vi "Main_Marvin Remake.vi"() -> ()   [LabVIEW 2017]
uses:
  PCAN_Driver/ControlCAN.llb/DevType.ctl
  PCAN_Driver/ControlCAN.llb/CAN Channel.ctl
  PCAN_Driver/ControlCAN.llb/VCI_INIT_CONFIG.ctl
  PCAN_Driver/ControlCAN.llb/InitFlag.ctl
  PCAN_Driver/ControlCAN.llb/Fliter.ctl
  PCAN_Driver/ControlCAN.llb/Mode.ctl
  <vilib>/Utility/miscctls.llb/LVRowAndColumnTypeDef.ctl
  <vilib>/Utility/config.llb/Read Key (String).vi
  <vilib>/Utility/config.llb/Write Key (String).vi
  <vilib>/Utility/cursorutil.llb/Set Cursor (Icon Pict).vi
  PCAN_Driver/ControlCAN.lvlib
  <vilib>/Utility/config.llb/NI_LVConfig.lvlib
panel:
  in  "AD Resistor Step":dbl=9.0 format="%#_13g"
  out "ClosePanel":bool=TRUE
  out "UUT SN Report":string
  out "Automation":bool
  out "Test Failed":bool
  out "AuxiOFFResult":bool
  out "AuxiONResult":bool
  out "SensCalResult":bool
  out "VisualInspectionResult":bool
  out "BurnResult":bool
  out "BurnSpeed":bool
  out "BurnTemp":bool
  out "BurnDC":bool
  out "TempControlResult":bool
  out "MotorTempResult":bool
  out "StopTimeResult":bool
  out "SpeedResult":bool=TRUE
  out "VenableDirectionResult":bool
  out "VenableResult":bool
  out "ComTestResult":bool=TRUE
  out "UUT SoftwareVer":string
  out "Next SN":i32
  in  "SetSN":bool
  out "Current SN":i32
  out "Cal":dbl
  out "AO[1]Meas":dbl
  out "FullSpeed2 Speed":dbl
  out "FullSpeed2 Current":dbl
  out "FullSpeed1 Current":dbl
  out "FullSpeed1 Speed":dbl
  out "MaxBurnInTempVal":dbl
  in  "Stop Burn-in":bool
  out "VISA Tester":refnum<visa-resource-name>
  out "UUT":u8
  out "CAN Status":bool
  in  "Channel 2":T1 caption="Channel" items=["Channel 1", "Channel 2"]
  out "Config_CANAT":T7 {"DevType" items=["USB-CAN"=3, "USB-CAN2"=4]; "CanIndex" items=["通道1", "通道2"]; "VCI_INIT_CONFIG"."Fliter" items=["接收所有类型"=3, "只接收标准帧"=4, "只接收扩展帧"=7]; "VCI_INIT_CONFIG"."Mode" items=["正常工作", "自测模式（环回）", "仅侦听模式"]; "VCI_INIT_CONFIG"."InitFlag" items=["使用Flash参数", "使用界面设置参数"]}
  out "Array":u64[][](array[numeric]) format="%016x"
  out "Motor Phase Current RMS":dbl
  out "Ambient Temperature":dbl
  out "Speed error":bool
  out "Commutation err":bool
  out "Under voltage/Over voltage":bool
  out "Derated drive temp":bool
  out "Motor Over temperature":bool
  out "Motor Sensor temp Fauilre":bool
  out "Drive Over temperature":bool
  out "Drive Sensor temp Failure":bool
  out "Ambient Over temp":bool
  out "Ambient Sensor temp":bool
  out "DC Voltage":dbl
  out "DC Current":dbl
  out "Power transistor Heat sink Temp.":dbl
  out "Motor Stator Temp.":dbl
  out "Motor Speed RPM":dbl
  out "ECS State":u16
  out "UUT":string="EBAY"
  in  "Logger Path":path
  in  "Report":bool
  in  "Start":bool
  in  "ATR":string[][](table)=[["Test Communication", "-", "-", "-", "-", ""], ["Set S/N", "-", "-", "-", "-", ""], ["Set Board Number", "-", "-", "-", "-", ""], [" ", "", "", "", "", ""], ["Test Communication", "-", "-", "-", "-", ""], ["Get S/N", "-", "-", "-", "", ""], ["Get Board Number", "-", "-", "-", "", ""], ["Get FW", "-", "-", "-", "", ""], ["Enable Motor", "", "", "", "", ""], ["Small position command", "", "", "", "", ""], ["Measure delta", "", "", "", "", ""], ["Velocity command", "", "", "", "", ""]]
  in  "Settings":bool
  in  "Refresh Button":bool
  out "Status":bool
  in  "VISA Marvin":refnum<visa-resource-name>="COM6"
  in  "Serial Com":bool
  in  "Help Button":bool
  out "Pannel User Message":string
  in  "Stop Button":bool
  # "Marvin"
  # "REDLER TECHNOLOGIES LTD"
  # "ver 1.2n"
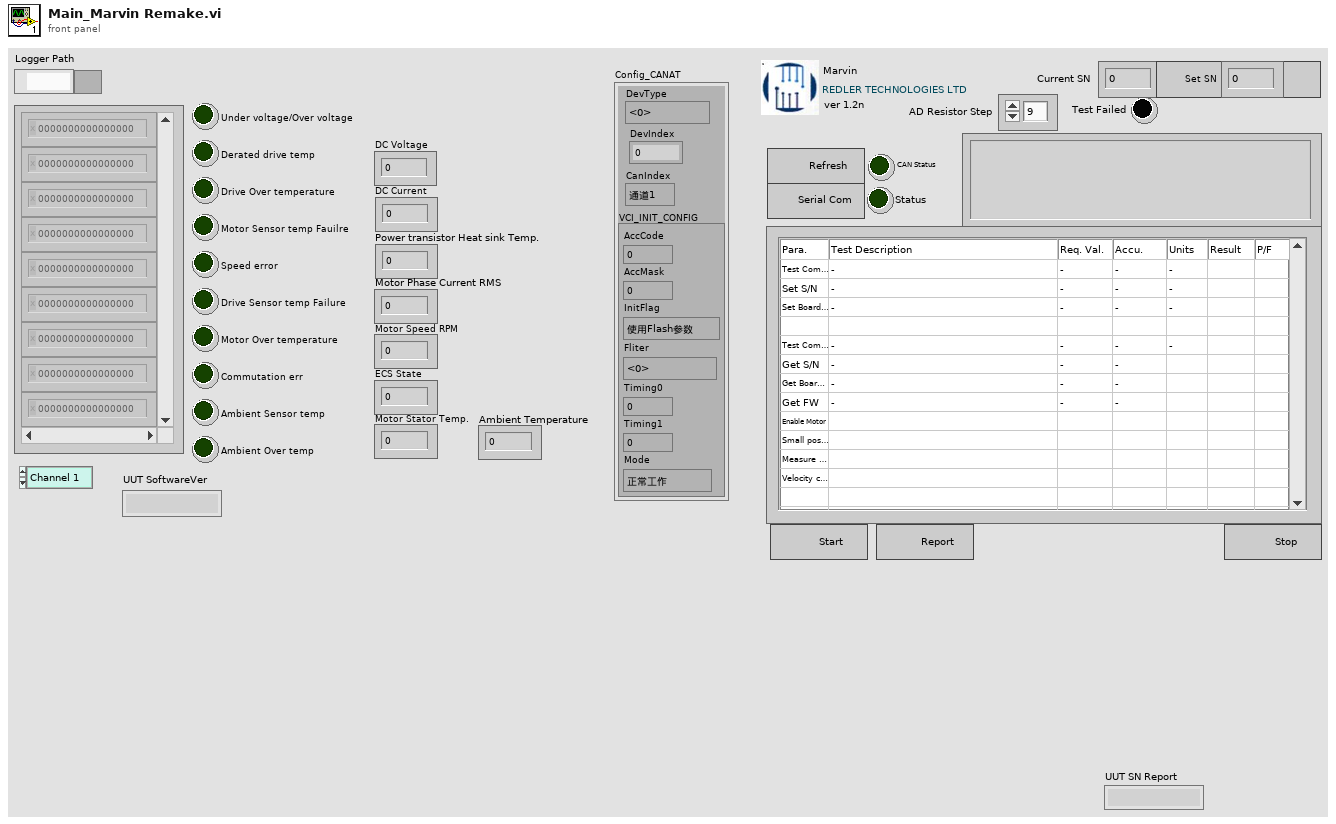
[diagram p1: front panel]
types:
  T1 = typedef "ControlCAN.lvlib/CAN Channel.ctl" = u32
  T2 = typedef "ControlCAN.lvlib/DevType.ctl" = u32
  T3 = typedef "ControlCAN.lvlib/VCI_INIT_CONFIG.ctl" = cluster{"AccCode":u32, "AccMask":u32, "InitFlag":T4, "Fliter":T5, "Timing0":u8, "Timing1":u8, "Mode":T6}
  T4 = typedef "ControlCAN.lvlib/InitFlag.ctl" = u32
  T5 = typedef "ControlCAN.lvlib/Fliter.ctl" = u8
  T6 = typedef "ControlCAN.lvlib/Mode.ctl" = u8
  T7 = cluster{"DevType":T2, "DevIndex":u32, "CanIndex":T1, "VCI_INIT_CONFIG":T3}
  T8 = cluster{"VISA":refnum<visa-resource-name>, "Array Test":enum16{"Auxiliary", "Temp Sens Cal", "Com Test", "Enable Test", "Speed Command", "Stop Time", "Temp Control", "Burn in", "Visual Inspec", "Empty"}[]}
  T9 = cluster{"ID":u32, "MSGTYPE":u8, "LEN":u8, "aDATA":u8[]}[]
  T10 = enum16{"Erase ATR Table", "Stop", "MainProgram", "Initialize"}
  T11 = enum16{"K15", "K16", "K17", "Venable", "Firmeware", "Fan", "Power", "120C", "110C", "100C", "90C", "80C", "70C", "60C", "50C", "40C", "30C", "25C", "20C", "10C", "0C"}
  T12 = enum16{"Stop", "Result", "FullSpeed2", "MD[1]=1", "FullSpeed1", "MD[1]=0"}
  T13 = enum8{"Term1", "Term2", "Current", "Fan", "TempCPU"}
  T14 = enum16{"Stop", "AO[1]=Meas.", "TA[5]", "AO[1]=0", "Start"}
  T15 = enum16{"Stop", "BurnIn", "Ambient Temp", "MotorSpeed", "DC Current Measure", "Start"}
  T16 = enum16{"Auxiliary", "Temp Sens Cal", "Com Test", "Enable Test", "Speed Command", "Stop Time", "Temp Control", "Burn in", "Visual Inspec", "Empty"}[]
  T17 = enum16{"K15", "K16", "K17", "Venable", "Firmeware", "Fan", "Power", "120C", "110C", "100C", "90C", "80C", "70C", "60C", "50C", "40C", "30C", "25C", "20C", "10C", "0C"}[]
  T18 = enum32{"6000", "11500", "15100", "11500-2", "6000-2"}[]
  T19 = enum8{"Enabled", "Disabled", "Disabled and Grayed Out"}
  T20 = typedef "LVRowAndColumnTypeDef.ctl" = cluster{"Row":i32, "Column":i32}
  T21 = enum32{"Invalid", "Standard", "Closed", "Hidden", "Minimized", "Maximized"}
  T22 = cluster{"ID":u32, "MSGTYPE":u8, "LEN":u8, "aDATA":u8[]}
  T23 = enum16{"Auxiliary", "Temp Sens Cal", "Com Test", "Enable Test", "Speed Command", "Stop Time", "Temp Control", "Burn in", "Visual Inspec", "Empty"}
  T24 = enum16{"open", "replace", "create", "open or create", "replace or create", "replace or create with confirmation"}
  T25 = typedef "NI_LVConfig.lvlib/Config Data RefNum.ctl" = refnum<k1>
  T26 = typedef "ControlCAN.lvlib/VCI_CAN_OBJ.ctl" = cluster{"ID":u32, "TimeStamp":u32, "TimeFlag":u8, "SendType":u8, "RemoteFlag":u8, "ExternFlag":u8, "DataLen":u8, "Data":u8[], "Reserved":u8[]}
  T27 = cluster{"Type":enum16{"接收", "发送"}, "Channel":T1, "Time":timestamp, "VCI_CAN_OBJ":T26}[]
  T28 = cluster{"Type":enum16{"接收", "发送"}, "Channel":T1, "Time":timestamp, "VCI_CAN_OBJ":T26}
  T29 = typedef "LVPoint32TypeDef.ctl" = cluster{"Horizontal":i32, "Vertical":i32}
  T30 = enum8{"Term1", "Term2", "Current", "Fan", "TempCPU"}[]
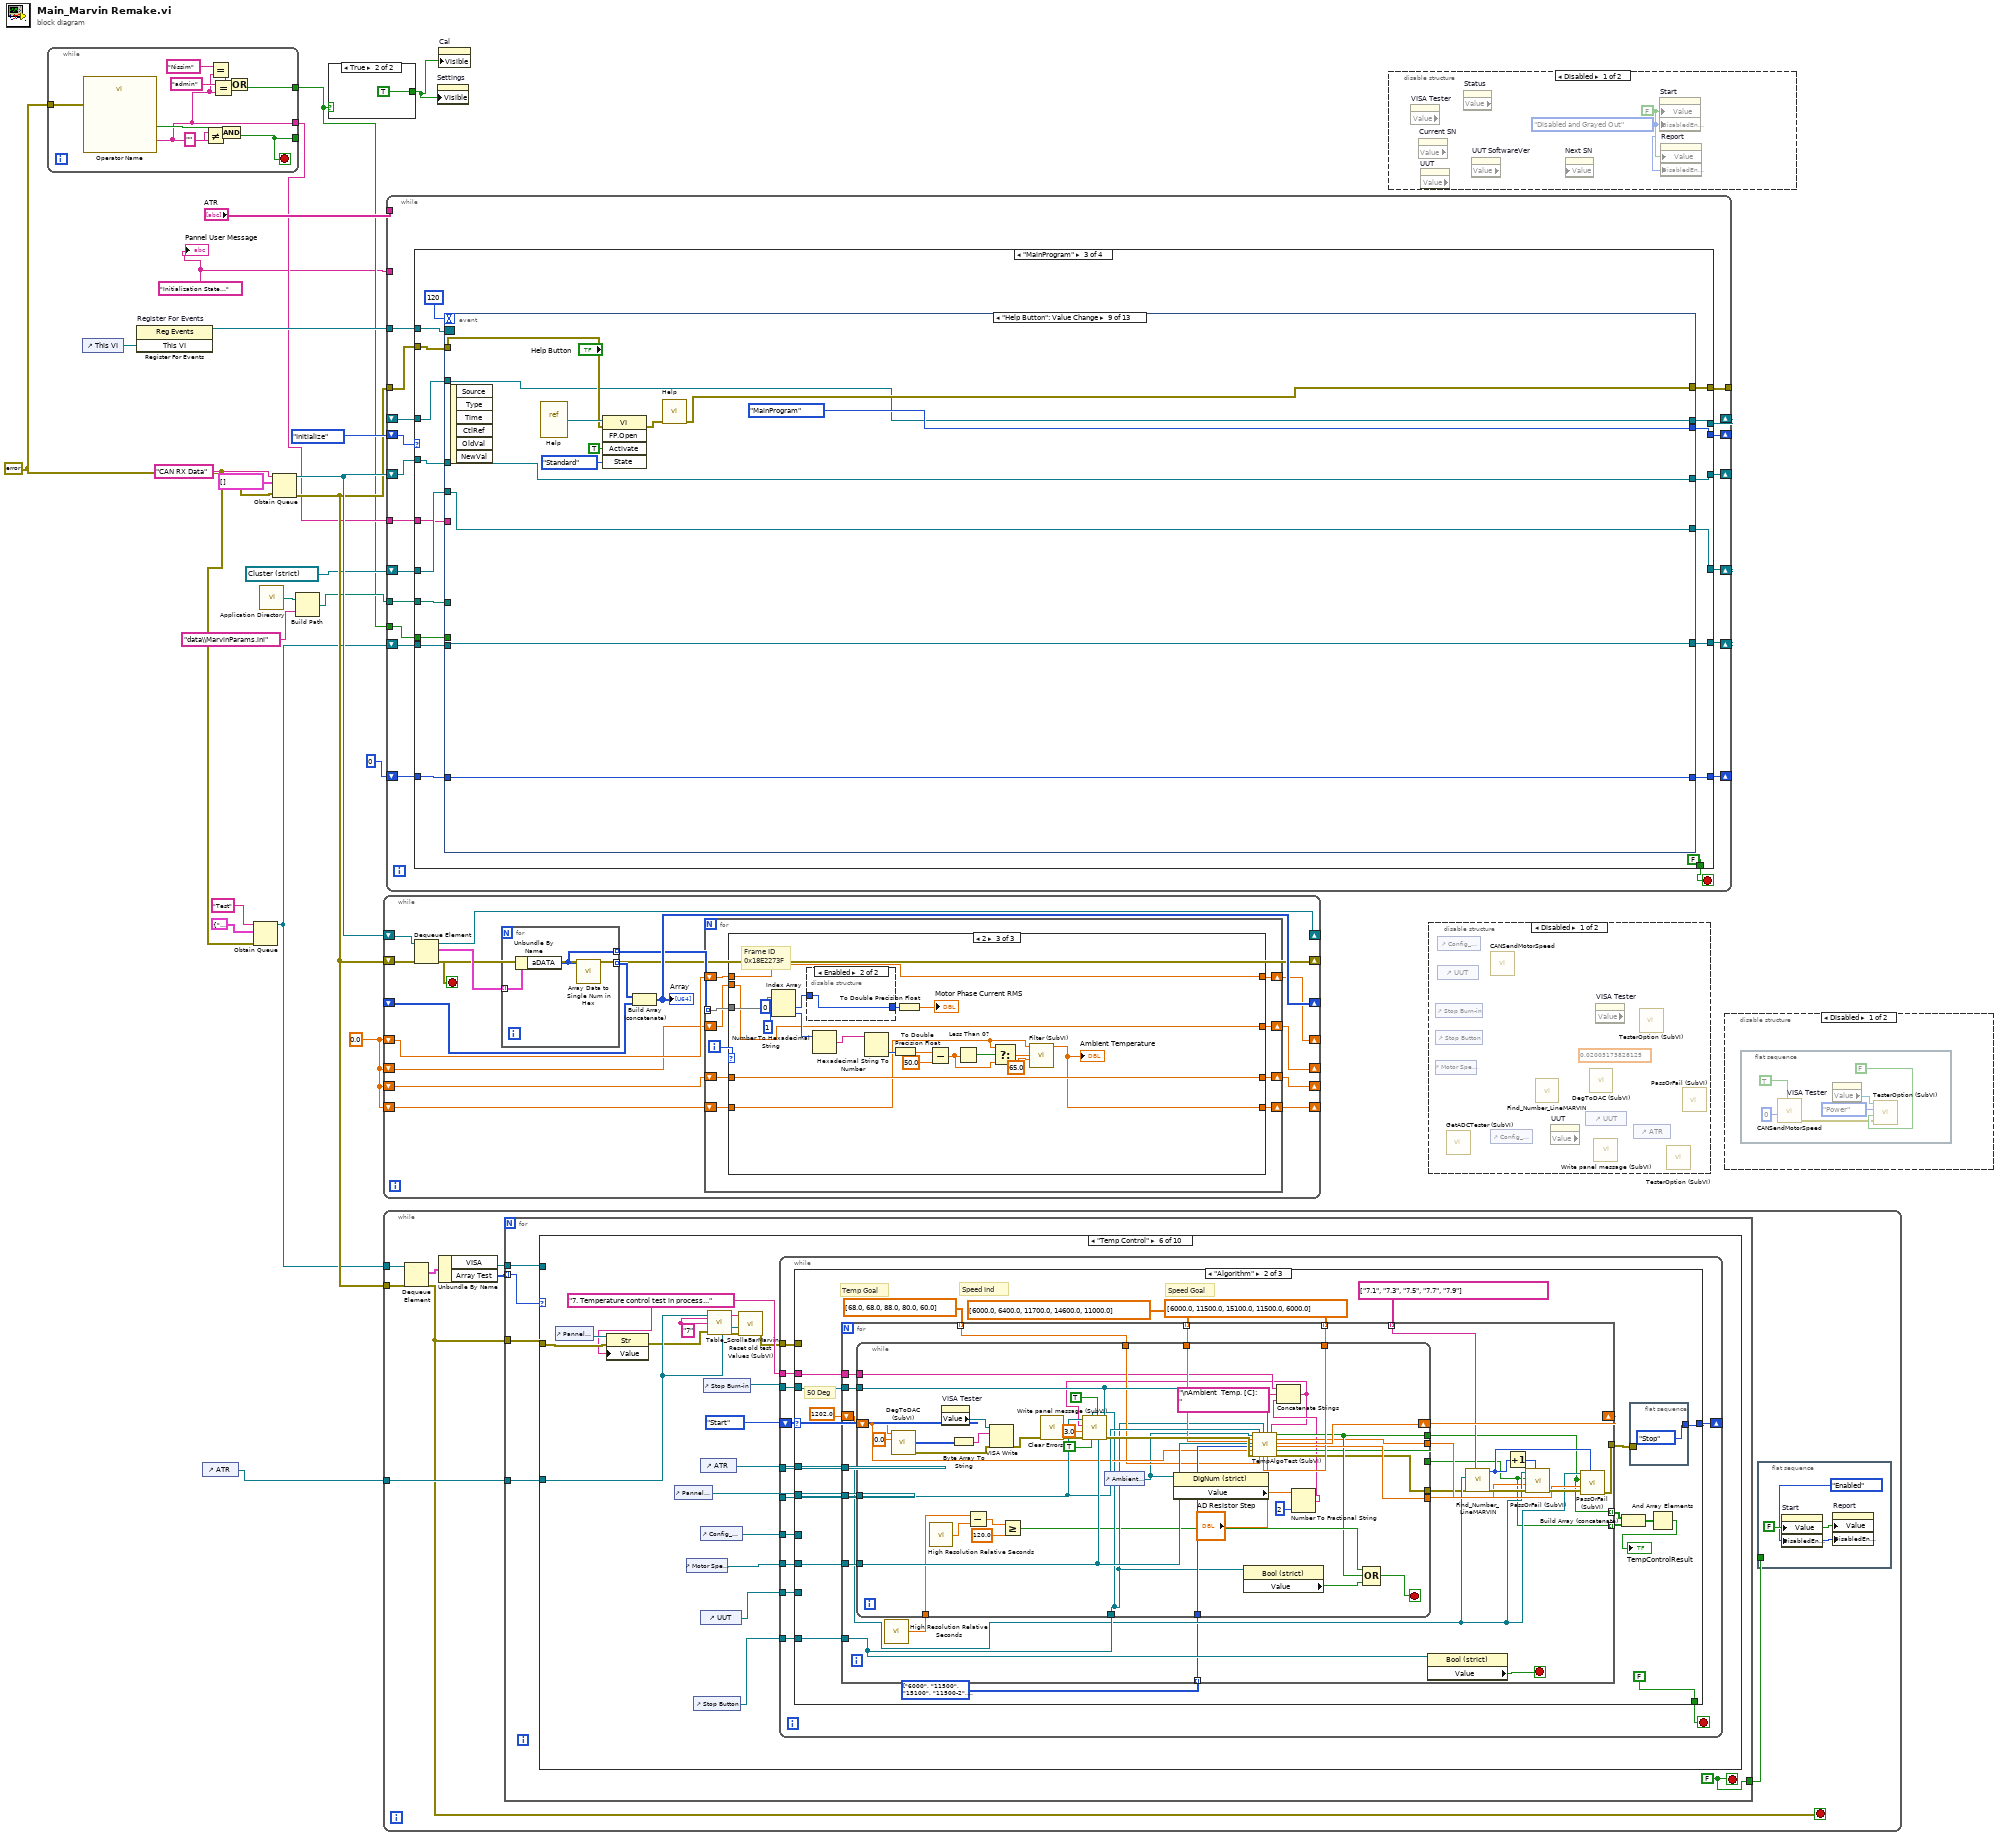
[diagram p0: block diagram]
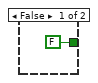
[diagram p2: hidden frame]
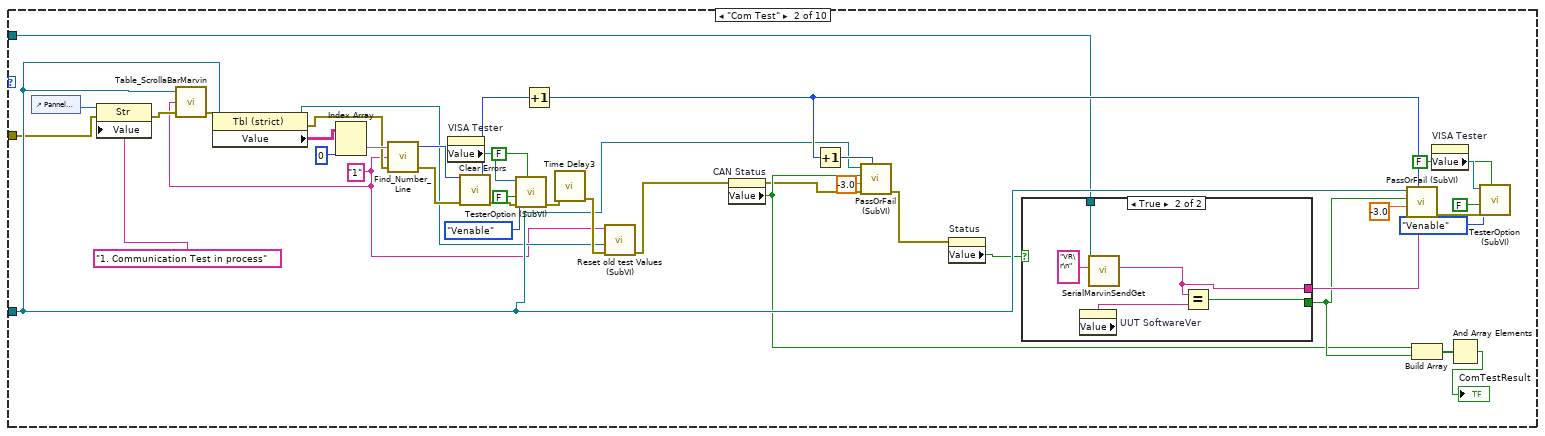
[diagram p7: hidden frame]
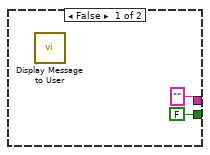
[diagram p8: hidden frame]
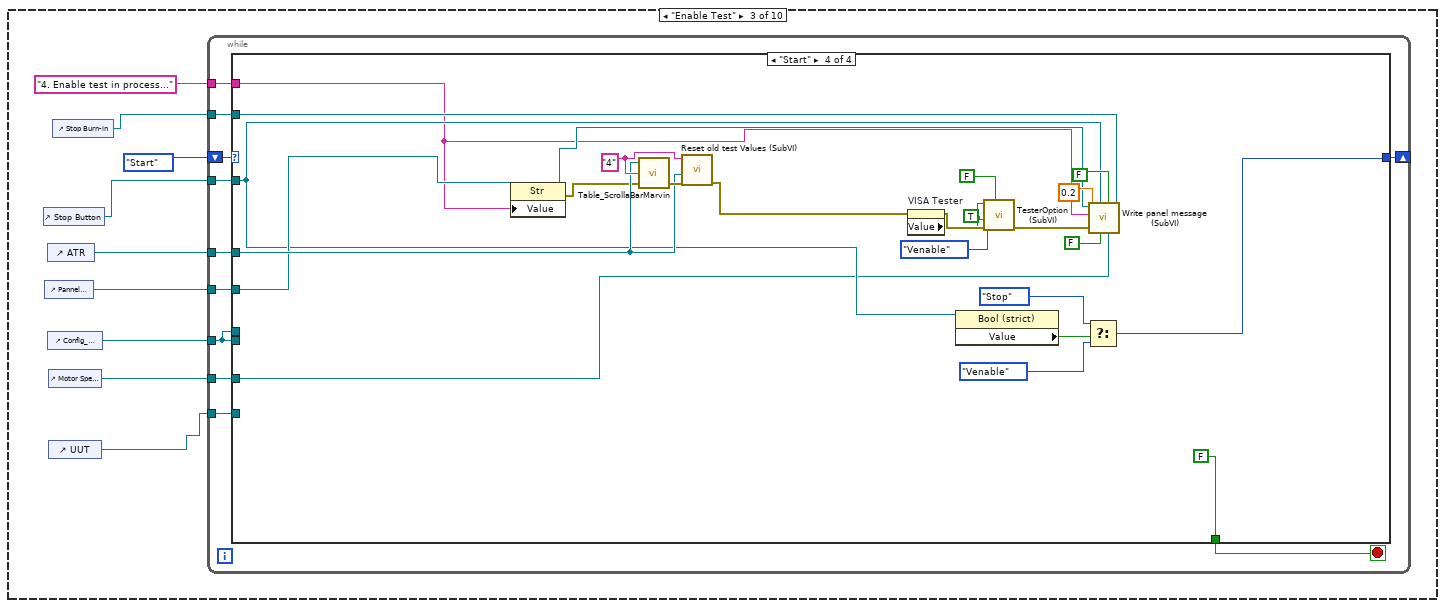
[diagram p9: hidden frame]
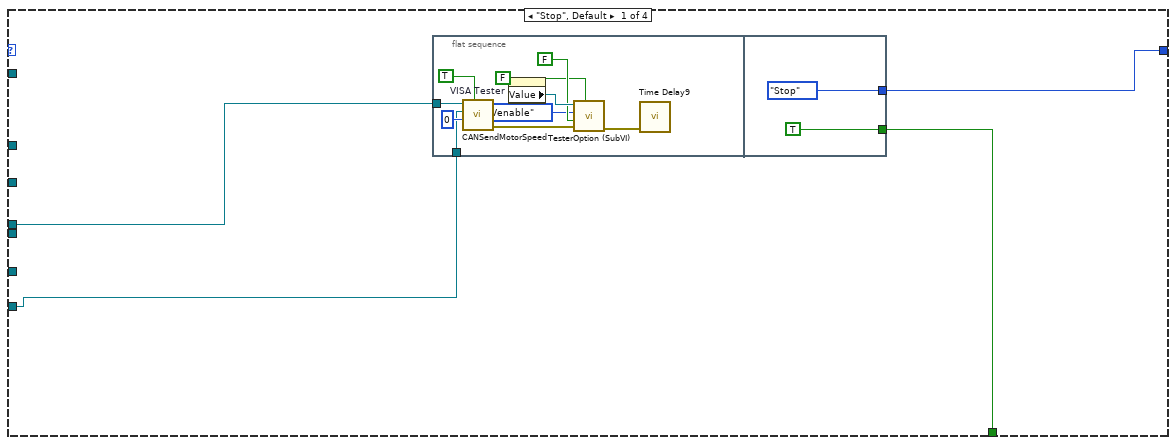
[diagram p10: hidden frame]
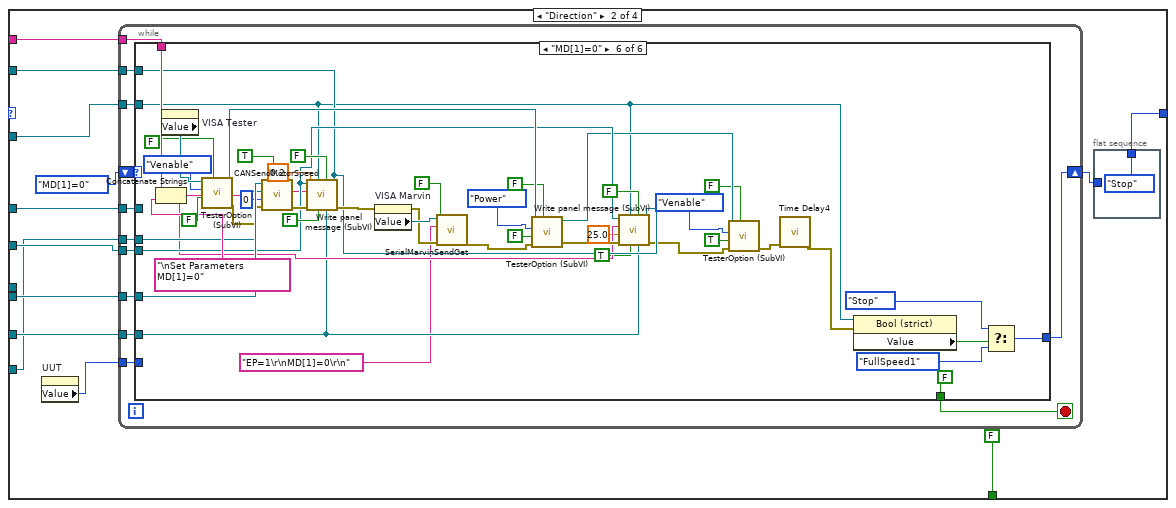
[diagram p11: hidden frame]
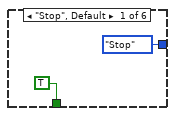
[diagram p12: hidden frame]
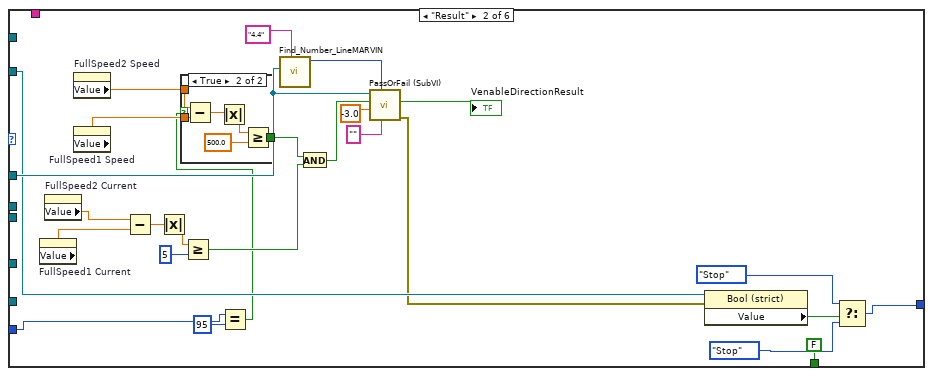
[diagram p13: hidden frame]
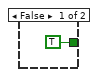
[diagram p14: hidden frame]
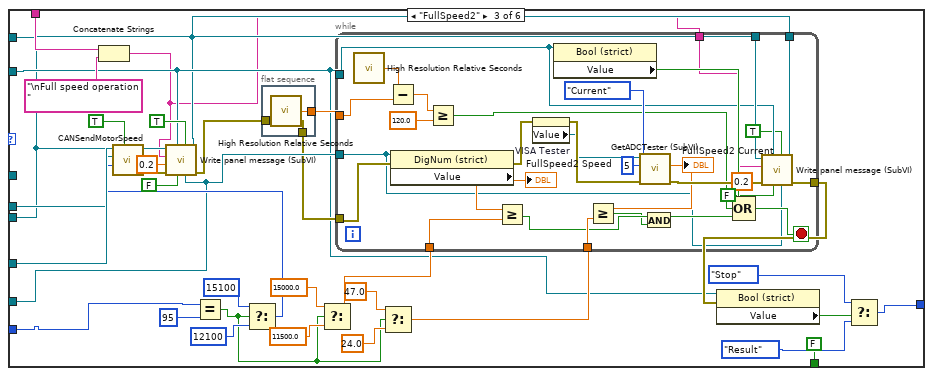
[diagram p15: hidden frame]
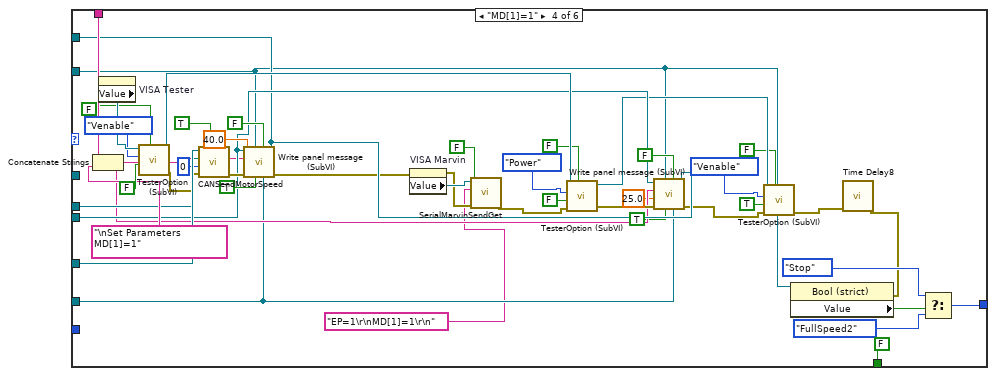
[diagram p16: hidden frame]
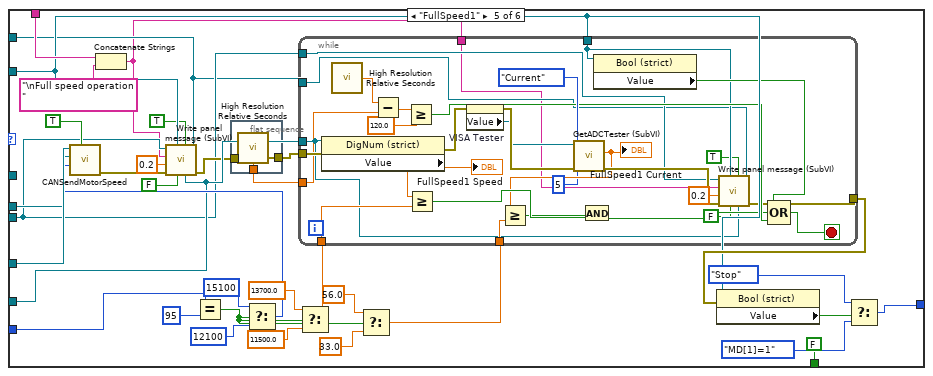
[diagram p17: hidden frame]
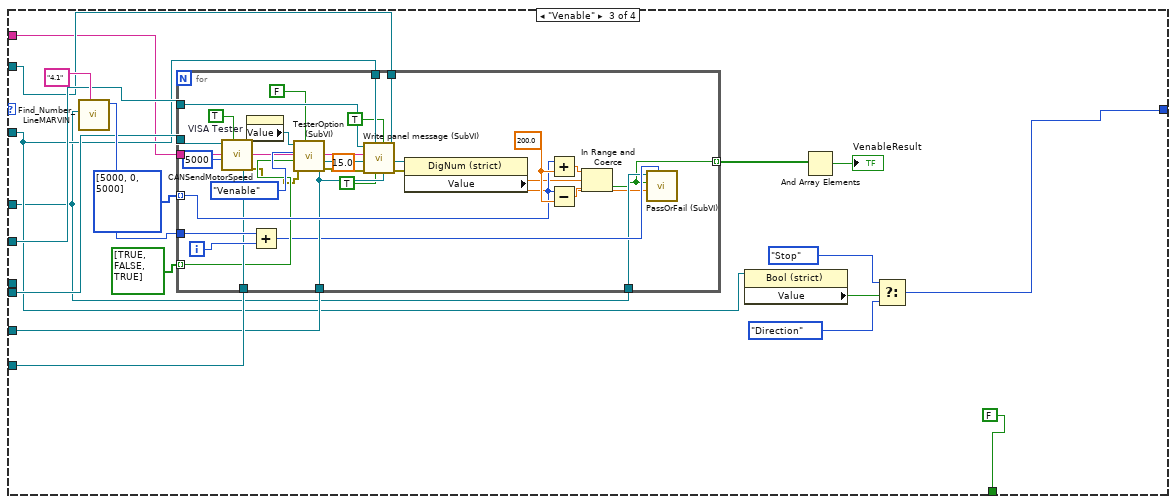
[diagram p18: hidden frame]
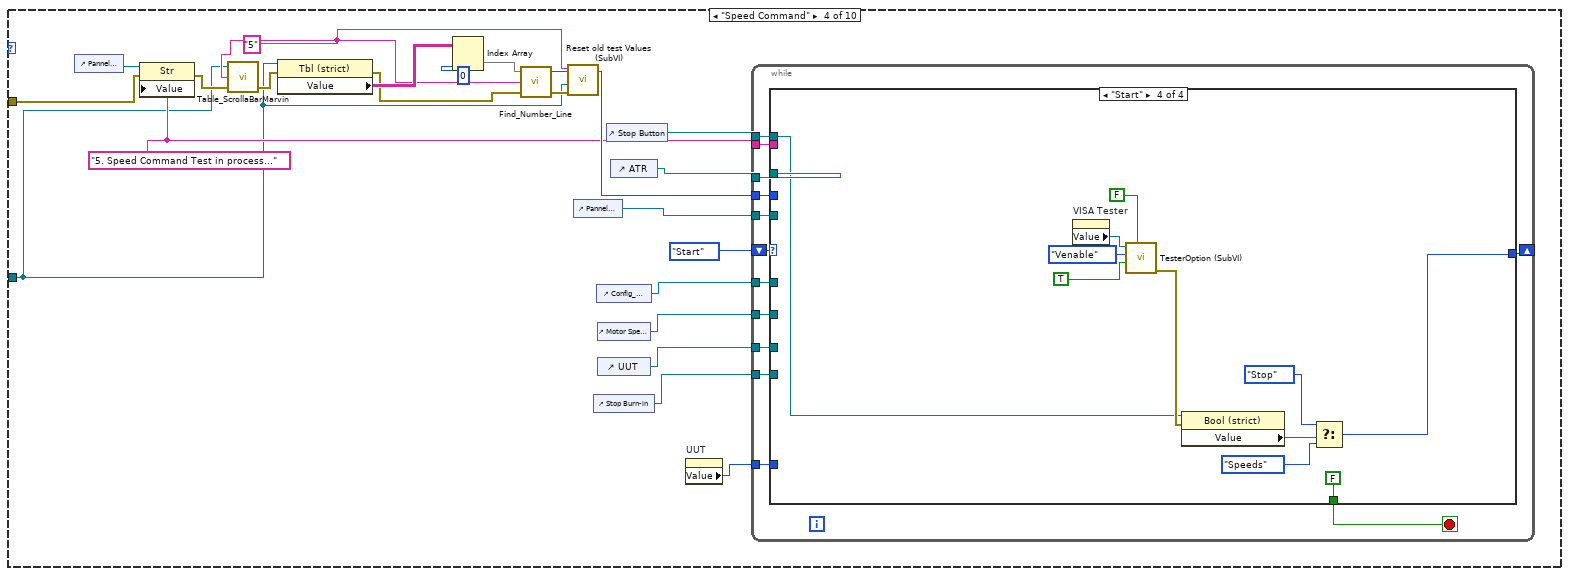
[diagram p19: hidden frame]
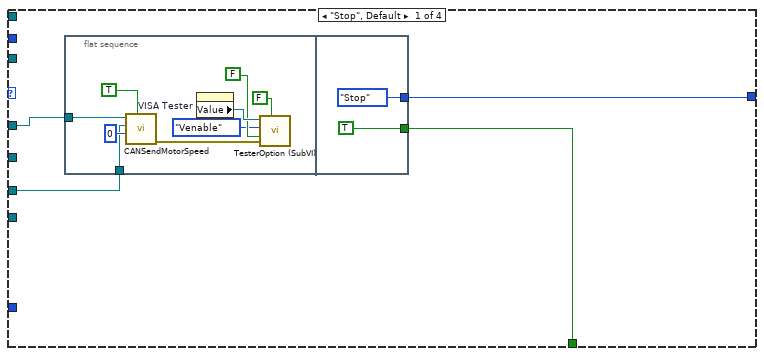
[diagram p20: hidden frame]
diagram:
  w2 = "Initialization State..."
  w13 = 0.0
  w12 = errorcluster {"status"=FALSE, "code"=0, "source"=""} ("error in (no error)")
  n1 = while {
    tunnel: [w31] -> _
    tunnel: [w27] -> w7
    tunnel: [w28] -> w3
    tunnel: w12 -> [w24]
    stop <- w31 stop-if-true
    n2 = call "Operator Name"("error in (no error)"=w24) -> ("Operator Name"=w27:string, "OK"=w32:bool)  [unwired: 16 in, 1 out]
    n3 = Not Equal?(x=w27, y="") -> (x != y?=w33:bool)
    n4 = Equal?(x="Nissim", y=w27) -> (x = y?=w25:bool)
    n5 = Equal?(x="admin", y=w27) -> (x = y?=w29:bool)
    n6 = And(x=w32, y=w33) -> (x .and. y?=w31:bool)
    n7 = Or(x=w25, y=w29) -> (x .or. y?=w28:bool)
  }
  n8 = control-ref of="This VI"() -> (w9:refnum<vi>)
  n9 = register-events "Register For Events"(w9) -> (reference out=w8:refnum<event-registration>)  [unwired: 2 in, 1 out]
  n10 = control-ref of="ATR"() -> (w1:refnum<vi>)
  n11 = Obtain Queue(name (unnamed)="Test", element data type=T8 {"VISA"="COM1", "Array Test"=[]}, error in (no error)=w12) -> (queue out=w17:refnum<queue>)  [unwired: 2 in, 2 out]
  n12 = call <vilib>:"Application Directory.vi"() -> ("Application Directory"=w11:path)
  n13 = Obtain Queue(name (unnamed)="CAN RX Data", element data type=T9 [], error in (no error)=w12) -> (queue out=w20:refnum<queue>, error out=w18:errorcluster)  [unwired: 2 in, 1 out]
  n14 = Build Path(base path=w11, name or relative path="data\\MarvinParams.ini") -> (appended path=w5:path)
  n15 = case shown="True" w3 {
    tunnel: [FALSE TRUE] -> w4
    frame False {
    }
    frame True {
    }
  }
  n16 = while {
    shift-right: [w51] -> _
    shift-left: w20 -> [w53]
    shift-right: [w49] -> _
    shift-left: _ -> [w50]
    shift-right: [w45] -> _
    shift-left: w18 -> [w45]
    shift-right: [w43] -> _
    shift-left: w13 -> [w44]
    shift-right: [w42] -> _
    shift-left: w13 -> [w41]
    shift-right: [w40] -> _
    shift-left: w13 -> [w39]
    shift-right: [w38] -> _
    shift-left: w13 -> [w37]
    stop <- w52 stop-if-true
    n17 = Dequeue Element(queue=w53, error in (no error)=w45) -> (queue out=w51:refnum<queue>, element=w46:T9, error out=w52:errorcluster)  [unwired: 1 in, 1 out]
    n18 = for {
      tunnel: [w182] -> w48 mode=indexing
      tunnel: w46 -> [w181] mode=indexing
      tunnel: [w180] -> w47 mode=indexing
      n19 = Unbundle By Name(w181) -> ("aDATA"=w180:u8[])
      n20 = call "Array Data to Single Num in Hex.vi"("aDATA"=w180) -> ("Numeric"=w182:u64)  [unwired: 10 in]
    }
    n21 = Build Array (concatenate)(w48, w50) -> (w49:u64[][])
    "Array" <- w49
    n22 = for {
      tunnel: w47 -> [w63] mode=indexing
      shift-right: [w60] -> w43
      shift-left: w44 -> [w61]
      shift-right: [w59] -> w42
      shift-left: w41 -> [w58]
      shift-right: [w57] -> w40
      shift-left: w39 -> [w56]
      shift-right: [w55] -> w38
      shift-left: w37 -> [w54]
      i -> [w62]
      n23 = case shown="2" w62 {
        tunnel: w63 -> [w103 w136 w175]
        tunnel: w61 -> [w77 w125 w164]
        tunnel: [w75 w125 w164] -> w60
        tunnel: [w72 w124 w163] -> w59
        tunnel: w58 -> [w71 w124 w163]
        tunnel: [w66 w123 w162] -> w57
        tunnel: w56 -> [w65 w123 w162]
        tunnel: [w64 w122 w157] -> w55
        tunnel: w54 -> [w64 w122 w156]
        frame 0, Default {
          # "Frame ID\n0x18E1273F"
          n24 = Index Array(array=w103, index #1=0 ("index"), index #2=1 ("index"), index #3=2 ("index"), index #4=3 ("index"), index #5=4 ("index"), index #6=5 ("index"), index #7=6 ("index"), index #8=7 ("index")) -> (element #1=w87:u8, element #2=w89:u8, element #3=w90:u8, element #4=w94:u8, element #5=w97:u8, element #6=w101:u8, element #7=w102:u8, element #8=w100:u8)
          n25 = Number To Hexadecimal String(2:w100) -> (0:w114:string)  [unwired: 1 in]
          n26 = Join Numbers(hi=w102, lo=w101) -> ((hi.lo)=w121:u16)
          n27 = Join Numbers(hi=w90, lo=w89) -> ((hi.lo)=w91:u16)
          n28 = Number To Hexadecimal String(2:w97) -> (0:w98:string)  [unwired: 1 in]
          n29 = Number To Hexadecimal String(2:w121) -> (0:w120:string)  [unwired: 1 in]
          n30 = Number To Hexadecimal String(2:w87) -> (0:w88:string)  [unwired: 1 in]
          n31 = Number To Hexadecimal String(2:w91) -> (0:w92:string)  [unwired: 1 in]
          n32 = Number To Hexadecimal String(2:w94) -> (0:w95:string)  [unwired: 1 in]
          n33 = Hexadecimal String To Number(string=w114) -> (number=w113:u32)  [unwired: 2 in, 1 out]
          n34 = To Double Precision Float(number=w113) -> (double precision float=→"DC Current":dbl)
          n35 = Hexadecimal String To Number(string=w98) -> (number=w99:u32)  [unwired: 2 in, 1 out]
          n36 = Hexadecimal String To Number(string=w120) -> (number=w119:u32)  [unwired: 2 in, 1 out]
          n37 = Hexadecimal String To Number(string=w88) -> (number=w85:u32)  [unwired: 2 in, 1 out]
          n38 = Hexadecimal String To Number(string=w92) -> (number=w93:u32)  [unwired: 2 in, 1 out]
          n39 = Hexadecimal String To Number(string=w95) -> (number=w96:u32)  [unwired: 2 in, 1 out]
          n40 = To Double Precision Float(number=u32 10 ("y")) -> (double precision float=w117:dbl)
          n41 = To Double Precision Float(number=w119) -> (double precision float=w116:dbl)
          n42 = To Double Precision Float(number=w99) -> (double precision float=w82:dbl)
          n43 = To Double Precision Float(number=w93) -> (double precision float=w78:dbl)
          n44 = To Double Precision Float(number=w96) -> (double precision float=w84:dbl)
          n45 = Divide(x=w116, y=w117) -> (x/y=→"DC Voltage":dbl)
          n46 = To Unsigned Word Integer(number=w85) -> (unsigned 16bit integer=→"ECS State":u16)
          n47 = Subtract(x=w82, y=50.0 ("x")) -> (x-y=w70:dbl)
          n48 = Subtract(x=w84, y=50.0 ("x")) -> (x-y=w73:dbl)
          n49 = call "Filter (SubVI).vi"("Delta"=5000.0, "NewVal"=w78, "OldVal"=w77) -> ("Val"=w75:dbl)  [unwired: 8 in]
          "Motor Speed RPM" <- w75
          n50 = Less Than 0?(x=w73) -> (x < 0?=w80:bool)
          n51 = Less Than 0?(x=w70) -> (x < 0?=w79:bool)
          n52 = Select(t=w71, s=w80, f=w73) -> (s? t:f=w74:dbl)
          n53 = Select(t=w65, s=w79, f=w70) -> (s? t:f=w69:dbl)
          n54 = call "Filter (SubVI).vi"("Delta"=130.0, "NewVal"=w74, "OldVal"=w71) -> ("Val"=w72:dbl)  [unwired: 8 in]
          "Motor Stator Temp." <- w72
          n55 = call "Filter (SubVI).vi"("Delta"=100.0, "NewVal"=w69, "OldVal"=w65) -> ("Val"=w66:dbl)  [unwired: 8 in]
          "Power transistor Heat sink Temp." <- w66
        }
        frame 1 {
          # "Framde ID\n0x18E3273F"
          n56 = control-ref of="UUT"() -> (w126:refnum<vi>)
          n57 = property on="Property Node" class="DigNum (strict)"(reference=w126) -> ("Value"=w127:u8)  [unwired: 1 in, 2 out]
          n58 = Index Array(array=w136, index #1=0 ("index"), index #2=1 ("index")) -> (element #1=w134:u8, element #2=w129:u8)
          n59 = Number To Boolean Array(number=w134) -> (Boolean array=w133:bool[])
          n60 = Number To Boolean Array(number=w129) -> (Boolean array=w131:bool[])
          n61 = Boolean To (0,1)(Boolean=w131) -> (0, 1=w128:i16[])
          n62 = Boolean To (0,1)(Boolean=w133) -> (0, 1=w132:i16[])
          n63 = case shown="95" w127 {
            tunnel: w128 -> [_ w137]
            frame 0, Default {
            }
            frame 95 {
              n64 = for {
                tunnel: w137 -> [w142] mode=indexing
                i -> [w138]
                stop <- w140 stop-if-true
                n65 = Not Equal To 0?(x=w142) -> (x != 0?=w141:bool)
                n66 = case shown="0, Default" w138 {
                  tunnel: w141 -> [w143 w144]
                  frame 0, Default {
                    "Ambient Sensor temp" <- w143
                  }
                  frame 1 {
                    "Ambient Over temp" <- w144
                  }
                }
                n67 = Equal?(x=w138, y=1.0) -> (x = y?=w140:bool)
              }
            }
          }
          n68 = for {
            tunnel: w132 -> [w146] mode=indexing
            i -> [w147]
            n69 = Not Equal To 0?(x=w146) -> (x != 0?=w145:bool)
            n70 = case shown="1" w147 {
              tunnel: w145 -> [w148 w149 w150 w151 w152 w153 w154 w155]
              frame 0, Default {
                "Drive Sensor temp Failure" <- w148
              }
              frame 1 {
                "Drive Over temperature" <- w149
              }
              frame 2 {
                "Motor Sensor temp Fauilre" <- w150
              }
              frame 3 {
                "Motor Over temperature" <- w151
              }
              frame 4 {
                "Derated drive temp" <- w152
              }
              frame 5 {
                "Under voltage/Over voltage" <- w153
              }
              frame 6 {
                "Commutation err" <- w154
              }
              frame 7 {
                "Speed error" <- w155
              }
            }
          }
        }
        frame 2 {
          # "Frame ID\n0x18E2273F"
          n71 = Index Array(array=w175, index #1=0 ("index"), index #2=1 ("index")) -> (element #1=w172:u8, element #2=w169:u8)
          n72 = disable-structure shown="Enabled" {
            disable-tunnel: [w178 w179] -> w173
            disable-tunnel: w172 -> [w177 w179]
            frame Disabled {
              n73 = Number To Hexadecimal String(2:w177) -> (0:w176:string)  [unwired: 1 in]
              n74 = Hexadecimal String To Number(string=w176) -> (number=w178:u32)  [unwired: 2 in, 1 out]
            }
            frame Enabled {
            }
          }
          n75 = Number To Hexadecimal String(2:w169) -> (0:w167:string)  [unwired: 1 in]
          n76 = Hexadecimal String To Number(string=w167) -> (number=w168:u32)  [unwired: 2 in, 1 out]
          n77 = To Double Precision Float(number=w168) -> (double precision float=w166:dbl)
          n78 = To Double Precision Float(number=w173) -> (double precision float=→"Motor Phase Current RMS":dbl)
          n79 = Subtract(x=w166, y=50.0) -> (x-y=w160:dbl)
          n80 = Less Than 0?(x=w160) -> (x < 0?=w161:bool)
          n81 = Select(t=w156, s=w161, f=w160) -> (s? t:f=w159:dbl)
          n82 = call "Filter (SubVI).vi"("Delta"=65.0, "NewVal"=w159, "OldVal"=w156) -> ("Val"=w157:dbl)  [unwired: 8 in]
          "Ambient Temperature" <- w157
        }
      }
    }
  }
  n83 = while {
    tunnel: w1 -> [w190]
    tunnel: w18 -> [w188]
    tunnel: w17 -> [w189]
    stop <- w184 stop-if-true
    n84 = Dequeue Element(queue=w189, error in (no error)=w188) -> (element=w187:T8, error out=w184:errorcluster)  [unwired: 1 in, 2 out]
    n85 = Unbundle By Name(w187) -> ("VISA"=w186:refnum<visa-resource-name>, "Array Test"=w185:T16)
    n86 = for {
      tunnel: w185 -> [w194] mode=indexing
      tunnel: w186 -> [w197]
      tunnel: w190 -> [w196]
      tunnel: w184 -> [w195]
      tunnel: [w193] -> w183
      stop <- w193 stop-if-true
      w193 = FALSE
      n87 = case shown="\"Temp Control\"" w194 {
        tunnel: w197 -> [_ w221 _ _ w805 _ _ _ w1362 _]
        tunnel: w196 -> [_ w228 _ w640 w801 w964 _ w1348 w1369 w1581]
        tunnel: w195 -> [_ w225 _ w655 w811 w962 _ w1347 w1367 w1580]
        frame "Empty", Default {
        }
        frame "Com Test" {
          w204 = "1" ("Test Paragraph")
          n88 = control-ref of="Pannel User Message"() -> (w226:refnum<vi>)
          n89 = property class="Str"(reference=w226, error in=w225, "Value"="1. Communication Test in process") -> (error out=w224:errorcluster)  [unwired: 1 out]
          n90 = call "Table_ScrollaBarMarvin.vi"("error in"=w224, "Line to focus"=w204, "reference in"=w228) -> ("error out"=w227:errorcluster)  [unwired: 2 out]
          n91 = property class="Tbl (strict)"(reference=w228, error in=w227) -> (reference out=w205:refnum<vi>, error out=w235:errorcluster, "Value"=w236:string[][])
          n92 = Index Array(array=w236, index (col)=0 ("disabled index (col)")) -> (element=w237:string[])  [unwired: 1 in]
          n93 = call "Find_Number_Line.vi"("error in"=w235, "Test Paragraph"=w204, "Row Headers[]"=w237) -> ("error out"=w233:errorcluster, "Line number"=w232:i32)  [unwired: 1 out]
          n94 = property on="VISA Tester" class="VISAName"() -> ("Value"=w215:refnum<visa-resource-name>)  [unwired: 2 in, 2 out]
          n95 = call <vilib>:"Clear Errors.vi"("error in (no error)"=w233) -> ("error out"=w217:errorcluster)  [unwired: 5 in, 1 out]
          n96 = call "TesterOption (SubVI).vi"("2 Options"=FALSE, "error in (no error)"=w217, "On/Off"=FALSE, "Tester Option"=T11."Venable", "VISA Refnum in"=w215) -> ("error out"=w216:errorcluster)  [unwired: 5 in, 1 out]
          n97 = Increment(x=w232) -> (x+1=w231:i32)
          n98 = call "Time Delay3"("error in (no error)"=w216) -> ("error out"=w229:errorcluster)  [unwired: 10 in]
          n99 = call "Reset old test Values (SubVI).vi"("error in"=w229, "Atr in"=w205, "Test Paragraph"=w204) -> ("error out"=w199:errorcluster)  [unwired: 8 in]
          n100 = property on="CAN Status" class="Bool (strict)"(error in=w199) -> (error out=w198:errorcluster, "Value"=w200:bool)  [unwired: 1 in, 1 out]
          n101 = Increment(x=w231) -> (x+1=w230:i32)
          n102 = call "PassOrFail (SubVI).vi"("index (row)"=w230, "error in (no error)"=w198, "Data in"=-3.0, "Pass?Fail"=w200, "Table in"=w228) -> ("error out"=w220:errorcluster)  [unwired: 6 in]
          n103 = property on="Status" class="Bool (strict)"(error in=w220) -> ("Value"=w222:bool)  [unwired: 1 in, 2 out]
          n104 = case shown="True" w222 {
            tunnel: w221 -> [_ w244]
            tunnel: [FALSE w241] -> w202
            tunnel: ["" ("read buffer") w240] -> w219
            frame False {
              n105 = call "Display Message to User"() -> ()  [unwired: 10 in, 2 out]
            }
            frame True {
              n106 = property on="UUT SoftwareVer" class="Str"() -> ("Value"=w242:string)  [unwired: 2 in, 2 out]
              n107 = call "SerialMarvinSendGet.vi"("write buffer"="VR\r\n", "VISA resource name"=w244) -> ("read buffer"=w240:string)  [unwired: 8 in, 1 out]
              n108 = Equal?(x=w240, y=w242) -> (x = y?=w241:bool)
            }
          }
          n109 = call "PassOrFail (SubVI).vi"("String Res"=w219, "index (row)"=w231, "Data in"=-3.0, "Pass?Fail"=w202, "Table in"=w228) -> ("error out"=w211:errorcluster)  [unwired: 6 in]
          n110 = Build Array(w200, w202) -> (w203:bool[])
          n111 = property on="VISA Tester" class="VISAName"() -> ("Value"=w210:refnum<visa-resource-name>)  [unwired: 2 in, 2 out]
          n112 = And Array Elements(Boolean array=w203) -> (logical AND=→"ComTestResult":bool)
          n113 = call "TesterOption (SubVI).vi"("2 Options"=FALSE, "error in (no error)"=w211, "On/Off"=FALSE, "Tester Option"=T11."Venable", "VISA Refnum in"=w210) -> ()  [unwired: 5 in, 2 out]
        }
        frame "Enable Test" {
          n114 = control-ref of="Stop Button"() -> (w247:refnum<vi>)
          n115 = control-ref of="Pannel User Message"() -> (w249:refnum<vi>)
          n116 = control-ref of="ATR"() -> (w248:refnum<vi>)
          n117 = control-ref of="Config_CANAT"() -> (w250:refnum<vi>)
          n118 = control-ref of="Motor Speed RPM"() -> (w251:refnum<vi>)
          n119 = control-ref of="UUT"() -> (w252:refnum<vi>)
          n120 = control-ref of="Stop Burn-in"() -> (w253:refnum<vi>)
          n121 = while {
            shift-right: [w258] -> _
            shift-left: enum16{"Stop", "Direction", "Venable", "Start"}."Start" -> [w264]
            tunnel: w247 -> [w263]
            tunnel: w248 -> [w262]
            tunnel: w249 -> [w261]
            tunnel: w250 -> [w254]
            tunnel: w251 -> [w260]
            tunnel: w252 -> [w255]
            tunnel: w253 -> [w257]
            tunnel: "4. Enable test in process..." ("Strin") -> [w256]
            stop <- w259 stop-if-true
            n122 = case shown="\"Start\"" w264 {
              tunnel: w263 -> [_ w291 w572 w619]
              tunnel: w262 -> [_ w286 w570 w626]
              tunnel: w261 -> [_ w289 w574 w625]
              tunnel: w254 -> [_ w292 w577 _]
              tunnel: w260 -> [_ w288 w575 w617]
              tunnel: w255 -> [w265 w282 w576 _]
              tunnel: [w268 FALSE FALSE FALSE] -> w259
              tunnel: [w266 w285 w571 w623] -> w258
              tunnel: w257 -> [_ w290 w573 w618]
              tunnel: w256 -> [_ w287 w569 w616]
              tunnel: w254 -> [w267 _ _ _]
              frame "Stop", Default {
                n123 = flat-sequence {
                  tunnel: w265 -> [w274]
                  tunnel: w267 -> [w273]
                  tunnel: [TRUE] -> w268
                  tunnel: [enum16{"Stop", "Direction", "Venable", "Start"}."Stop"] -> w266
                  frame #0 {
                    n124 = call "CANSendMotorSpeed.vi"("Remote"=TRUE, "Motor Speed RPM"=u16 0, "UUT"=w274, "CAN Cluster in"=w273) -> ("error out"=w277:errorcluster)  [unwired: 7 in]
                    n125 = property on="VISA Tester" class="VISAName"() -> ("Value"=w278:refnum<visa-resource-name>)  [unwired: 2 in, 2 out]
                    n126 = call "TesterOption (SubVI).vi"("2 Options"=FALSE, "error in (no error)"=w277, "On/Off"=FALSE, "Tester Option"=T11."Venable", "VISA Refnum in"=w278) -> ("error out"=w269:errorcluster)  [unwired: 5 in, 1 out]
                    n127 = call "Time Delay9"("error in (no error)"=w269) -> ()  [unwired: 10 in, 1 out]
                  }
                  frame #1 {
                  }
                }
              }
              frame "Direction" {
                n128 = property on="UUT" class="DigNum (strict)"() -> ("Value"=w281:u8)  [unwired: 2 in, 2 out]
                n129 = while {
                  shift-right: [w305] -> w284
                  shift-left: T12."MD[1]=0" -> [w306]
                  tunnel: w292 -> [w303]
                  tunnel: w282 -> [w302]
                  tunnel: w291 -> [w301]
                  tunnel: w290 -> [w300]
                  tunnel: w289 -> [w299]
                  tunnel: w288 -> [w298]
                  tunnel: w287 -> [w297]
                  tunnel: w286 -> [w296]
                  tunnel: w281 -> [w295]
                  stop <- w304 stop-if-true
                  n130 = case shown="\"MD[1]=0\"" w306 {
                    tunnel: [T12."Stop" w330 w372 w452 w485 w565] -> w305
                    tunnel: [TRUE FALSE FALSE FALSE FALSE FALSE] -> w304
                    tunnel: w303 -> [_ _ w370 w446 w483 w559]
                    tunnel: w302 -> [_ _ w366 w425 w479 w537]
                    tunnel: w301 -> [_ w317 w345 w416 w461 w527]
                    tunnel: w300 -> [_ _ w343 w426 w459 w538]
                    tunnel: w299 -> [_ _ w344 w427 w460 w539]
                    tunnel: w298 -> [_ _ w361 w414 w475 w533]
                    tunnel: w297 -> [_ _ w356 w435 w473 w547]
                    tunnel: w296 -> [_ w321 _ _ _ _]
                    tunnel: w295 -> [_ w309 w341 _ w454 _]
                    frame "Stop", Default {
                    }
                    frame "Result" {
                      n131 = property on="FullSpeed1 Current" class="DigNum (strict)"() -> ("Value"=w325:dbl)  [unwired: 2 in, 2 out]
                      n132 = property on="FullSpeed2 Current" class="DigNum (strict)"() -> ("Value"=w326:dbl)  [unwired: 2 in, 2 out]
                      n133 = property on="FullSpeed2 Speed" class="DigNum (strict)"() -> ("Value"=w328:dbl)  [unwired: 2 in, 2 out]
                      n134 = property on="FullSpeed1 Speed" class="DigNum (strict)"() -> ("Value"=w327:dbl)  [unwired: 2 in, 2 out]
                      n135 = Subtract(x=w326, y=w325) -> (x-y=w324:dbl)
                      n136 = Absolute Value(x=w324) -> (abs(x)=w313:dbl)
                      n137 = Greater Or Equal?(x=w313, y=u32 5) -> (x >= y?=w319:bool)
                      n138 = Equal?(x=w309, y=u8 95) -> (x = y?=w311:bool)
                      n139 = case shown="True" w311 {
                        tunnel: w328 -> [_ w339]
                        tunnel: w327 -> [_ w338]
                        tunnel: [TRUE w335] -> w320
                        frame False {
                        }
                        frame True {
                          n140 = Subtract(x=w339, y=w338) -> (x-y=w340:dbl)
                          n141 = Absolute Value(x=w340) -> (abs(x)=w337:dbl)
                          n142 = Greater Or Equal?(x=w337, y=500.0) -> (x >= y?=w335:bool)
                        }
                      }
                      n143 = call "Find_Number_LineMARVIN.vi"("Test Paragraph"="4.4", "TableIn"=w321) -> ("Line number"=w318:i32)  [unwired: 3 in, 3 out]
                      n144 = And(x=w320, y=w319) -> (x .and. y?=w310:bool)
                      "VenableDirectionResult" <- w310
                      n145 = call "PassOrFail (SubVI).vi"("String Res"="", "index (row)"=w318, "Data in"=-3.0, "Pass?Fail"=w310, "Table in"=w321) -> ("error out"=w316:errorcluster)  [unwired: 6 in]
                      n146 = property class="Bool (strict)"(reference=w317, error in=w316) -> ("Value"=w333:bool)  [unwired: 2 out]
                      n147 = Select(t=T12."Stop", s=w333, f=T12."Stop") -> (s? t:f=w330:T12)
                    }
                    frame "FullSpeed2" {
                      n148 = Concatenate Strings(w356, "\nFull speed operation " ("string")) -> (w342:string)
                      n149 = Equal?(x=w341, y=u8 95) -> (x = y?=w351:bool)
                      n150 = Select(t=u16 15100, s=w351, f=u16 12100 ("y")) -> (s? t:f=w365:u16)
                      n151 = call "CANSendMotorSpeed.vi"("Remote"=TRUE, "Motor Speed RPM"=w365, "UUT"=w366, "CAN Cluster in"=w370) -> ("error out"=w363:errorcluster)  [unwired: 7 in]
                      n152 = call "Write panel message (SubVI).vi"("Stop BurnIn"=w343, 4:"rpm"=w361, 5:"rpm"=TRUE ("rpm"), "PrintTime"=FALSE, "Stop"=w345, "error in (no error)"=w363, "Time to wait"=0.2, "Strin"=w342, "String in"=w344) -> ("error out"=w348:errorcluster)  [unwired: 2 in]
                      n153 = flat-sequence {
                        tunnel: w348 -> [w377]
                        tunnel: [w377] -> w347
                        tunnel: [w376] -> w346
                        frame #0 {
                          n154 = call <vilib>:"High Resolution Relative Seconds.vi"() -> ("relative seconds"=w376:dbl)
                        }
                      }
                      n155 = Select(t=15000.0, s=w351, f=11500.0) -> (s? t:f=w350:dbl)
                      n156 = Select(t=47.0, s=w351, f=24.0) -> (s? t:f=w349:dbl)
                      n157 = while {
                        tunnel: w361 -> [w379]
                        tunnel: w347 -> [w407]
                        tunnel: [w387] -> w358
                        tunnel: w350 -> [w400]
                        tunnel: w349 -> [w399]
                        tunnel: w346 -> [w395]
                        tunnel: w345 -> [w385]
                        tunnel: w344 -> [w386]
                        tunnel: w343 -> [w383]
                        tunnel: w342 -> [w382]
                        stop <- w397 stop-if-true
                        n158 = call <vilib>:"High Resolution Relative Seconds.vi"() -> ("relative seconds"=w396:dbl)
                        n159 = Subtract(x=w396, y=w395) -> (x-y=w394:dbl)
                        n160 = property class="DigNum (strict)"(reference=w379, error in=w407) -> (error out=w406:errorcluster, "Value"=w401:dbl)  [unwired: 1 out]
                        "FullSpeed2 Speed" <- w401
                        n161 = Greater Or Equal?(x=w394, y=120.0) -> (x >= y?=w392:bool)
                        n162 = Greater Or Equal?(x=w401, y=w400) -> (x >= y?=w391:bool)
                        n163 = property on="VISA Tester" class="VISAName"(error in=w406) -> (error out=w405:errorcluster, "Value"=w404:refnum<visa-resource-name>)  [unwired: 1 in, 1 out]
                        n164 = property class="Bool (strict)"(reference=w385) -> ("Value"=w390:bool)  [unwired: 1 in, 2 out]
                        n165 = call "GetADCTester (SubVI).vi"("error in (no error)"=w405, "GetADCTester"=T13."Current", "TimeToGet"=5, "VISA Refnum in"=w404) -> ("error out"=w402:errorcluster, "ADCValOutput Single"=w398:dbl)  [unwired: 5 in, 1 out]
                        "FullSpeed2 Current" <- w398
                        n166 = Greater Or Equal?(x=w398, y=w399) -> (x >= y?=w388:bool)
                        n167 = And(x=w391, y=w388) -> (x .and. y?=w389:bool)
                        n168 = Compound Arithmetic op=OR(w390, w392, w389) -> (w397:bool)
                        n169 = call "Write panel message (SubVI).vi"("Stop BurnIn"=w383, 4:"rpm"=w379, 5:"rpm"=TRUE ("rpm"), "PrintTime"=FALSE, "Stop"=w385, "error in (no error)"=w402, "Time to wait"=0.2, "Strin"=w382, "String in"=w386) -> ("error out"=w387:errorcluster)  [unwired: 2 in]
                      }
                      n170 = property class="Bool (strict)"(reference=w345, error in=w358) -> ("Value"=w375:bool)  [unwired: 2 out]
                      n171 = Select(t=T12."Stop", s=w375, f=T12."Result") -> (s? t:f=w372:T12)
                    }
                    frame "MD[1]=1" {
                      n172 = Concatenate Strings(w435, "\nSet Parameters MD[1]=1" ("Strin")) -> (w424:string)
                      n173 = property on="VISA Tester" class="VISAName"() -> ("Value"=w440:refnum<visa-resource-name>)  [unwired: 2 in, 2 out]
                      n174 = call "TesterOption (SubVI).vi"("2 Options"=FALSE, "On/Off"=FALSE, "Tester Option"=T11."Venable", "VISA Refnum in"=w440) -> ("error out"=w441:errorcluster, "VISA Refnum out"=w431:refnum<visa-resource-name>)  [unwired: 6 in]
                      n175 = call "CANSendMotorSpeed.vi"("Remote"=TRUE, "error in (no error)"=w441, "Motor Speed RPM"=u16 0, "UUT"=w425, "CAN Cluster in"=w446) -> ("error out"=w443:errorcluster)  [unwired: 6 in]
                      n176 = call "Write panel message (SubVI).vi"("Stop BurnIn"=w426, 4:"rpm"=w414, 5:"rpm"=FALSE ("rpm"), "PrintTime"=TRUE, "Stop"=w416, "error in (no error)"=w443, "Time to wait"=40.0, "Strin"=w424, "String in"=w427) -> ("error out"=w413:errorcluster)  [unwired: 2 in]
                      n177 = property on="VISA Marvin" class="VISAName"(error in=w413) -> (error out=w442:errorcluster, "Value"=w448:refnum<visa-resource-name>)  [unwired: 1 in, 1 out]
                      n178 = call "SerialMarvinSendGet.vi"("error in (no error)"=w442, "Clear Log"=FALSE, "write buffer"="EP=1\r\nMD[1]=1\r\n", "VISA resource name"=w448) -> ("error out"=w430:errorcluster)  [unwired: 6 in, 1 out]
                      n179 = call "TesterOption (SubVI).vi"("2 Options"=FALSE, "error in (no error)"=w430, "On/Off"=FALSE, "Tester Option"=T11."Power", "VISA Refnum in"=w431) -> ("error out"=w428:errorcluster, "VISA Refnum out"=w417:refnum<visa-resource-name>)  [unwired: 5 in]
                      n180 = call "Write panel message (SubVI).vi"("Stop BurnIn"=w426, 4:"rpm"=w414, 5:"rpm"=FALSE ("rpm"), "PrintTime"=TRUE, "Stop"=w416, "error in (no error)"=w428, "Time to wait"=25.0, "Strin"=w424, "String in"=w427) -> ("error out"=w418:errorcluster)  [unwired: 2 in]
                      n181 = call "TesterOption (SubVI).vi"("2 Options"=FALSE, "error in (no error)"=w418, "On/Off"=TRUE, "Tester Option"=T11."Venable", "VISA Refnum in"=w417) -> ("error out"=w415:errorcluster)  [unwired: 5 in, 1 out]
                      n182 = call "Time Delay8"("error in (no error)"=w415) -> ("error out"=w411:errorcluster)  [unwired: 10 in]
                      n183 = property class="Bool (strict)"(reference=w416, error in=w411) -> ("Value"=w453:bool)  [unwired: 2 out]
                      n184 = Select(t=T12."Stop", s=w453, f=T12."FullSpeed2") -> (s? t:f=w452:T12)
                    }
                    frame "FullSpeed1" {
                      n185 = Concatenate Strings(w473, "\nFull speed operation " ("string")) -> (w458:string)
                      n186 = Equal?(x=w454, y=u8 95) -> (x = y?=w471:bool)
                      n187 = flat-sequence {
                        tunnel: w464 -> [w490]
                        tunnel: [w490] -> w463
                        tunnel: [w489] -> w462
                        frame #0 {
                          n188 = call <vilib>:"High Resolution Relative Seconds.vi"() -> ("relative seconds"=w489:dbl)
                        }
                      }
                      n189 = Select(t=u16 15100, s=w471, f=u16 12100 ("y")) -> (s? t:f=w478:u16)
                      n190 = call "CANSendMotorSpeed.vi"("Remote"=TRUE, "Motor Speed RPM"=w478, "UUT"=w479, "CAN Cluster in"=w483) -> ("error out"=w476:errorcluster)  [unwired: 7 in]
                      n191 = call "Write panel message (SubVI).vi"("Stop BurnIn"=w459, 4:"rpm"=w475, 5:"rpm"=TRUE ("rpm"), "PrintTime"=FALSE, "Stop"=w461, "error in (no error)"=w476, "Time to wait"=0.2, "Strin"=w458, "String in"=w460) -> ("error out"=w464:errorcluster)  [unwired: 2 in]
                      n192 = Select(t=13700.0, s=w471, f=11500.0) -> (s? t:f=w466:dbl)
                      n193 = Select(t=56.0, s=w471, f=33.0) -> (s? t:f=w465:dbl)
                      n194 = while {
                        tunnel: w475 -> [w492]
                        tunnel: w463 -> [w520]
                        tunnel: [w500] -> w474
                        tunnel: w466 -> [w512]
                        tunnel: w465 -> [w509]
                        tunnel: w462 -> [w507]
                        tunnel: w461 -> [w498]
                        tunnel: w460 -> [w499]
                        tunnel: w459 -> [w496]
                        tunnel: w458 -> [w495]
                        stop <- w514 stop-if-true
                        n195 = property class="DigNum (strict)"(reference=w492, error in=w520) -> (error out=w519:errorcluster, "Value"=w513:dbl)  [unwired: 1 out]
                        "FullSpeed1 Speed" <- w513
                        n196 = call <vilib>:"High Resolution Relative Seconds.vi"() -> ("relative seconds"=w508:dbl)
                        n197 = Subtract(x=w508, y=w507) -> (x-y=w506:dbl)
                        n198 = Greater Or Equal?(x=w506, y=120.0) -> (x >= y?=w504:bool)
                        n199 = Greater Or Equal?(x=w513, y=w512) -> (x >= y?=w511:bool)
                        n200 = property on="VISA Tester" class="VISAName"(error in=w519) -> (error out=w518:errorcluster, "Value"=w517:refnum<visa-resource-name>)  [unwired: 1 in, 1 out]
                        n201 = call "GetADCTester (SubVI).vi"("error in (no error)"=w518, "GetADCTester"=T13."Current", "TimeToGet"=5, "VISA Refnum in"=w517) -> ("error out"=w515:errorcluster, "ADCValOutput Single"=w510:dbl)  [unwired: 5 in, 1 out]
                        "FullSpeed1 Current" <- w510
                        n202 = Greater Or Equal?(x=w510, y=w509) -> (x >= y?=w501:bool)
                        n203 = And(x=w501, y=w511) -> (x .and. y?=w502:bool)
                        n204 = property class="Bool (strict)"(reference=w498) -> ("Value"=w503:bool)  [unwired: 1 in, 2 out]
                        n205 = call "Write panel message (SubVI).vi"("Stop BurnIn"=w496, 4:"rpm"=w492, 5:"rpm"=TRUE ("rpm"), "PrintTime"=FALSE, "Stop"=w498, "error in (no error)"=w515, "Time to wait"=0.2, "Strin"=w495, "String in"=w499) -> ("error out"=w500:errorcluster)  [unwired: 2 in]
                        n206 = Compound Arithmetic op=OR(w503, w502, w504) -> (w514:bool)
                      }
                      n207 = property class="Bool (strict)"(reference=w461, error in=w474) -> ("Value"=w488:bool)  [unwired: 2 out]
                      n208 = Select(t=T12."Stop", s=w488, f=T12."MD[1]=1") -> (s? t:f=w485:T12)
                    }
                    frame "MD[1]=0" {
                      n209 = Concatenate Strings(w547, "\nSet Parameters MD[1]=0" ("Strin")) -> (w536:string)
                      n210 = property on="VISA Tester" class="VISAName"() -> ("Value"=w553:refnum<visa-resource-name>)  [unwired: 2 in, 2 out]
                      n211 = call "TesterOption (SubVI).vi"("2 Options"=FALSE, "On/Off"=FALSE, "Tester Option"=T11."Venable", "VISA Refnum in"=w553) -> ("error out"=w554:errorcluster, "VISA Refnum out"=w543:refnum<visa-resource-name>)  [unwired: 6 in]
                      n212 = call "CANSendMotorSpeed.vi"("Remote"=TRUE, "error in (no error)"=w554, "Motor Speed RPM"=u16 0, "UUT"=w537, "CAN Cluster in"=w559) -> ("error out"=w556:errorcluster)  [unwired: 6 in]
                      n213 = call "Write panel message (SubVI).vi"("Stop BurnIn"=w538, 4:"rpm"=w533, 5:"rpm"=FALSE ("rpm"), "PrintTime"=FALSE, "Stop"=w527, "error in (no error)"=w556, "Time to wait"=0.2, "Strin"=w536, "String in"=w539) -> ("error out"=w550:errorcluster)  [unwired: 2 in]
                      n214 = property on="VISA Marvin" class="VISAName"(error in=w550) -> (error out=w555:errorcluster, "Value"=w561:refnum<visa-resource-name>)  [unwired: 1 in, 1 out]
                      n215 = call "SerialMarvinSendGet.vi"("error in (no error)"=w555, "Clear Log"=FALSE, "write buffer"="EP=1\r\nMD[1]=0\r\n", "VISA resource name"=w561) -> ("error out"=w542:errorcluster)  [unwired: 6 in, 1 out]
                      n216 = call "TesterOption (SubVI).vi"("2 Options"=FALSE, "error in (no error)"=w542, "On/Off"=FALSE, "Tester Option"=T11."Power", "VISA Refnum in"=w543) -> ("error out"=w540:errorcluster, "VISA Refnum out"=w528:refnum<visa-resource-name>)  [unwired: 5 in]
                      n217 = call "Write panel message (SubVI).vi"("Stop BurnIn"=w538, 4:"rpm"=w533, 5:"rpm"=FALSE ("rpm"), "PrintTime"=TRUE, "Stop"=w527, "error in (no error)"=w540, "Time to wait"=25.0, "Strin"=w536, "String in"=w539) -> ("error out"=w529:errorcluster)  [unwired: 2 in]
                      n218 = call "TesterOption (SubVI).vi"("2 Options"=FALSE, "error in (no error)"=w529, "On/Off"=TRUE, "Tester Option"=T11."Venable", "VISA Refnum in"=w528) -> ("error out"=w526:errorcluster)  [unwired: 5 in, 1 out]
                      n219 = call "Time Delay4"("error in (no error)"=w526) -> ("error out"=w522:errorcluster)  [unwired: 10 in]
                      n220 = property class="Bool (strict)"(reference=w527, error in=w522) -> ("Value"=w566:bool)  [unwired: 2 out]
                      n221 = Select(t=T12."Stop", s=w566, f=T12."FullSpeed1") -> (s? t:f=w565:T12)
                    }
                  }
                }
                n222 = flat-sequence {
                  tunnel: [enum16{"Stop", "Direction", "Venable", "Start"}."Stop"] -> w285
                  tunnel: w284 -> [_]
                  frame #0 {
                  }
                }
              }
              frame "Venable" {
                n223 = call "Find_Number_LineMARVIN.vi"("Test Paragraph"="4.1", "TableIn"=w570) -> ("Line number"=w578:i32)  [unwired: 3 in, 3 out]
                n224 = for {
                  tunnel: u16[] [5000, 0, 5000] -> [w608] mode=indexing
                  tunnel: bool[] [TRUE, FALSE, TRUE] -> [w603] mode=indexing
                  tunnel: w578 -> [w609]
                  tunnel: w577 -> [w607]
                  tunnel: w576 -> [w606]
                  tunnel: w575 -> [w594]
                  tunnel: w574 -> [w598]
                  tunnel: w572 -> [w597]
                  tunnel: w573 -> [w596]
                  tunnel: w570 -> [w590]
                  tunnel: w569 -> [w588]
                  tunnel: [w587] -> w568 mode=indexing
                  i -> [w610]
                  w612 = 200.0 ("y")
                  n225 = call "CANSendMotorSpeed.vi"("Remote"=TRUE, "Motor Speed RPM"=u16 5000, "UUT"=w606, "CAN Cluster in"=w607) -> ("error out"=w602:errorcluster)  [unwired: 7 in]
                  n226 = property on="VISA Tester" class="VISAName"() -> ("Value"=w601:refnum<visa-resource-name>)  [unwired: 2 in, 2 out]
                  n227 = Add(x=w609, y=w610) -> (x+y=w591:i32)
                  n228 = call "TesterOption (SubVI).vi"("2 Options"=FALSE, "error in (no error)"=w602, "On/Off"=w603, "Tester Option"=T11."Venable", "VISA Refnum in"=w601) -> ("error out"=w600:errorcluster)  [unwired: 5 in, 1 out]
                  n229 = call "Write panel message (SubVI).vi"("Stop BurnIn"=w596, 4:"rpm"=w594, 5:"rpm"=TRUE ("rpm"), "PrintTime"=TRUE, "Stop"=w597, "error in (no error)"=w600, "Time to wait"=15.0, "Strin"=w588, "String in"=w598) -> ("error out"=w599:errorcluster)  [unwired: 2 in]
                  n230 = property class="DigNum (strict)"(reference=w594, error in=w599) -> ("Value"=w589:dbl)  [unwired: 2 out]
                  n231 = Add(x=w608, y=w612) -> (x+y=w614:dbl)
                  n232 = Subtract(x=w608, y=w612) -> (x-y=w613:dbl)
                  n233 = In Range and Coerce(upper limit=w614, x=w589, lower limit=w613) -> (In Range?=w587:bool)  [unwired: 1 out]
                  n234 = call "PassOrFail (SubVI).vi"("index (row)"=w591, "Data in"=w589, "Pass?Fail"=w587, "Table in"=w590) -> ()  [unwired: 7 in, 1 out]
                }
                n235 = property class="Bool (strict)"(reference=w572) -> ("Value"=w585:bool)  [unwired: 1 in, 2 out]
                n236 = And Array Elements(Boolean array=w568) -> (logical AND=→"VenableResult":bool)
                n237 = Select(t=enum16{"Stop", "Direction", "Venable", "Start"}."Stop", s=w585, f=enum16{"Stop", "Direction", "Venable", "Start"}."Direction") -> (s? t:f=w571:enum16{"Stop", "Direction", "Venable", "Start"})
              }
              frame "Start" {
                w634 = "4" ("Test Paragraph")
                n238 = property class="Str"(reference=w625, "Value"=w616) -> (reference out=w635:refnum<vi>, error out=w622:errorcluster)  [unwired: 1 in]
                n239 = call "Table_ScrollaBarMarvin.vi"("error in"=w622, "Line to focus"=w634, "reference in"=w626) -> ("error out"=w631:errorcluster)  [unwired: 2 out]
                n240 = call "Reset old test Values (SubVI).vi"("error in"=w631, "Atr in"=w626, "Test Paragraph"=w634) -> ("error out"=w630:errorcluster)  [unwired: 8 in]
                n241 = property on="VISA Tester" class="VISAName"(error in=w630) -> (error out=w629:errorcluster, "Value"=w628:refnum<visa-resource-name>)  [unwired: 1 in, 1 out]
                n242 = property class="Bool (strict)"(reference=w619) -> ("Value"=w639:bool)  [unwired: 1 in, 2 out]
                n243 = call "TesterOption (SubVI).vi"("2 Options"=FALSE, "error in (no error)"=w629, "On/Off"=TRUE, "Tester Option"=T11."Venable", "VISA Refnum in"=w628) -> ("error out"=w627:errorcluster)  [unwired: 5 in, 1 out]
                n244 = Select(t=enum16{"Stop", "Direction", "Venable", "Start"}."Stop", s=w639, f=enum16{"Stop", "Direction", "Venable", "Start"}."Venable") -> (s? t:f=w623:enum16{"Stop", "Direction", "Venable", "Start"})
                n245 = call "Write panel message (SubVI).vi"("Stop BurnIn"=w618, 4:"rpm"=w617, 5:"rpm"=FALSE ("rpm"), "PrintTime"=FALSE, "Stop"=w619, "error in (no error)"=w627, "Time to wait"=0.2, "Strin"=w616, "String in"=w635) -> ()  [unwired: 2 in, 1 out]
              }
            }
          }
        }
        frame "Speed Command" {
          w644 = "5. Speed Command Test in process..." ("Value")
          w641 = "5" ("Test Paragraph")
          n246 = control-ref of="Pannel User Message"() -> (w656:refnum<vi>)
          n247 = property class="Str"(reference=w656, error in=w655, "Value"=w644) -> (error out=w654:errorcluster)  [unwired: 1 out]
          n248 = call "Table_ScrollaBarMarvin.vi"("error in"=w654, "Line to focus"=w641, "reference in"=w640) -> ("error out"=w657:errorcluster)  [unwired: 2 out]
          n249 = property class="Tbl (strict)"(reference=w640, error in=w657) -> (error out=w659:errorcluster, "Value"=w660:string[][])  [unwired: 1 out]
          n250 = Index Array(array=w660, index (col)=0 ("disabled index (col)")) -> (element=w661:string[])  [unwired: 1 in]
          n251 = call "Find_Number_Line.vi"("error in"=w659, "Test Paragraph"=w641, "Row Headers[]"=w661) -> ("error out"=w642:errorcluster, "Line number"=w645:i32)  [unwired: 1 out]
          n252 = call "Reset old test Values (SubVI).vi"("error in"=w642, "Atr in"=w640, "Test Paragraph"=w641) -> ()  [unwired: 8 in, 1 out]
          n253 = control-ref of="Pannel User Message"() -> (w649:refnum<vi>)
          n254 = control-ref of="Stop Burn-in"() -> (w653:refnum<vi>)
          n255 = control-ref of="Config_CANAT"() -> (w650:refnum<vi>)
          n256 = control-ref of="Motor Speed RPM"() -> (w651:refnum<vi>)
          n257 = control-ref of="UUT"() -> (w652:refnum<vi>)
          n258 = control-ref of="Stop Button"() -> (w647:refnum<vi>)
          n259 = control-ref of="ATR"() -> (w648:refnum<vi>)
          n260 = property on="UUT" class="DigNum (strict)"() -> ("Value"=w643:u8)  [unwired: 2 in, 2 out]
          n261 = while {
            shift-right: [w673] -> _
            shift-left: enum16{"Stop", "StopTime", "Speeds", "Start"}."Start" -> [w674]
            tunnel: w647 -> [w672]
            tunnel: w648 -> [w671]
            tunnel: w649 -> [w670]
            tunnel: w650 -> [w669]
            tunnel: w651 -> [w668]
            tunnel: w652 -> [w667]
            tunnel: w653 -> [w666]
            tunnel: w645 -> [w665]
            tunnel: w644 -> [w664]
            tunnel: w643 -> [w662]
            stop <- w663 stop-if-true
            n262 = case shown="\"Start\"" w674 {
              tunnel: [w678 w707 w748 w792] -> w673
              tunnel: w672 -> [_ w702 w752 w790]
              tunnel: w671 -> [_ w692 w756 _]
              tunnel: w670 -> [_ w703 w753 _]
              tunnel: w669 -> [w676 w705 w755 _]
              tunnel: w668 -> [_ w700 w750 _]
              tunnel: w667 -> [w677 w704 w747 _]
              tunnel: w666 -> [_ w701 w751 _]
              tunnel: w665 -> [_ _ w757 _]
              tunnel: w664 -> [_ _ w754 _]
              tunnel: [w675 w706 w749 FALSE ("Value")] -> w663
              tunnel: w662 -> [_ _ w740 _]
              frame "Stop", Default {
                n263 = flat-sequence {
                  tunnel: w677 -> [w681]
                  tunnel: w676 -> [w680]
                  tunnel: [enum16{"Stop", "StopTime", "Speeds", "Start"}."Stop"] -> w678
                  tunnel: [TRUE] -> w675
                  frame #0 {
                    n264 = call "CANSendMotorSpeed.vi"("Remote"=TRUE, "Motor Speed RPM"=u16 0, "UUT"=w681, "CAN Cluster in"=w680) -> ("error out"=w686:errorcluster)  [unwired: 7 in]
                    n265 = property on="VISA Tester" class="VISAName"() -> ("Value"=w687:refnum<visa-resource-name>)  [unwired: 2 in, 2 out]
                    n266 = call "TesterOption (SubVI).vi"("2 Options"=FALSE, "error in (no error)"=w686, "On/Off"=FALSE, "Tester Option"=T11."Venable", "VISA Refnum in"=w687) -> ()  [unwired: 5 in, 2 out]
                  }
                  frame #1 {
                  }
                }
              }
              frame "StopTime" {
                n267 = call "Table_ScrollaBarMarvin.vi"("Line to focus"="6", "reference in"=w692) -> ("error out"=w693:errorcluster)  [unwired: 1 in, 2 out]
                n268 = call "CANSendMotorSpeed.vi"("Remote"=TRUE, "error in (no error)"=w693, "Motor Speed RPM"=u16 0, "UUT"=w704, "CAN Cluster in"=w705) -> ("error out"=w711:errorcluster)  [unwired: 6 in]
                n269 = flat-sequence {
                  tunnel: [w737] -> w710
                  tunnel: w711 -> [w736]
                  tunnel: [w736] -> w712
                  frame #0 {
                    n270 = call <vilib>:"High Resolution Relative Seconds.vi"() -> ("relative seconds"=w737:dbl)
                  }
                }
                n271 = while {
                  tunnel: [w732] -> w706
                  tunnel: w703 -> [w730]
                  tunnel: w702 -> [w729]
                  tunnel: w701 -> [w727]
                  tunnel: w700 -> [w726]
                  tunnel: "6. Stop Time Test in process..." ("Value") -> [w714]
                  tunnel: [w722] -> w690
                  tunnel: w712 -> [w734]
                  tunnel: [w723] -> w698
                  tunnel: w710 -> [w733]
                  tunnel: [w721] -> w694
                  stop <- w713 stop-if-true
                  n272 = call "Write panel message (SubVI).vi"("Stop BurnIn"=w727, 4:"rpm"=w726, 5:"rpm"=TRUE ("rpm"), "PrintTime"=FALSE, "Stop"=w729, "error in (no error)"=w734, "Time to wait"=0.1, "Strin"=w714, "String in"=w730) -> ("error out"=w731:errorcluster)  [unwired: 2 in]
                  n273 = control-ref of="Motor Speed RPM"() -> (w720:refnum<vi>)
                  n274 = property class="DigNum (strict)"(reference=w720, error in=w731) -> (error out=w723:errorcluster, "Value"=w719:dbl)  [unwired: 1 out]
                  n275 = call <vilib>:"High Resolution Relative Seconds.vi"() -> ("relative seconds"=w717:dbl)
                  n276 = property class="Bool (strict)"(reference=w729) -> ("Value"=w732:bool)  [unwired: 1 in, 2 out]
                  n277 = Subtract(x=w717, y=w733) -> (x-y=w721:dbl)
                  n278 = Greater Or Equal?(x=w721, y=50.0) -> (x >= y?=w715:bool)
                  n279 = Less Or Equal?(x=w719, y=0.0) -> (x <= y?=w722:bool)
                  n280 = Compound Arithmetic op=OR(w722, w715, w732) -> (w713:bool)
                }
                "StopTimeResult" <- w690
                n281 = call "Find_Number_LineMARVIN.vi"("Test Paragraph"="6", "TableIn"=w692) -> ("Line number"=w695:i32)  [unwired: 3 in, 3 out]
                n282 = call "PassOrFail (SubVI).vi"("index (row)"=w695, "error in (no error)"=w698, "Data in"=w694, "Pass?Fail"=w690, "Table in"=w692) -> ("error out"=w697:errorcluster)  [unwired: 6 in]
                n283 = flat-sequence {
                  tunnel: [enum16{"Stop", "StopTime", "Speeds", "Start"}."Stop"] -> w707
                  tunnel: w697 -> [_]
                  frame #0 {
                  }
                }
              }
              frame "Speeds" {
                n284 = Equal?(x=w740, y=u8 95) -> (x = y?=w745:bool)
                n285 = Select(t=u16[] [6000, 11500, 15100], s=w745, f=u16[] [6000, 9000, 12100]) -> (s? t:f=w742:u16[])
                n286 = for {
                  tunnel: w742 -> [w783] mode=indexing
                  tunnel: w757 -> [w776]
                  tunnel: w756 -> [w775]
                  tunnel: w747 -> [w774]
                  tunnel: w755 -> [w773]
                  tunnel: w754 -> [w772]
                  tunnel: w753 -> [w771]
                  tunnel: w752 -> [w770]
                  tunnel: w751 -> [w768]
                  tunnel: w750 -> [w766]
                  tunnel: [w764] -> w749
                  tunnel: [w763] -> w741
                  tunnel: [w762] -> w739 mode=indexing
                  i -> [w782]
                  stop <- w764 stop-if-true
                  w784 = 200.0 ("y")
                  n287 = Increment(x=w782) -> (x+1=w781:i32)
                  n288 = Add(x=w776, y=w781) -> (x+y=w777:i32)
                  n289 = call "CANSendMotorSpeed.vi"("Remote"=TRUE, "Motor Speed RPM"=w783, "UUT"=w774, "CAN Cluster in"=w773) -> ("error out"=w788:errorcluster)  [unwired: 7 in]
                  n290 = control-ref of="Motor Speed RPM"() -> (w789:refnum<vi>)
                  n291 = call "Write panel message (SubVI).vi"("Stop BurnIn"=w768, 4:"rpm"=w766, 5:"rpm"=TRUE ("rpm"), "PrintTime"=TRUE, "Stop"=w770, "error in (no error)"=w788, "Time to wait"=25.0 ("Delay Time (sec)"), "Strin"=w772, "String in"=w771) -> ("error out"=w780:errorcluster)  [unwired: 2 in]
                  n292 = property class="DigNum (strict)"(reference=w789, error in=w780) -> (error out=w787:errorcluster, "Value"=w765:dbl)  [unwired: 1 out]
                  n293 = property class="Bool (strict)"(reference=w770) -> ("Value"=w764:bool)  [unwired: 1 in, 2 out]
                  n294 = Add(x=w783, y=w784) -> (x+y=w786:dbl)
                  n295 = Subtract(x=w783, y=w784) -> (x-y=w785:dbl)
                  n296 = In Range and Coerce(upper limit=w786, x=w765, lower limit=w785) -> (In Range?=w762:bool)  [unwired: 1 out]
                  n297 = call "PassOrFail (SubVI).vi"("index (row)"=w777, "error in (no error)"=w787, "Data in"=w765, "Pass?Fail"=w762, "Table in"=w775) -> ("error out"=w763:errorcluster)  [unwired: 6 in]
                }
                n298 = flat-sequence {
                  tunnel: w749 -> [w761]
                  tunnel: [w759] -> w748
                  tunnel: w741 -> [_]
                  frame #0 {
                    n299 = Select(t=enum16{"Stop", "StopTime", "Speeds", "Start"}."Stop", s=w761, f=enum16{"Stop", "StopTime", "Speeds", "Start"}."StopTime") -> (s? t:f=w759:enum16{"Stop", "StopTime", "Speeds", "Start"})
                  }
                }
                n300 = And Array Elements(Boolean array=w739) -> (logical AND=→"SpeedResult":bool)
              }
              frame "Start" {
                n301 = property on="VISA Tester" class="VISAName"() -> ("Value"=w800:refnum<visa-resource-name>)  [unwired: 2 in, 2 out]
                n302 = call "TesterOption (SubVI).vi"("2 Options"=FALSE, "On/Off"=TRUE, "Tester Option"=T11."Venable", "VISA Refnum in"=w800) -> ("error out"=w791:errorcluster)  [unwired: 6 in, 1 out]
                n303 = property class="Bool (strict)"(reference=w790, error in=w791) -> ("Value"=w796:bool)  [unwired: 2 out]
                n304 = Select(t=enum16{"Stop", "StopTime", "Speeds", "Start"}."Stop", s=w796, f=enum16{"Stop", "StopTime", "Speeds", "Start"}."Speeds") -> (s? t:f=w792:enum16{"Stop", "StopTime", "Speeds", "Start"})
              }
            }
          }
        }
        frame "Stop Time" {
          w804 = "3. Motor Temperature test in process..." ("Value")
          w802 = "3" ("Test Paragraph")
          n305 = control-ref of="Pannel User Message"() -> (w812:refnum<vi>)
          n306 = property class="Str"(reference=w812, error in=w811, "Value"=w804) -> (error out=w810:errorcluster)  [unwired: 1 out]
          n307 = call "Table_ScrollaBarMarvin.vi"("error in"=w810, "Line to focus"=w802, "reference in"=w801) -> ("error out"=w814:errorcluster)  [unwired: 2 out]
          n308 = property class="Tbl (strict)"(reference=w801, error in=w814) -> (reference out=w807:refnum<vi>, error out=w816:errorcluster, "Value"=w817:string[][])
          n309 = Index Array(array=w817, index (col)=0 ("disabled index (col)")) -> (element=w818:string[])  [unwired: 1 in]
          n310 = call "Find_Number_LineMARVIN.vi"("Test Paragraph"=w802, "error in"=w816, "TableIn"=w801, "Row Headers[]"=w818) -> ("error out"=w813:errorcluster, "Line number"=w806:i32)  [unwired: 1 in, 2 out]
          n311 = call "Reset old test Values (SubVI).vi"("error in"=w813, "Atr in"=w801, "Test Paragraph"=w802) -> ("error out"=w803:errorcluster)  [unwired: 8 in]
          n312 = property on="Status" class="Bool (strict)"(error in=w803) -> (error out=w808:errorcluster, "Value"=w809:bool)  [unwired: 1 in, 1 out]
          n313 = case shown="True" w809 {
            selector: w809 -> [w822 _]
            tunnel: w808 -> [w824 _]
            tunnel: w807 -> [w821 _]
            tunnel: w806 -> [w820 w827]
            tunnel: w805 -> [_ w832]
            tunnel: w804 -> [_ w828]
            frame False {
              n314 = flat-sequence {
                tunnel: w824 -> [w825]
                tunnel: [w825] -> w823
                frame #0 {
                  n315 = One Button Dialog(message="Please establish RS connection.") -> ()  [unwired: 1 in, 1 out]
                }
              }
              n316 = Increment(x=w820) -> (x+1=w819:i32)
              n317 = call "PassOrFail (SubVI).vi"("index (row)"=w819, "error in (no error)"=w823, "Pass?Fail"=w822, "Table in"=w821) -> ()  [unwired: 7 in, 1 out]
            }
            frame True {
              n318 = control-ref of="Stop Burn-in"() -> (w834:refnum<vi>)
              n319 = control-ref of="Pannel User Message"() -> (w836:refnum<vi>)
              n320 = control-ref of="Config_CANAT"() -> (w830:refnum<vi>)
              n321 = control-ref of="ATR"() -> (w837:refnum<vi>)
              n322 = control-ref of="Motor Speed RPM"() -> (w838:refnum<vi>)
              n323 = control-ref of="UUT"() -> (w829:refnum<vi>)
              n324 = control-ref of="Stop Button"() -> (w835:refnum<vi>)
              n325 = property on="VISA Tester" class="VISAName"() -> ("Value"=w831:refnum<visa-resource-name>)  [unwired: 2 in, 2 out]
              n326 = while {
                shift-right: [w842] -> _
                shift-left: T14."Start" -> [w852]
                tunnel: w834 -> [w851]
                tunnel: w835 -> [w850]
                tunnel: w836 -> [w849]
                tunnel: w837 -> [w848]
                tunnel: w838 -> [w847]
                tunnel: w832 -> [w846]
                tunnel: w831 -> [w845]
                tunnel: w830 -> [w844]
                tunnel: w829 -> [w843]
                tunnel: w828 -> [w840]
                tunnel: w827 -> [w839]
                stop <- w841 stop-if-true
                n327 = case shown="\"Start\"" w852 {
                  tunnel: w851 -> [_ w875 w934]
                  tunnel: w850 -> [_ w867 w936]
                  tunnel: w849 -> [_ w876 w938]
                  tunnel: w848 -> [_ w865 _]
                  tunnel: w847 -> [_ w874 w933]
                  tunnel: w846 -> [_ w879 _]
                  tunnel: w845 -> [w855 w878 w927]
                  tunnel: w844 -> [_ _ w944]
                  tunnel: w843 -> [_ _ w943]
                  tunnel: [w853 w868 w929] -> w842
                  tunnel: [w854 FALSE FALSE] -> w841
                  tunnel: w840 -> [_ w877 _]
                  tunnel: w839 -> [_ w864 _]
                  frame "Stop", Default {
                    n328 = flat-sequence {
                      tunnel: w855 -> [w856]
                      tunnel: [TRUE] -> w854
                      tunnel: [T14."Stop"] -> w853
                      frame #0 {
                        n329 = call "TesterOption (SubVI).vi"("2 Options"=FALSE, "On/Off"=FALSE, "Tester Option"=T11."Venable", "VISA Refnum in"=w856) -> ()  [unwired: 6 in, 2 out]
                      }
                      frame #1 {
                      }
                    }
                  }
                  frame "TA[5]" {
                    w880 = T17 [enum."60C", enum."90C", enum."120C"] items=["K15", "K16", "K17", "Venable", "Firmeware", "Fan", "Power", "120C", "110C", "100C", "90C", "80C", "70C", "60C", "50C", "40C", "30C", "25C", "20C", "10C", "0C"]
                    n330 = for {
                      tunnel: w880 -> [w904] mode=indexing
                      tunnel: w879 -> [w903]
                      tunnel: w878 -> [w902]
                      tunnel: w877 -> [w901]
                      tunnel: w876 -> [w900]
                      tunnel: w867 -> [w899]
                      tunnel: w875 -> [w898]
                      tunnel: w874 -> [w897]
                      tunnel: dbl[] [60.0, 90.0, 120.0] -> [w887] mode=indexing
                      tunnel: [w886] -> w866
                      tunnel: w865 -> [w893]
                      tunnel: w864 -> [w892]
                      tunnel: [w881] -> w863 mode=indexing
                      i -> [w890]
                      w885 = 3.0 ("y")
                      n331 = for {
                        N: 5 -> [_]
                        tunnel: w904 -> [w906]
                        tunnel: w903 -> [w922]
                        tunnel: w902 -> [w918]
                        tunnel: w901 -> [w916]
                        tunnel: w900 -> [w915]
                        tunnel: w899 -> [w914]
                        tunnel: w898 -> [w912]
                        tunnel: w897 -> [w909]
                        tunnel: [w908] -> w896 mode=indexing
                        tunnel: [w907] -> w894
                        n332 = call "TesterOption (SubVI).vi"("2 Options"=FALSE, "On/Off"=TRUE, "Tester Option"=w906, "VISA Refnum in"=w918) -> ("error out"=w919:errorcluster)  [unwired: 6 in, 1 out]
                        n333 = call "Write panel message (SubVI).vi"("Stop BurnIn"=w912, 4:"rpm"=w909, 5:"rpm"=FALSE ("rpm"), "PrintTime"=FALSE, "Stop"=w914, "error in (no error)"=w919, "Time to wait"=1.0, "Strin"=w916, "String in"=w915) -> ("error out"=w917:errorcluster)  [unwired: 2 in]
                        n334 = call "SerialMarvinSendGet.vi"("error in (no error)"=w917, "write buffer"="TA[2]\r\n", "VISA resource name"=w922) -> ("error out"=w907:errorcluster, "read buffer"=w920:string)  [unwired: 7 in]
                        n335 = Fract/Exp String To Number(string=w920) -> (number=w908:dbl)  [unwired: 3 in, 1 out]
                      }
                      n336 = Increment(x=w890) -> (x+1=w889:i32)
                      n337 = Add Array Elements(numeric array=w896) -> (sum=w895:dbl)
                      n338 = Add(x=w887, y=w885) -> (x+y=w884:dbl)
                      n339 = Subtract(x=w887, y=w885) -> (x-y=w883:dbl)
                      n340 = Divide(x=w895, y=5.0) -> (x/y=w882:dbl)
                      n341 = In Range and Coerce(upper limit=w884, x=w882, lower limit=w883) -> (In Range?=w881:bool)  [unwired: 1 out]
                      n342 = Add(x=w892, y=w889) -> (x+y=w891:i32)
                      n343 = call "PassOrFail (SubVI).vi"("index (row)"=w891, "error in (no error)"=w894, "Data in"=w882, "Pass?Fail"=w881, "Table in"=w893) -> ("error out"=w886:errorcluster)  [unwired: 6 in]
                    }
                    n344 = property class="Bool (strict)"(reference=w867, error in=w866) -> ("Value"=w872:bool)  [unwired: 2 out]
                    n345 = Select(t=T14."Stop", s=w872, f=T14."Stop") -> (s? t:f=w868:T14)
                    n346 = And Array Elements(Boolean array=w863) -> (logical AND=→"MotorTempResult":bool)
                  }
                  frame "Start" {
                    n347 = call "Write panel message (SubVI).vi"("Stop BurnIn"=w934, 4:"rpm"=w933, 5:"rpm"=FALSE ("rpm"), "PrintTime"=FALSE, "Stop"=w936, "Time to wait"=0.1, "Strin"="3. Motor Temperature test in process...\nInitialization state...", "String in"=w938) -> ("error out"=w939:errorcluster)  [unwired: 3 in]
                    n348 = call "TesterOption (SubVI).vi"("2 Options"=FALSE, "error in (no error)"=w939, "On/Off"=FALSE, "Tester Option"=T11."Venable", "VISA Refnum in"=w927) -> ("error out"=w941:errorcluster)  [unwired: 5 in, 1 out]
                    n349 = call "CANSendMotorSpeed.vi"("Remote"=TRUE, "error in (no error)"=w941, "Motor Speed RPM"=u16 0, "UUT"=w943, "CAN Cluster in"=w944) -> ("error out"=w926:errorcluster)  [unwired: 6 in]
                    n350 = property class="Bool (strict)"(reference=w936, error in=w926) -> ("Value"=w948:bool)  [unwired: 2 out]
                    n351 = Select(t=T14."Stop", s=w948, f=T14."TA[5]") -> (s? t:f=w929:T14)
                  }
                }
              }
            }
          }
        }
        frame "Temp Control" {
          w951 = "7. Temperature control test in process..." ("Value")
          w949 = "7" ("Test Paragraph")
          n352 = control-ref of="Pannel User Message"() -> (w963:refnum<vi>)
          n353 = property class="Str"(reference=w963, error in=w962, "Value"=w951) -> (error out=w961:errorcluster)  [unwired: 1 out]
          n354 = control-ref of="Pannel User Message"() -> (w956:refnum<vi>)
          n355 = control-ref of="Motor Speed RPM"() -> (w954:refnum<vi>)
          n356 = control-ref of="Stop Button"() -> (w958:refnum<vi>)
          n357 = control-ref of="ATR"() -> (w957:refnum<vi>)
          n358 = control-ref of="Config_CANAT"() -> (w955:refnum<vi>)
          n359 = control-ref of="UUT"() -> (w953:refnum<vi>)
          n360 = control-ref of="Stop Burn-in"() -> (w952:refnum<vi>)
          n361 = call "Table_ScrollaBarMarvin.vi"("error in"=w961, "Line to focus"=w949, "reference in"=w964) -> ("error out"=w960:errorcluster)  [unwired: 2 out]
          n362 = call "Reset old test Values (SubVI).vi"("error in"=w960, "Atr in"=w964, "Test Paragraph"=w949) -> ("error out"=w950:errorcluster)  [unwired: 8 in]
          n363 = while {
            tunnel: w950 -> [w976]
            shift-right: [w974] -> _
            shift-left: enum16{"Stop", "Algorithm", "Start"}."Start" -> [w975]
            tunnel: w958 -> [w973]
            tunnel: w957 -> [w972]
            tunnel: w956 -> [w971]
            tunnel: w955 -> [w970]
            tunnel: w954 -> [w969]
            tunnel: w953 -> [w968]
            tunnel: w952 -> [w966]
            tunnel: w951 -> [w965]
            stop <- w967 stop-if-true
            n364 = case shown="\"Algorithm\"" w975 {
              tunnel: w976 -> [_ _ w1098]
              tunnel: [w977 w997 w1087] -> w974
              tunnel: w973 -> [_ w1008 w1091]
              tunnel: w972 -> [_ w1004 _]
              tunnel: w971 -> [_ w1009 _]
              tunnel: w970 -> [w980 _ w1084]
              tunnel: w969 -> [_ w1005 _]
              tunnel: w968 -> [w979 _ w1083]
              tunnel: [w978 FALSE FALSE] -> w967
              tunnel: w966 -> [_ w1007 _]
              tunnel: w965 -> [_ w1006 _]
              frame "Stop", Default {
                n365 = flat-sequence {
                  tunnel: w980 -> [w985]
                  tunnel: w979 -> [w983]
                  tunnel: [TRUE] -> w978
                  tunnel: [enum16{"Stop", "Algorithm", "Start"}."Stop"] -> w977
                  frame #0 {
                    n366 = call "CANSendMotorSpeed.vi"("Remote"=TRUE, "Motor Speed RPM"=u16 0, "UUT"=w983, "CAN Cluster in"=w985) -> ("error out"=w981:errorcluster)  [unwired: 7 in]
                    n367 = property on="VISA Tester" class="VISAName"() -> ("Value"=w989:refnum<visa-resource-name>)  [unwired: 2 in, 2 out]
                    n368 = call "TesterOption (SubVI).vi"("2 Options"=FALSE, "error in (no error)"=w981, "On/Off"=FALSE, "Tester Option"=T11."Venable", "VISA Refnum in"=w989) -> ()  [unwired: 5 in, 2 out]
                  }
                  frame #1 {
                  }
                  frame #2 {
                  }
                }
              }
              frame "Algorithm" {
                w992 = T18 [enum."6000", enum."11500", enum."15100", enum."11500-2", enum."6000-2"] items=["6000", "11500", "15100", "11500-2", "6000-2"]
                # "Speed Goal"
                # "Speed Ind"
                # "Temp Goal"
                # "50 Deg"
                n369 = for {
                  tunnel: w1009 -> [w1036]
                  tunnel: w1008 -> [w1035]
                  tunnel: w1007 -> [w1034]
                  tunnel: w1006 -> [w1033]
                  tunnel: w1005 -> [w1032]
                  tunnel: w1004 -> [w1019]
                  tunnel: string[] ["7.1", "7.3", "7.5", "7.7", "7.9"] -> [w1017] mode=indexing
                  shift-right: [w1029] -> _
                  shift-left: 1202.0 ("Rt") -> [w1030]
                  tunnel: dbl[] [68.0, 68.0, 88.0, 80.0, 60.0] -> [w1028] mode=indexing
                  tunnel: dbl[] [6000.0, 11500.0, 15100.0, 11500.0, 6000.0] -> [w1027] mode=indexing
                  tunnel: dbl[] [6000.0, 6400.0, 11700.0, 14600.0, 11000.0] -> [w1026] mode=indexing
                  tunnel: [w1015] -> w998
                  tunnel: [w1014] -> w994 mode=indexing
                  tunnel: [w1013] -> w995 mode=indexing
                  tunnel: w992 -> [w1012] mode=indexing
                  stop <- w1031 stop-if-true
                  n370 = call <vilib>:"High Resolution Relative Seconds.vi"() -> ("relative seconds"=w1025:dbl)
                  n371 = while {
                    tunnel: w1036 -> [w1065]
                    tunnel: w1035 -> [w1057]
                    tunnel: w1034 -> [w1064]
                    tunnel: w1033 -> [w1043]
                    tunnel: w1032 -> [w1066]
                    shift-right: [w1062] -> w1029
                    shift-left: w1030 -> [w1061]
                    tunnel: w1012 -> [w1063]
                    tunnel: w1028 -> [w1060]
                    tunnel: w1027 -> [w1059]
                    tunnel: w1026 -> [w1058]
                    tunnel: w1025 -> [w1054]
                    tunnel: [w1049] -> w1020
                    tunnel: [w1048] -> w1013
                    tunnel: [w1047] -> w1018
                    tunnel: [w1046] -> w1014
                    tunnel: [w1045] -> w1016
                    stop <- w1055 stop-if-true
                    n372 = call "DegToDAC (SubVI).vi"("R2"=0.0, "Rt"=w1061) -> ("error out"=w1073:errorcluster, "output array"=w1074:u8[])  [unwired: 8 in]
                    n373 = call <vilib>:"High Resolution Relative Seconds.vi"() -> ("relative seconds"=w1053:dbl)
                    n374 = property on="VISA Tester" class="VISAName"() -> ("Value"=w1076:refnum<visa-resource-name>)  [unwired: 2 in, 2 out]
                    n375 = Byte Array To String(unsigned byte array=w1074) -> (string=w1075:string)
                    n376 = Subtract(x=w1054, y=w1053) -> (x-y=w1052:dbl)
                    n377 = VISA Write(VISA resource name=w1076, write buffer=w1075, error in (no error)=w1073) -> (error out=w1072:errorcluster)  [unwired: 2 out]
                    n378 = Greater Or Equal?(x=w1052, y=120.0) -> (x >= y?=w1050:bool)
                    n379 = call <vilib>:"Clear Errors.vi"("error in (no error)"=w1072) -> ("error out"=w1071:errorcluster)  [unwired: 5 in, 1 out]
                    n380 = control-ref of="Ambient Temperature"() -> (w1044:refnum<vi>)
                    n381 = property class="DigNum (strict)"(reference=w1044) -> ("Value"=w1042:dbl)  [unwired: 1 in, 2 out]
                    n382 = property class="Bool (strict)"(reference=w1057) -> ("Value"=w1056:bool)  [unwired: 1 in, 2 out]
                    n383 = Number To Fractional String(number=w1042, precision (6)=i16 2) -> (F-format string=w1039:string)  [unwired: 2 in]
                    n384 = Concatenate Strings(w1043, "\nAmbient  Temp. [C]: " ("string"), w1039) -> (w1038:string)
                    n385 = call "Write panel message (SubVI).vi"("Stop BurnIn"=w1064, 4:"rpm"=w1066, 5:"rpm"=TRUE ("rpm"), "PrintTime"=TRUE, "Stop"=w1057, "error in (no error)"=w1071, "Time to wait"=3.0, "Strin"=w1038, "String in"=w1065) -> ("error out"=w1070:errorcluster)  [unwired: 2 in]
                    n386 = call "TempAlgoTest (SubVI).vi"("Temp"=w1044, "Speed Ind"=w1058, "Motor Speed RPM"=w1066, "Round"=w1063, "Temp Up In"=w1061, "error in (no error)"=w1070, "String in"=w1065, "Temp Goal"=w1060, "Stop"=w1057, "Speed Goal"=w1059, "Stop BurnIn"=w1064, "AD Resistor Step"="AD Resistor Step", "Strin"=w1038) -> (14:"Speed Pass/Fail"=w1048:bool, "Temp  Pass/Fail"=w1047:dbl, "Temp Up Out"=w1062:dbl, 17:"Speed Pass/Fail"=w1049:dbl, "Temp Pass/Fail"=w1046:bool, "error out"=w1045:errorcluster)  [unwired: 1 in]
                    n387 = Compound Arithmetic op=OR(w1050, w1048, w1056) -> (w1055:bool)
                  }
                  n388 = property class="Bool (strict)"(reference=w1035) -> ("Value"=w1031:bool)  [unwired: 1 in, 2 out]
                  n389 = call "Find_Number_LineMARVIN.vi"("Test Paragraph"=w1017, "error in"=w1016, "TableIn"=w1019) -> ("error out"=w1021:errorcluster, "Line number"=w1024:i32)  [unwired: 2 in, 2 out]
                  n390 = Increment(x=w1024) -> (x+1=w1023:i32)
                  n391 = call "PassOrFail (SubVI).vi"("index (row)"=w1023, "error in (no error)"=w1021, "Data in"=w1018, "Pass?Fail"=w1014, "Table in"=w1019) -> ("error out"=w1022:errorcluster)  [unwired: 6 in]
                  n392 = call "PassOrFail (SubVI).vi"("index (row)"=w1024, "error in (no error)"=w1022, "Data in"=w1020, "Pass?Fail"=w1013, "Table in"=w1019) -> ("error out"=w1015:errorcluster)  [unwired: 6 in]
                }
                n393 = Build Array (concatenate)(w995, w994) -> (w996:bool[])
                n394 = flat-sequence {
                  tunnel: w998 -> [_]
                  tunnel: [enum16{"Stop", "Algorithm", "Start"}."Stop"] -> w997
                  frame #0 {
                  }
                }
                n395 = And Array Elements(Boolean array=w996) -> (logical AND=→"TempControlResult":bool)
              }
              frame "Start" {
                n396 = call <vilib>:"Clear Errors.vi"("error in (no error)"=w1098) -> ("error out"=w1080:errorcluster)  [unwired: 5 in, 1 out]
                n397 = property on="VISA Tester" class="VISAName"() -> ("Value"=w1097:refnum<visa-resource-name>)  [unwired: 2 in, 2 out]
                n398 = call "TesterOption (SubVI).vi"("On/Off 2"=TRUE, "Tester Option 2"=T11."Venable", "2 Options"=TRUE, "error in (no error)"=w1080, "On/Off"=TRUE, "Tester Option"=T11."K16", "VISA Refnum in"=w1097) -> ("error out"=w1079:errorcluster)  [unwired: 3 in, 1 out]
                n399 = call "Time Delay12"("error in (no error)"=w1079) -> ("error out"=w1078:errorcluster)  [unwired: 10 in]
                n400 = call "CANSendMotorSpeed.vi"("Remote"=FALSE, "error in (no error)"=w1078, "Motor Speed RPM"=u16 0, "UUT"=w1083, "CAN Cluster in"=w1084) -> ("error out"=w1085:errorcluster)  [unwired: 6 in]
                n401 = property class="Bool (strict)"(reference=w1091, error in=w1085) -> ("Value"=w1090:bool)  [unwired: 2 out]
                n402 = Select(t=enum16{"Stop", "Algorithm", "Start"}."Stop", s=w1090, f=enum16{"Stop", "Algorithm", "Start"}."Algorithm") -> (s? t:f=w1087:enum16{"Stop", "Algorithm", "Start"})
              }
            }
          }
        }
        frame "Burn in" {
          n403 = control-ref of="Stop Button"() -> (w1102:refnum<vi>)
          n404 = control-ref of="Pannel User Message"() -> (w1105:refnum<vi>)
          n405 = control-ref of="ATR"() -> (w1101:refnum<vi>)
          n406 = control-ref of="Config_CANAT"() -> (w1104:refnum<vi>)
          n407 = control-ref of="UUT"() -> (w1103:refnum<vi>)
          n408 = control-ref of="Stop Burn-in"() -> (w1100:refnum<vi>)
          n409 = property on="UUT" class="DigNum (strict)"() -> ("Value"=w1099:u8)  [unwired: 2 in, 2 out]
          n410 = while {
            tunnel: w1105 -> [w1116]
            tunnel: w1101 -> [w1115]
            tunnel: w1104 -> [w1114]
            tunnel: w1103 -> [w1113]
            tunnel: w1102 -> [w1112]
            shift-right: [w1111] -> _
            shift-left: T15."Start" -> [w1118]
            shift-right: [w1117] -> _
            shift-left: _ -> [w1109]
            tunnel: w1100 -> [w1108]
            tunnel: w1099 -> [w1107]
            stop <- w1110 stop-if-true
            n411 = case shown="\"Stop\", Default" w1118 {
              tunnel: [w1121 w1156 w1224 w1253 w1286 w1322] -> w1117
              tunnel: w1116 -> [_ w1148 _ _ _ w1321]
              tunnel: w1115 -> [_ w1151 w1197 w1240 w1272 w1308]
              tunnel: w1114 -> [_ w1147 _ _ _ w1320]
              tunnel: w1113 -> [_ w1144 _ _ _ w1299]
              tunnel: w1112 -> [_ _ w1226 w1255 w1290 w1314]
              tunnel: [w1119 T15."Stop" w1227 w1256 w1291 w1310] -> w1111
              tunnel: [w1120 FALSE FALSE FALSE FALSE FALSE] -> w1110
              tunnel: w1109 -> [w1121 w1156 w1224 w1253 w1286 _]
              tunnel: w1108 -> [_ _ _ _ _ w1304]
              tunnel: w1107 -> [_ w1136 w1188 w1232 w1264 w1298]
              frame "Stop", Default {
                n412 = flat-sequence {
                  tunnel: [TRUE] -> w1120
                  tunnel: [T15."Stop"] -> w1119
                  frame #0 {
                    n413 = property on="VISA Tester" class="VISAName"() -> ("Value"=w1126:refnum<visa-resource-name>)  [unwired: 2 in, 2 out]
                    n414 = call "TesterOption (SubVI).vi"("2 Options"=FALSE, "On/Off"=FALSE, "Tester Option"=T11."Venable", "VISA Refnum in"=w1126) -> ("error out"=w1123:errorcluster)  [unwired: 6 in, 1 out]
                    n415 = property on="Stop Burn-in" class="Bool (strict)"(error in=w1123, "Visible"=FALSE) -> ()  [unwired: 1 in, 2 out]
                  }
                  frame #1 {
                  }
                }
              }
              frame "BurnIn" {
                w1140 = FALSE ("Stop Burn-in")
                n416 = control-ref of="Motor Speed RPM"() -> (w1150:refnum<vi>)
                n417 = control-ref of="Stop Button"() -> (w1149:refnum<vi>)
                n418 = property on="Stop Burn-in" class="Bool (strict)"("Visible"=TRUE) -> (error out=w1152:errorcluster)  [unwired: 2 in, 1 out]
                n419 = Equal?(x=w1136, y=u8 95) -> (x = y?=w1133:bool)
                n420 = Select(t="8. " ("Test Paragraph"), s=w1133, f="7. " ("Test Paragraph")) -> (s? t:f=w1132:string)
                n421 = Select(t="8.4" ("Test Paragraph"), s=w1133, f="7.4" ("Test Paragraph")) -> (s? t:f=w1137:string)
                n422 = call "Find_Number_LineMARVIN.vi"("Test Paragraph"=w1137, "error in"=w1152, "TableIn"=w1151) -> ("error out"=w1154:errorcluster, "Line number"=w1155:i32)  [unwired: 2 in, 2 out]
                n423 = Select(t=u16 15100, s=w1133, f=u16 12100 ("y")) -> (s? t:f=w1142:u16)
                n424 = for {
                  tunnel: w1154 -> [w1176]
                  tunnel: dbl[] [600.0, 600.0, 600.0] -> [w1180] mode=indexing
                  tunnel: w1155 -> [w1185]
                  tunnel: w1151 -> [w1175]
                  tunnel: w1150 -> [w1174]
                  tunnel: w1149 -> [w1173]
                  tunnel: w1148 -> [w1172]
                  tunnel: w1147 -> [w1168]
                  tunnel: w1144 -> [w1167]
                  tunnel: w1142 -> [w1166]
                  tunnel: [w1164] -> w1141
                  tunnel: w1132 -> [w1161]
                  tunnel: [w1160] -> w1131 mode=indexing
                  i -> [w1182]
                  n425 = call "CANSendMotorSpeed.vi"("Remote"=TRUE, "error in (no error)"=w1176, "Motor Speed RPM"=w1166, "UUT"=w1167, "CAN Cluster in"=w1168) -> ("error out"=w1170:errorcluster)  [unwired: 6 in]
                  n426 = control-ref of="Stop Burn-in"() -> (w1171:refnum<vi>)
                  n427 = Concatenate Strings(w1161, "Burn-in test in process..." ("Strin")) -> (w1162:string)
                  n428 = Add(x=w1185, y=w1182) -> (x+y=w1181:i32)
                  n429 = call "Write panel message (SubVI).vi"("Stop BurnIn"=w1171, 4:"rpm"=w1174, 5:"rpm"=TRUE ("rpm"), "PrintTime"=TRUE, "Stop"=w1173, "error in (no error)"=w1170, "Time to wait"=w1180, "Strin"=w1162, "String in"=w1172) -> ("error out"=w1177:errorcluster)  [unwired: 2 in]
                  n430 = control-ref of="Power transistor Heat sink Temp."() -> (w1186:refnum<vi>)
                  n431 = property on="MaxBurnInTempVal" class="DigNum (strict)"() -> ("Value"=w1184:dbl)  [unwired: 2 in, 2 out]
                  n432 = property class="DigNum (strict)"(reference=w1186, error in=w1177) -> (error out=w1165:errorcluster, "Value"=w1183:dbl)  [unwired: 1 out]
                  n433 = Less Or Equal?(x=w1183, y=w1184) -> (x <= y?=w1160:bool)
                  n434 = call "PassOrFail (SubVI).vi"("index (row)"=w1181, "error in (no error)"=w1165, "Data in"=w1183, "Pass?Fail"=w1160, "Table in"=w1175) -> ("error out"=w1164:errorcluster)  [unwired: 6 in]
                }
                n435 = And Array Elements(Boolean array=w1131) -> (logical AND=→"BurnResult":bool)
                n436 = property on="Stop Burn-in" class="Bool (strict)"(error in=w1141, "Value"=w1140, "Visible"=w1140) -> ()  [unwired: 1 in, 2 out]
              }
              frame "Ambient Temp" {
                w1202 = 2 ("disabled index (col)")
                n437 = control-ref of="Power transistor Heat sink Temp."() -> (w1212:refnum<vi>)
                n438 = Equal?(x=w1188, y=u8 95) -> (x = y?=w1191:bool)
                n439 = Select(t="8.3" ("Test Paragraph"), s=w1191, f="7.3" ("Test Paragraph")) -> (s? t:f=w1189:string)
                n440 = call "Find_Number_LineMARVIN.vi"("Test Paragraph"=w1189, "TableIn"=w1197) -> ("error out"=w1223:errorcluster, "Line number"=w1203:i32)  [unwired: 3 in, 2 out]
                n441 = property class="DigNum (strict)"(reference=w1212, error in=w1223) -> (error out=w1214:errorcluster, "Value"=w1204:dbl)  [unwired: 1 out]
                n442 = Select(t=25.0 ("y"), s=w1191, f=25.0 ("y")) -> (s? t:f=w1213:dbl)
                n443 = Select(t=13.0 ("y"), s=w1191, f=13.0) -> (s? t:f=w1215:dbl)
                n444 = Add(x=w1213, y=w1215) -> (x+y=w1222:dbl)
                n445 = Subtract(x=w1213, y=w1215) -> (x-y=w1221:dbl)
                n446 = In Range and Coerce(upper limit=w1222, x=w1204, lower limit=w1221) -> (In Range?=w1187:bool)  [unwired: 1 out]
                "BurnTemp" <- w1187
                n447 = call "PassOrFail (SubVI).vi"("index (row)"=w1203, "error in (no error)"=w1214, "Data in"=w1204, "Pass?Fail"=w1187, "Table in"=w1197) -> ("error out"=w1194:errorcluster)  [unwired: 6 in]
                n448 = property class="Tbl (strict)"(reference=w1197, error in=w1194) -> (reference out=w1196:refnum<vi>, error out=w1211:errorcluster, "Value"=w1210:string[][])
                n449 = Add(x=w1204, y=25.0) -> (x+y=w1195:dbl)
                "MaxBurnInTempVal" <- w1195
                n450 = Number To Fractional String(number=w1195, precision (6)=i16 0) -> (F-format string=w1209:string)  [unwired: 2 in]
                n451 = Concatenate Strings("< " ("string"), w1209) -> (w1198:string)
                n452 = Increment(x=w1203) -> (x+1=w1201:i32)
                n453 = Increment(x=w1201) -> (x+1=w1200:i32)
                n454 = Increment(x=w1200) -> (x+1=w1199:i32)
                n455 = Replace Array Subset(array=w1210, new element #1=w1198, index (row) #1=w1201, index (col) #1=w1202, new element #2=w1198, index (row) #2=w1200, index (col) #2=w1202, new element #3=w1198, index (row) #3=w1199, index (col) #3=w1202) -> (w1208:string[][])
                n456 = property class="Tbl (strict)"(reference=w1196, error in=w1211, "Value"=w1208) -> (error out=w1193:errorcluster)  [unwired: 1 out]
                n457 = property class="Bool (strict)"(reference=w1226, error in=w1193) -> ("Value"=w1230:bool)  [unwired: 2 out]
                n458 = Select(t=T15."Stop", s=w1230, f=T15."BurnIn") -> (s? t:f=w1227:T15)
              }
              frame "MotorSpeed" {
                n459 = control-ref of="Motor Speed RPM"() -> (w1238:refnum<vi>)
                n460 = Equal?(x=w1232, y=u8 95) -> (x = y?=w1235:bool)
                n461 = Select(t="8.2" ("Test Paragraph"), s=w1235, f="7.2" ("Test Paragraph")) -> (s? t:f=w1233:string)
                n462 = call "Find_Number_LineMARVIN.vi"("Test Paragraph"=w1233, "TableIn"=w1240) -> ("error out"=w1252:errorcluster, "Line number"=w1243:i32)  [unwired: 3 in, 2 out]
                n463 = property class="DigNum (strict)"(reference=w1238, error in=w1252) -> (error out=w1241:errorcluster, "Value"=w1242:dbl)  [unwired: 1 out]
                n464 = Select(t=15100.0 ("y"), s=w1235, f=12100.0 ("y")) -> (s? t:f=w1239:dbl)
                n465 = Select(t=200.0 ("y"), s=w1235, f=200.0) -> (s? t:f=w1244:dbl)
                n466 = Add(x=w1239, y=w1244) -> (x+y=w1251:dbl)
                n467 = Subtract(x=w1239, y=w1244) -> (x-y=w1250:dbl)
                n468 = In Range and Coerce(upper limit=w1251, x=w1242, lower limit=w1250) -> (In Range?=w1231:bool)  [unwired: 1 out]
                "BurnSpeed" <- w1231
                n469 = call "PassOrFail (SubVI).vi"("index (row)"=w1243, "error in (no error)"=w1241, "Data in"=w1242, "Pass?Fail"=w1231, "Table in"=w1240) -> ("error out"=w1237:errorcluster)  [unwired: 6 in]
                n470 = property class="Bool (strict)"(reference=w1255, error in=w1237) -> ("Value"=w1259:bool)  [unwired: 2 out]
                n471 = Select(t=T15."Stop", s=w1259, f=T15."Ambient Temp") -> (s? t:f=w1256:T15)
              }
              frame "DC Current Measure" {
                n472 = property on="VISA Tester" class="VISAName"() -> (error out=w1284:errorcluster, "Value"=w1288:refnum<visa-resource-name>)  [unwired: 2 in, 1 out]
                n473 = call "GetADCTester (SubVI).vi"("error in (no error)"=w1284, "GetADCTester"=T13."Current", "TimeToGet"=10, "VISA Refnum in"=w1288) -> ("error out"=w1285:errorcluster, "ADCValOutput Single"=w1271:dbl)  [unwired: 5 in, 1 out]
                n474 = Equal?(x=w1264, y=u8 95) -> (x = y?=w1268:bool)
                n475 = Select(t="8.1" ("Test Paragraph"), s=w1268, f="7.1" ("Test Paragraph")) -> (s? t:f=w1266:string)
                n476 = call "Find_Number_LineMARVIN.vi"("Test Paragraph"=w1266, "error in"=w1285, "TableIn"=w1272) -> ("error out"=w1283:errorcluster, "Line number"=w1273:i32)  [unwired: 2 in, 2 out]
                n477 = Select(t=50.0 ("y"), s=w1268, f=28.0 ("y")) -> (s? t:f=w1275:dbl)
                n478 = Select(t=5.0 ("y"), s=w1268, f=3.0) -> (s? t:f=w1274:dbl)
                n479 = Add(x=w1275, y=w1274) -> (x+y=w1282:dbl)
                n480 = Subtract(x=w1275, y=w1274) -> (x-y=w1281:dbl)
                n481 = In Range and Coerce(upper limit=w1282, x=w1271, lower limit=w1281) -> (In Range?=w1262:bool)  [unwired: 1 out]
                "BurnDC" <- w1262
                n482 = call "PassOrFail (SubVI).vi"("index (row)"=w1273, "error in (no error)"=w1283, "Data in"=w1271, "Pass?Fail"=w1262, "Table in"=w1272) -> ("error out"=w1270:errorcluster)  [unwired: 6 in]
                n483 = property class="Bool (strict)"(reference=w1290, error in=w1270) -> ("Value"=w1261:bool)  [unwired: 2 out]
                n484 = Not(x=w1262) -> (.not. x?=w1260:bool)
                n485 = Or(x=w1260, y=w1261) -> (x .or. y?=w1263:bool)
                n486 = Select(t=T15."Stop", s=w1263, f=T15."MotorSpeed") -> (s? t:f=w1291:T15)
              }
              frame "Start" {
                n487 = Equal?(x=w1298, y=u8 95) -> (x = y?=w1300:bool)
                n488 = Select(t="8" ("Test Paragraph"), s=w1300, f="7" ("Test Paragraph")) -> (s? t:f=w1295:string)
                n489 = Concatenate Strings(w1295, ". Burn-in test in process...\nFull Speed Operation" ("Value")) -> (w1294:string)
                n490 = property class="Str"(reference=w1321, "Value"=w1294) -> (reference out=w1318:refnum<vi>, error out=w1303:errorcluster)  [unwired: 1 in]
                n491 = call "Find_Number_LineMARVIN.vi"("Test Paragraph"=w1295, "error in"=w1303, "TableIn"=w1308) -> ("error out"=w1328:errorcluster, "Line number"=w1329:i32)  [unwired: 2 in, 2 out]
                n492 = Select(t=u16 15100 ("y"), s=w1300, f=u16 12100 ("y")) -> (s? t:f=w1335:u16)
                n493 = call "Table_ScrollaBarMarvin.vi"("error in"=w1328, "Line to focus"=w1295, "reference in"=w1308) -> ("error out"=w1330:errorcluster)  [unwired: 2 out]
                n494 = call "Reset old test Values (SubVI).vi"("error in"=w1330, "Atr in"=w1308, "Test Paragraph"=w1295) -> ("error out"=w1331:errorcluster)  [unwired: 8 in]
                n495 = Increment(x=w1329) -> (x+1=w1322:i32)
                n496 = property on="VISA Tester" class="VISAName"(error in=w1331) -> (error out=w1332:errorcluster, "Value"=w1333:refnum<visa-resource-name>)  [unwired: 1 in, 1 out]
                n497 = call "TesterOption (SubVI).vi"("2 Options"=FALSE, "error in (no error)"=w1332, "On/Off"=TRUE, "Tester Option"=T11."Venable", "VISA Refnum in"=w1333) -> ("error out"=w1334:errorcluster)  [unwired: 5 in, 1 out]
                n498 = call "CANSendMotorSpeed.vi"("Remote"=TRUE, "error in (no error)"=w1334, "Motor Speed RPM"=w1335, "UUT"=w1299, "CAN Cluster in"=w1320) -> ("error out"=w1319:errorcluster)  [unwired: 6 in]
                n499 = control-ref of="Motor Speed RPM"() -> (w1307:refnum<vi>)
                n500 = call "Write panel message (SubVI).vi"("Stop BurnIn"=w1304, 4:"rpm"=w1307, 5:"rpm"=TRUE ("rpm"), "PrintTime"=TRUE, "Stop"=w1314, "error in (no error)"=w1319, "Time to wait"=50.0, "Strin"=w1294, "String in"=w1318) -> ("error out"=w1306:errorcluster)  [unwired: 2 in]
                n501 = property class="Bool (strict)"(reference=w1314, error in=w1306) -> ("Value"=w1313:bool)  [unwired: 2 out]
                n502 = Select(t=T15."Stop", s=w1313, f=T15."DC Current Measure") -> (s? t:f=w1310:T15)
              }
            }
          }
        }
        frame "Visual Inspec" {
          n503 = property on="VISA Tester" class="VISAName"() -> ("Value"=w1346:refnum<visa-resource-name>)  [unwired: 2 in, 2 out]
          n504 = call "TesterOption (SubVI).vi"("2 Options"=FALSE, "error in (no error)"=w1347, "On/Off"=FALSE, "Tester Option"=T11."Venable", "VISA Refnum in"=w1346) -> ("error out"=w1342:errorcluster)  [unwired: 5 in, 1 out]
          n505 = local read "UUT"() -> (w1338:u8)
          n506 = Equal?(x=w1338, y=u8 95) -> (x = y?=w1339:bool)
          n507 = case shown="False" w1339 {
            tunnel: w1348 -> [w1352 w1356]
            tunnel: w1342 -> [w1351 w1355]
            tunnel: [w1349 w1354] -> w1341
            tunnel: [w1350 w1353] -> w1337
            frame False {
              n508 = call "VisualInspectionAHU.vi"("error in (no error)"=w1351, "TableRef"=w1352) -> ("error out"=w1350:errorcluster, "VisualInspectionResult"=w1349:bool)  [unwired: 8 in]
            }
            frame True {
              n509 = call "VisualInspectionEBAY.vi"("error in (no error)"=w1355, "TableRef"=w1356) -> ("error out"=w1353:errorcluster, "VisualInspectionResult"=w1354:bool)  [unwired: 8 in]
            }
          }
          "VisualInspectionResult" <- w1341
          n510 = property on="Automation" class="Bool (strict)"(error in=w1337) -> ("Value"=w1336:bool)  [unwired: 1 in, 2 out]
          n511 = case shown="True" w1336 {
            frame False {
            }
            frame True {
              w1357 = TRUE ("Value (Signaling)")
              n512 = property on="SetSN" class="Bool (strict)"("Val(Sgnl)"=w1357, "Value"=w1357) -> ()  [unwired: 2 in, 2 out]
            }
          }
        }
        frame "Temp Sens Cal" {
          w1361 = "2. Temperature sensor calibration test in process..." ("Value")
          w1359 = "2" ("Test Paragraph")
          n513 = control-ref of="Pannel User Message"() -> (w1368:refnum<vi>)
          n514 = property class="Str"(reference=w1368, error in=w1367, "Value"=w1361) -> (error out=w1366:errorcluster)  [unwired: 1 out]
          n515 = call "Table_ScrollaBarMarvin.vi"("error in"=w1366, "Line to focus"=w1359, "reference in"=w1369) -> ("error out"=w1371:errorcluster)  [unwired: 2 out]
          n516 = property class="Tbl (strict)"(reference=w1369, error in=w1371) -> (reference out=w1358:refnum<vi>, error out=w1373:errorcluster, "Value"=w1374:string[][])
          n517 = Index Array(array=w1374, index (col)=0 ("disabled index (col)")) -> (element=w1375:string[])  [unwired: 1 in]
          n518 = call "Find_Number_Line.vi"("error in"=w1373, "Test Paragraph"=w1359, "Row Headers[]"=w1375) -> ("error out"=w1370:errorcluster, "Line number"=w1363:i32)  [unwired: 1 out]
          n519 = property on="Status" class="Bool (strict)"(error in=w1370) -> (error out=w1364:errorcluster, "Value"=w1365:bool)  [unwired: 1 in, 1 out]
          n520 = call "Reset old test Values (SubVI).vi"("error in"=w1364, "Atr in"=w1358, "Test Paragraph"=w1359) -> ("error out"=w1360:errorcluster)  [unwired: 8 in]
          n521 = case shown="True" w1365 {
            selector: w1365 -> [w1379 _]
            tunnel: w1360 -> [w1381 _]
            tunnel: w1358 -> [w1378 _]
            tunnel: w1363 -> [w1377 _]
            tunnel: w1362 -> [_ w1388]
            tunnel: w1361 -> [_ w1384]
            frame False {
              n522 = flat-sequence {
                tunnel: w1381 -> [w1382]
                tunnel: [w1382] -> w1380
                frame #0 {
                  n523 = One Button Dialog(message="Please establish RS connection.") -> ()  [unwired: 1 in, 1 out]
                }
              }
              n524 = Increment(x=w1377) -> (x+1=w1376:i32)
              n525 = call "PassOrFail (SubVI).vi"("index (row)"=w1376, "error in (no error)"=w1380, "Pass?Fail"=w1379, "Table in"=w1378) -> ()  [unwired: 7 in, 1 out]
            }
            frame True {
              n526 = control-ref of="Stop Burn-in"() -> (w1390:refnum<vi>)
              n527 = control-ref of="Pannel User Message"() -> (w1392:refnum<vi>)
              n528 = control-ref of="Config_CANAT"() -> (w1386:refnum<vi>)
              n529 = control-ref of="ATR"() -> (w1393:refnum<vi>)
              n530 = control-ref of="Motor Speed RPM"() -> (w1394:refnum<vi>)
              n531 = control-ref of="UUT"() -> (w1385:refnum<vi>)
              n532 = control-ref of="Stop Button"() -> (w1391:refnum<vi>)
              n533 = property on="VISA Tester" class="VISAName"() -> ("Value"=w1387:refnum<visa-resource-name>)  [unwired: 2 in, 2 out]
              n534 = while {
                shift-right: [w1397] -> _
                shift-left: T14."Start" -> [w1407]
                tunnel: w1390 -> [w1406]
                tunnel: w1391 -> [w1405]
                tunnel: w1392 -> [w1404]
                tunnel: w1393 -> [w1403]
                tunnel: w1394 -> [w1402]
                tunnel: w1388 -> [w1401]
                tunnel: w1387 -> [w1400]
                tunnel: w1386 -> [w1399]
                tunnel: w1385 -> [w1398]
                tunnel: w1384 -> [w1395]
                stop <- w1396 stop-if-true
                n535 = case shown="\"Start\"" w1407 {
                  tunnel: w1406 -> [_ w1442 w1469 w1524 w1554]
                  tunnel: w1405 -> [_ w1443 w1461 w1510 w1556]
                  tunnel: w1404 -> [_ w1440 w1470 w1522 w1558]
                  tunnel: w1403 -> [_ w1420 _ _ _]
                  tunnel: w1402 -> [_ w1444 w1468 w1525 w1553]
                  tunnel: w1401 -> [_ w1453 w1473 w1534 w1550]
                  tunnel: w1400 -> [w1410 w1449 w1472 w1530 w1538]
                  tunnel: w1399 -> [_ _ _ _ w1564]
                  tunnel: w1398 -> [_ _ _ _ w1563]
                  tunnel: [w1408 w1429 w1462 w1513 w1541] -> w1397
                  tunnel: [w1409 FALSE FALSE FALSE FALSE] -> w1396
                  tunnel: w1395 -> [_ _ w1471 _ _]
                  frame "Stop", Default {
                    n536 = flat-sequence {
                      tunnel: w1410 -> [w1411]
                      tunnel: [TRUE] -> w1409
                      tunnel: [T14."Stop"] -> w1408
                      frame #0 {
                        n537 = call "TesterOption (SubVI).vi"("2 Options"=FALSE, "On/Off"=FALSE, "Tester Option"=T11."Venable", "VISA Refnum in"=w1411) -> ()  [unwired: 6 in, 2 out]
                      }
                      frame #1 {
                      }
                    }
                  }
                  frame "AO[1]=Meas." {
                    n538 = property on="AO[1]Meas" class="DigNum (strict)"() -> ("Value"=w1423:dbl)  [unwired: 2 in, 2 out]
                    n539 = Number To Fractional String(number=w1423) -> (F-format string=w1431:string)  [unwired: 3 in]
                    n540 = Search and Replace String(input string="EP=1\r\nAO[1]=0\r\n" ("write buffer"), search string="0", replace string=w1431) -> (result string=w1430:string)  [unwired: 5 in, 3 out]
                    n541 = call "SerialMarvinSendGet.vi"("Clear Log"=FALSE, "write buffer"=w1430, "VISA resource name"=w1453) -> ("error out"=w1448:errorcluster)  [unwired: 7 in, 1 out]
                    n542 = call "TesterOption (SubVI).vi"("2 Options"=FALSE, "error in (no error)"=w1448, "On/Off"=FALSE, "Tester Option"=T11."Power", "VISA Refnum in"=w1449) -> ("error out"=w1447:errorcluster, "VISA Refnum out"=w1434:refnum<visa-resource-name>)  [unwired: 5 in]
                    n543 = call "Write panel message (SubVI).vi"("Stop BurnIn"=w1442, 4:"rpm"=w1444, 5:"rpm"=FALSE ("rpm"), "PrintTime"=TRUE, "Stop"=w1443, "error in (no error)"=w1447, "Time to wait"=20.0, "Strin"="2. Temperature sensor calibration test in process...\nSet Parameters...", "String in"=w1440) -> ("error out"=w1435:errorcluster)  [unwired: 2 in]
                    n544 = call "TesterOption (SubVI).vi"("2 Options"=FALSE, "error in (no error)"=w1435, "On/Off"=FALSE, "Tester Option"=T11."Venable", "VISA Refnum in"=w1434) -> ("error out"=w1428:errorcluster)  [unwired: 5 in, 1 out]
                    n545 = flat-sequence {
                      tunnel: [T14."Stop"] -> w1429
                      tunnel: w1421 -> [_]
                      frame #0 {
                      }
                    }
                    n546 = In Range and Coerce(upper limit=0.1, x=w1423, lower limit=-0.1) -> (In Range?=w1418:bool)  [unwired: 1 out]
                    "SensCalResult" <- w1418
                    n547 = call "Find_Number_LineMARVIN.vi"("Test Paragraph"="2.1", "error in"=w1428, "TableIn"=w1420) -> ("error out"=w1422:errorcluster, "Line number"=w1426:i32)  [unwired: 2 in, 2 out]
                    n548 = call "PassOrFail (SubVI).vi"("Test#"="2", "index (row)"=w1426, "error in (no error)"=w1422, "Data in"=w1423, "Pass?Fail"=w1418, "Table in"=w1420) -> ("error out"=w1421:errorcluster)  [unwired: 5 in]
                  }
                  frame "TA[5]" {
                    w1474 = T17 [enum."50C", enum."80C", enum."100C", enum."120C"] items=["K15", "K16", "K17", "Venable", "Firmeware", "Fan", "Power", "120C", "110C", "100C", "90C", "80C", "70C", "60C", "50C", "40C", "30C", "25C", "20C", "10C", "0C"]
                    n549 = for {
                      tunnel: w1474 -> [w1489] mode=indexing
                      tunnel: w1473 -> [w1488]
                      tunnel: w1472 -> [w1487]
                      tunnel: w1471 -> [w1486]
                      tunnel: w1470 -> [w1485]
                      tunnel: w1461 -> [w1484]
                      tunnel: w1469 -> [w1483]
                      tunnel: w1468 -> [w1482]
                      tunnel: dbl[] [0.59774, 0.65238, 0.68545, 0.71584] -> [w1477] mode=indexing
                      tunnel: [w1476] -> w1457 mode=indexing
                      tunnel: [w1475] -> w1460
                      n550 = for {
                        N: 5 -> [_]
                        tunnel: w1489 -> [w1507]
                        tunnel: w1488 -> [w1506]
                        tunnel: w1487 -> [w1502]
                        tunnel: w1486 -> [w1500]
                        tunnel: w1485 -> [w1499]
                        tunnel: w1484 -> [w1498]
                        tunnel: w1483 -> [w1496]
                        tunnel: w1482 -> [w1493]
                        tunnel: [w1492] -> w1481 mode=indexing
                        tunnel: [w1491] -> w1475
                        n551 = call "TesterOption (SubVI).vi"("2 Options"=FALSE, "On/Off"=TRUE, "Tester Option"=w1507, "VISA Refnum in"=w1502) -> ("error out"=w1503:errorcluster)  [unwired: 6 in, 1 out]
                        n552 = call "Write panel message (SubVI).vi"("Stop BurnIn"=w1496, 4:"rpm"=w1493, 5:"rpm"=FALSE ("rpm"), "PrintTime"=FALSE, "Stop"=w1498, "error in (no error)"=w1503, "Time to wait"=1.0, "Strin"=w1500, "String in"=w1499) -> ("error out"=w1501:errorcluster)  [unwired: 2 in]
                        n553 = call "SerialMarvinSendGet.vi"("error in (no error)"=w1501, "write buffer"="TA[5]\r\n", "VISA resource name"=w1506) -> ("error out"=w1491:errorcluster, "read buffer"=w1504:string)  [unwired: 7 in]
                        n554 = Fract/Exp String To Number(string=w1504) -> (number=w1492:dbl)  [unwired: 3 in, 1 out]
                      }
                      n555 = Add Array Elements(numeric array=w1481) -> (sum=w1480:dbl)
                      n556 = Divide(x=w1480, y=5.0) -> (x/y=w1478:dbl)
                      n557 = Subtract(x=w1478, y=w1477) -> (x-y=w1476:dbl)
                    }
                    n558 = property class="Bool (strict)"(reference=w1461, error in=w1460) -> ("Value"=w1466:bool)  [unwired: 2 out]
                    n559 = Select(t=T14."Stop", s=w1466, f=T14."AO[1]=Meas.") -> (s? t:f=w1462:T14)
                    n560 = Array Size(array=w1457) -> (size(s)=w1456:i32)
                    n561 = Add Array Elements(numeric array=w1457) -> (sum=w1459:dbl)
                    n562 = Divide(x=w1459, y=w1456) -> (x/y=→"AO[1]Meas":dbl)
                  }
                  frame "AO[1]=0" {
                    n563 = call "SerialMarvinSendGet.vi"("write buffer"="EP=1\r\nAO[1]=0\r\n", "VISA resource name"=w1534) -> ("error out"=w1529:errorcluster)  [unwired: 8 in, 1 out]
                    n564 = call "TesterOption (SubVI).vi"("2 Options"=FALSE, "error in (no error)"=w1529, "On/Off"=FALSE, "Tester Option"=T11."Power", "VISA Refnum in"=w1530) -> ("error out"=w1528:errorcluster, "VISA Refnum out"=w1516:refnum<visa-resource-name>)  [unwired: 5 in]
                    n565 = call "Write panel message (SubVI).vi"("Stop BurnIn"=w1524, 4:"rpm"=w1525, 5:"rpm"=FALSE ("rpm"), "PrintTime"=TRUE, "Stop"=w1510, "error in (no error)"=w1528, "Time to wait"=20.0, "Strin"="2. Temperature sensor calibration test in process...\nSet Parameters...", "String in"=w1522) -> ("error out"=w1517:errorcluster)  [unwired: 2 in]
                    n566 = call "TesterOption (SubVI).vi"("2 Options"=FALSE, "error in (no error)"=w1517, "On/Off"=FALSE, "Tester Option"=T11."Venable", "VISA Refnum in"=w1516) -> ("error out"=w1511:errorcluster)  [unwired: 5 in, 1 out]
                    n567 = property class="Bool (strict)"(reference=w1510, error in=w1511) -> ("Value"=w1515:bool)  [unwired: 2 out]
                    n568 = Select(t=T14."Stop", s=w1515, f=T14."TA[5]") -> (s? t:f=w1513:T14)
                  }
                  frame "Start" {
                    n569 = call "Write panel message (SubVI).vi"("Stop BurnIn"=w1554, 4:"rpm"=w1553, 5:"rpm"=FALSE ("rpm"), "PrintTime"=FALSE, "Stop"=w1556, "Time to wait"=0.1, "Strin"="2. Temperature sensor calibration test in process...\nInitialization state...", "String in"=w1558) -> ("error out"=w1559:errorcluster)  [unwired: 3 in]
                    n570 = call "TesterOption (SubVI).vi"("2 Options"=FALSE, "error in (no error)"=w1559, "On/Off"=FALSE, "Tester Option"=T11."Venable", "VISA Refnum in"=w1538) -> ("error out"=w1561:errorcluster)  [unwired: 5 in, 1 out]
                    n571 = call "CANSendMotorSpeed.vi"("Remote"=TRUE, "error in (no error)"=w1561, "Motor Speed RPM"=u16 0, "UUT"=w1563, "CAN Cluster in"=w1564) -> ("error out"=w1548:errorcluster)  [unwired: 6 in]
                    n572 = call "SerialMarvinSendGet.vi"("error in (no error)"=w1548, "write buffer"="AO[1]\r\n", "VISA resource name"=w1550) -> ("error out"=w1537:errorcluster, "read buffer"=w1547:string)  [unwired: 7 in]
                    n573 = Equal?(x=w1547, y="0.0") -> (x = y?=w1539:bool)
                    n574 = property class="Bool (strict)"(reference=w1556, error in=w1537) -> ("Value"=w1568:bool)  [unwired: 2 out]
                    n575 = Select(t=T14."TA[5]", s=w1539, f=T14."AO[1]=0") -> (s? t:f=w1543:T14)
                    n576 = Select(t=T14."Stop", s=w1568, f=w1543) -> (s? t:f=w1541:T14)
                  }
                }
              }
            }
          }
        }
        frame "Auxiliary" {
          w1572 = "9. Auxiliary test in process..." ("Value")
          w1584 = "9" ("Test Paragraph")
          n577 = control-ref of="Pannel User Message"() -> (w1583:refnum<vi>)
          n578 = property class="Str"(reference=w1583, error in=w1580, "Value"=w1572) -> (error out=w1582:errorcluster)  [unwired: 1 out]
          n579 = call "Table_ScrollaBarMarvin.vi"("error in"=w1582, "Line to focus"=w1584, "reference in"=w1581) -> ("error out"=w1590:errorcluster)  [unwired: 2 out]
          n580 = property class="Tbl (strict)"(reference=w1581, error in=w1590) -> (reference out=w1579:refnum<vi>, error out=w1589:errorcluster, "Value"=w1588:string[][])
          n581 = Index Array(array=w1588, index (col)=0 ("disabled index (col)")) -> (element=w1587:string[])  [unwired: 1 in]
          n582 = call "Find_Number_Line.vi"("error in"=w1589, "Test Paragraph"=w1584, "Row Headers[]"=w1587) -> ("error out"=w1585:errorcluster, "Line number"=w1570:i32)  [unwired: 1 out]
          n583 = call "Reset old test Values (SubVI).vi"("error in"=w1585, "Atr in"=w1579, "Test Paragraph"=w1584) -> ("error out"=w1577:errorcluster)  [unwired: 8 in]
          n584 = property on="VISA Tester" class="VISAName"() -> ("Value"=w1571:refnum<visa-resource-name>)  [unwired: 2 in, 2 out]
          n585 = control-ref of="Stop Burn-in"() -> (w1574:refnum<vi>)
          n586 = control-ref of="Stop Button"() -> (w1575:refnum<vi>)
          n587 = control-ref of="Pannel User Message"() -> (w1576:refnum<vi>)
          n588 = control-ref of="ATR"() -> (w1569:refnum<vi>)
          n589 = control-ref of="Config_CANAT"() -> ()  [unwired: 1 out]
          n590 = control-ref of="Motor Speed RPM"() -> (w1573:refnum<vi>)
          n591 = while {
            shift-right: [w1595] -> _
            shift-left: enum16{"Stop", "CoolingON", "HotGunON", "Start"}."Start" -> [w1602]
            tunnel: w1577 -> [w1593]
            tunnel: w1576 -> [w1601]
            tunnel: w1575 -> [w1600]
            tunnel: w1574 -> [w1599]
            tunnel: w1573 -> [w1598]
            tunnel: w1572 -> [w1597]
            tunnel: w1571 -> [w1596]
            tunnel: w1570 -> [w1592]
            tunnel: w1569 -> [w1591]
            stop <- w1594 stop-if-true
            n592 = case shown="\"CoolingON\"" w1602 {
              tunnel: w1601 -> [_ w1647 w1742 w1802]
              tunnel: w1600 -> [_ w1642 w1737 w1788]
              tunnel: w1599 -> [_ w1646 w1741 w1801]
              tunnel: w1598 -> [_ w1645 w1740 w1797]
              tunnel: w1597 -> [_ w1636 w1731 w1796]
              tunnel: w1596 -> [_ w1637 w1732 w1789]
              tunnel: [w1604 w1639 w1734 w1784] -> w1595
              tunnel: [w1603 FALSE FALSE FALSE] -> w1594
              tunnel: w1593 -> [_ w1635 w1730 _]
              tunnel: w1592 -> [_ w1630 w1725 _]
              tunnel: w1591 -> [_ w1626 w1722 _]
              frame "Stop", Default {
                n593 = flat-sequence {
                  tunnel: [enum16{"Stop", "CoolingON", "HotGunON", "Start"}."Stop"] -> w1604
                  tunnel: [TRUE] -> w1603
                  frame #0 {
                    n594 = property on="VISA Tester" class="VISAName"() -> ("Value"=w1608:refnum<visa-resource-name>)  [unwired: 2 in, 2 out]
                    n595 = call "TesterOption (SubVI).vi"("2 Options"=FALSE, "On/Off"=FALSE, "Tester Option"=T11."Venable", "VISA Refnum in"=w1608) -> ()  [unwired: 6 in, 2 out]
                  }
                  frame #1 {
                  }
                }
              }
              frame "CoolingON" {
                n596 = while {
                  tunnel: w1647 -> [w1682]
                  tunnel: w1646 -> [w1681]
                  tunnel: w1645 -> [w1677]
                  tunnel: [w1674] -> w1615
                  tunnel: w1642 -> [w1665]
                  tunnel: w1637 -> [w1651]
                  tunnel: w1636 -> [w1669]
                  tunnel: w1635 -> [w1666]
                  shift-right: [w1658] -> _
                  shift-left: 0.0 -> [w1659]
                  shift-right: [w1654] -> w1614
                  shift-left: 0.0 ("Value") -> [w1656]
                  tunnel: [w1649] -> w1618
                  stop <- w1663 stop-if-true
                  n597 = control-ref of="Power transistor Heat sink Temp."() -> (w1675:refnum<vi>)
                  n598 = property class="DigNum (strict)"(reference=w1675, error in=w1666) -> (error out=w1672:errorcluster, "Value"=w1654:dbl)  [unwired: 1 out]
                  n599 = Equal?(x=w1654, y=w1656) -> (x = y?=w1655:bool)
                  n600 = Number To Fractional String(number=w1654, precision (6)=i16 2) -> (F-format string=w1668:string)  [unwired: 2 in]
                  n601 = case shown="True" w1655 {
                    tunnel: w1659 -> [_ w1702]
                    tunnel: [0.0 w1700] -> w1658
                    tunnel: [FALSE w1699] -> w1657
                    frame False {
                    }
                    frame True {
                      n602 = Increment(x=w1702) -> (x+1=w1700:dbl)
                      n603 = Greater Or Equal?(x=w1700, y=300.0) -> (x >= y?=w1699:bool)
                    }
                  }
                  n604 = Concatenate Strings(w1669, "\nPCB Temperature [C]: " ("string"), w1668) -> (w1667:string)
                  n605 = call "Write panel message (SubVI).vi"("Stop BurnIn"=w1681, 4:"rpm"=w1677, 5:"rpm"=FALSE ("rpm"), "PrintTime"=FALSE, "Stop"=w1665, "error in (no error)"=w1672, "Time to wait"=0.2, "Strin"=w1667, "String in"=w1682) -> ("error out"=w1671:errorcluster)  [unwired: 2 in]
                  n606 = property class="Bool (strict)"(reference=w1665) -> ("Value"=w1664:bool)  [unwired: 1 in, 2 out]
                  n607 = Less Or Equal?(x=w1654, y=52.0) -> (x <= y?=w1653:bool)
                  n608 = call "GetADCTester (SubVI).vi"("error in (no error)"=w1671, "GetADCTester"=T13."Fan", "VISA Refnum in"=w1651) -> ("error out"=w1674:errorcluster, "ADCValOutput Single"=w1661:dbl)  [unwired: 6 in, 1 out]
                  n609 = Greater?(x=w1661, y=u32 2400) -> (0:w1650:bool)
                  n610 = case shown="True" w1653 {
                    tunnel: [w1689 w1696] -> w1652
                    tunnel: w1653 -> [w1689 w1696]
                    tunnel: w1651 -> [w1687 w1694]
                    tunnel: [w1683 w1690] -> w1649
                    frame False {
                      n611 = call "Time Delay11"() -> ("error out"=w1686:errorcluster)  [unwired: 11 in]
                      n612 = call "GetADCTester (SubVI).vi"("error in (no error)"=w1686, "GetADCTester"=T13."Fan", "VISA Refnum in"=w1687) -> ("ADCValOutput Single"=w1685:dbl)  [unwired: 6 in, 2 out]
                      n613 = Greater?(x=w1685, y=2400.0) -> (0:w1683:bool)
                    }
                    frame True {
                      n614 = call "Time Delay10"() -> ("error out"=w1693:errorcluster)  [unwired: 11 in]
                      n615 = call "GetADCTester (SubVI).vi"("error in (no error)"=w1693, "GetADCTester"=T13."Fan", "VISA Refnum in"=w1694) -> ("ADCValOutput Single"=w1692:dbl)  [unwired: 6 in, 2 out]
                      n616 = Greater?(x=w1692, y=2400.0) -> (0:w1690:bool)
                    }
                  }
                  n617 = Compound Arithmetic op=OR(w1650, w1664, w1652, w1657) -> (w1663:bool)
                }
                n618 = In Range and Coerce(upper limit=56.0, x=w1614, lower limit=52.0) -> (In Range?=w1617:bool)  [unwired: 1 out]
                n619 = Build Array(w1618, w1617) -> (w1619:bool[])
                n620 = And Array Elements(Boolean array=w1619) -> (logical AND=→"AuxiOFFResult":bool)
                n621 = Add(x=w1630, y=3) -> (x+y=w1628:i32)
                n622 = call "PassOrFail (SubVI).vi"("index (row)"=w1628, "error in (no error)"=w1615, "Data in"=w1614, "Pass?Fail"=w1617, "Table in"=w1626) -> ("error out"=w1632:errorcluster)  [unwired: 6 in]
                n623 = Select(t="OFF", s=w1618, f="ON") -> (s? t:f=w1622:string)
                n624 = Increment(x=w1628) -> (x+1=w1627:i32)
                n625 = call "PassOrFail (SubVI).vi"("String Res"=w1622, "index (row)"=w1627, "error in (no error)"=w1632, "Data in"=-3.0, "Pass?Fail"=w1618, "Table in"=w1626) -> ("error out"=w1631:errorcluster)  [unwired: 5 in]
                n626 = call "TesterOption (SubVI).vi"("2 Options"=FALSE, "error in (no error)"=w1631, "On/Off"=FALSE, "Tester Option"=T11."Venable" ("Tester Option 2"), "VISA Refnum in"=w1637) -> ("error out"=w1612:errorcluster)  [unwired: 5 in, 1 out]
                n627 = call "Time Delay14"("error in (no error)"=w1612) -> ("error out"=w1611:errorcluster)  [unwired: 10 in]
                n628 = property class="Bool (strict)"(reference=w1642, error in=w1611) -> ("Value"=w1648:bool)  [unwired: 2 out]
                n629 = Select(t=enum16{"Stop", "CoolingON", "HotGunON", "Start"}."Stop", s=w1648, f=enum16{"Stop", "CoolingON", "HotGunON", "Start"}."Stop") -> (s? t:f=w1639:enum16{"Stop", "CoolingON", "HotGunON", "Start"})
              }
              frame "HotGunON" {
                n630 = while {
                  tunnel: w1742 -> [w1775]
                  tunnel: w1741 -> [w1774]
                  tunnel: w1740 -> [w1770]
                  tunnel: [w1766] -> w1712
                  tunnel: w1737 -> [w1757]
                  tunnel: w1732 -> [w1767]
                  tunnel: w1731 -> [w1761]
                  tunnel: w1730 -> [w1758]
                  shift-right: [w1750] -> _
                  shift-left: 0.0 -> [w1751]
                  shift-right: [w1747] -> _
                  shift-left: 0.0 ("Value") -> [w1748]
                  tunnel: [w1745] -> w1710
                  stop <- w1755 stop-if-true
                  n631 = control-ref of="Power transistor Heat sink Temp."() -> (w1768:refnum<vi>)
                  n632 = property class="DigNum (strict)"(reference=w1768, error in=w1758) -> (error out=w1764:errorcluster, "Value"=w1747:dbl)  [unwired: 1 out]
                  n633 = Equal?(x=w1747, y=w1748) -> (x = y?=w1746:bool)
                  n634 = Number To Fractional String(number=w1747, precision (6)=i16 2) -> (F-format string=w1760:string)  [unwired: 2 in]
                  n635 = case shown="True" w1746 {
                    tunnel: w1751 -> [_ w1781]
                    tunnel: [0.0 w1779] -> w1750
                    tunnel: [FALSE w1778] -> w1749
                    frame False {
                    }
                    frame True {
                      n636 = Increment(x=w1781) -> (x+1=w1779:dbl)
                      n637 = Greater Or Equal?(x=w1779, y=300.0) -> (x >= y?=w1778:bool)
                    }
                  }
                  n638 = Concatenate Strings(w1761, "\nPCB Temperature [C]: " ("string"), w1760) -> (w1759:string)
                  n639 = call "Write panel message (SubVI).vi"("Stop BurnIn"=w1774, 4:"rpm"=w1770, 5:"rpm"=FALSE ("rpm"), "PrintTime"=FALSE, "Stop"=w1757, "error in (no error)"=w1764, "Time to wait"=0.2, "Strin"=w1759, "String in"=w1775) -> ("error out"=w1763:errorcluster)  [unwired: 2 in]
                  n640 = property class="Bool (strict)"(reference=w1757) -> ("Value"=w1756:bool)  [unwired: 1 in, 2 out]
                  n641 = call "GetADCTester (SubVI).vi"("error in (no error)"=w1763, "GetADCTester"=T13."Fan", "VISA Refnum in"=w1767) -> ("error out"=w1766:errorcluster, "ADCValOutput Single"=w1753:dbl)  [unwired: 6 in, 1 out]
                  n642 = Greater Or Equal?(x=w1747, y=61.0) -> (x >= y?=w1744:bool)
                  n643 = Less?(x=w1753, y=u32 100) -> (x < y?=w1745:bool)
                  n644 = Compound Arithmetic op=OR(w1745, w1756, w1744, w1749) -> (w1755:bool)
                }
                n645 = control-ref of="Power transistor Heat sink Temp."() -> (w1715:refnum<vi>)
                n646 = property class="DigNum (strict)"(reference=w1715, error in=w1712) -> (error out=w1714:errorcluster, "Value"=w1713:dbl)  [unwired: 1 out]
                n647 = In Range and Coerce(upper limit=62.0, x=w1713, lower limit=58.0) -> (In Range?=w1709:bool)  [unwired: 1 out]
                n648 = Build Array(w1710, w1709) -> (w1711:bool[])
                n649 = Increment(x=w1725) -> (x+1=w1724:i32)
                n650 = call "PassOrFail (SubVI).vi"("index (row)"=w1724, "error in (no error)"=w1714, "Data in"=w1713, "Pass?Fail"=w1709, "Table in"=w1722) -> ("error out"=w1727:errorcluster)  [unwired: 6 in]
                n651 = And Array Elements(Boolean array=w1711) -> (logical AND=→"AuxiONResult":bool)
                n652 = Increment(x=w1724) -> (x+1=w1723:i32)
                n653 = Select(t="ON", s=w1710, f="OFF") -> (s? t:f=w1720:string)
                n654 = call "PassOrFail (SubVI).vi"("String Res"=w1720, "index (row)"=w1723, "error in (no error)"=w1727, "Data in"=-3.0, "Pass?Fail"=w1710, "Table in"=w1722) -> ("error out"=w1726:errorcluster)  [unwired: 5 in]
                n655 = call "TesterOption (SubVI).vi"("On/Off 2"=FALSE, "Tester Option 2"=T11."Venable", "2 Options"=TRUE, "error in (no error)"=w1726, "On/Off"=FALSE, "Tester Option"=T11."Fan", "VISA Refnum in"=w1732) -> ("error out"=w1704:errorcluster)  [unwired: 3 in, 1 out]
                n656 = call "Time Delay13"("error in (no error)"=w1704) -> ("error out"=w1703:errorcluster)  [unwired: 10 in]
                n657 = property class="Bool (strict)"(reference=w1737, error in=w1703) -> ("Value"=w1743:bool)  [unwired: 2 out]
                n658 = Select(t=enum16{"Stop", "CoolingON", "HotGunON", "Start"}."Stop", s=w1743, f=enum16{"Stop", "CoolingON", "HotGunON", "Start"}."CoolingON") -> (s? t:f=w1734:enum16{"Stop", "CoolingON", "HotGunON", "Start"})
              }
              frame "Start" {
                n659 = call "Write panel message (SubVI).vi"("Stop BurnIn"=w1801, 4:"rpm"=w1797, 5:"rpm"=FALSE ("rpm"), "PrintTime"=TRUE, "Stop"=w1788, "Time to wait"=3.0, "Strin"=w1796, "String in"=w1802) -> ("error out"=w1795:errorcluster)  [unwired: 3 in]
                n660 = call "TesterOption (SubVI).vi"("On/Off 2"=TRUE, "Tester Option 2"=T11."Fan", "2 Options"=TRUE, "error in (no error)"=w1795, "On/Off"=FALSE, "Tester Option"=T11."Venable", "VISA Refnum in"=w1789) -> ("error out"=w1787:errorcluster)  [unwired: 3 in, 1 out]
                n661 = call "Time Delay"("error in (no error)"=w1787) -> ("error out"=w1782:errorcluster)  [unwired: 10 in]
                n662 = property class="Bool (strict)"(reference=w1788, error in=w1782) -> ("Value"=w1803:bool)  [unwired: 2 out]
                n663 = Select(t=enum16{"Stop", "CoolingON", "HotGunON", "Start"}."Stop", s=w1803, f=enum16{"Stop", "CoolingON", "HotGunON", "Start"}."HotGunON") -> (s? t:f=w1784:enum16{"Stop", "CoolingON", "HotGunON", "Start"})
              }
            }
          }
        }
      }
    }
    n664 = flat-sequence {
      tunnel: w183 -> [_]
      frame #0 {
        w191 = T19."Enabled" ("Disabled")
        w192 = FALSE ("Start")
        n665 = property on="Start" class="Bool (strict)"("Value"=w192, "DisabledEnum"=w191) -> ()  [unwired: 2 in, 2 out]
        n666 = property on="Report" class="Bool (strict)"("Value"=w192, "DisabledEnum"=w191) -> ()  [unwired: 2 in, 2 out]
      }
    }
  }
  n667 = while {
    shift-right: [w1822] -> _
    shift-left: T10."Initialize" -> [w1821]
    shift-right: [w1818] -> _
    shift-left: _ -> [w1817]
    shift-right: [w1816] -> _
    shift-left: w20 -> [w1814]
    shift-right: [w1815] -> _
    shift-left: refnum<vi> refnum ("Config_CANAT") -> [w1813]
    shift-right: [w1811] -> _
    shift-left: w17 -> [w1812]
    tunnel: "ATR" -> [_]
    tunnel: w8 -> [w1810]
    tunnel: w7 -> [w1809]
    shift-right: [w1807] -> _
    shift-left: 0 -> [w1808]
    tunnel: w5 -> [w1806]
    tunnel: w3 -> [w1805]
    tunnel: w2 -> [_]
    tunnel: w18 -> [w1820]
    tunnel: [w1819] -> _
    stop <- w1804 stop-if-true
    n668 = case shown="\"MainProgram\"" w1821 {
      tunnel: [T10."MainProgram" w1925 w1995 T10."Erase ATR Table"] -> w1822
      tunnel: [FALSE w1911 FALSE FALSE] -> w1804
      tunnel: [w1829 w1916 w1989 w2833] -> w1819
      tunnel: w1820 -> [_ w1936 w1993 _]
      tunnel: [w1866 refnum<visa-resource-name> refnum ("VISA resource name") w1990 w2838] -> w1818
      tunnel: w1817 -> [w1866 w1944 w1991 _]
      tunnel: [w1856 w1905 w1985 w2831] -> w1816
      tunnel: [w1855 refnum<vi> refnum ("Config_CANAT") w1986 w2834] -> w1815
      tunnel: w1814 -> [w1856 w1946 w1988 w2831]
      tunnel: w1813 -> [w1855 w1928 w1987 _]
      tunnel: w1812 -> [w1854 w1939 w1984 w2830]
      tunnel: [w1854 w1904 w1983 w2830] -> w1811
      tunnel: w1810 -> [_ _ w1982 _]
      tunnel: w1809 -> [_ _ w1981 _]
      tunnel: w1808 -> [w1843 w1930 w1980 w2827]
      tunnel: [w1843 w1930 w1979 w2827] -> w1807
      tunnel: w1806 -> [w1833 _ w1978 _]
      tunnel: w1805 -> [_ _ w1977 _]
      frame "Erase ATR Table", Default {
        w1837 = "Marvin" ("section")
        w1850 = refnum<visa-resource-name> "COM4" ("VISA resource name")
        w1861 = FALSE ("Visible")
        n669 = property on="Serial Com" class="Bool"(error in=errorcluster {"status"=FALSE, "code"=0, "source"=""} ("error out"), "Visible"=TRUE) -> (error out=w1851:errorcluster)  [unwired: 1 in, 1 out]
        n670 = property on="VISA Marvin" class="VISAName"(error in=w1851, "Visible"=w1861, "Value"=w1850) -> (error out=w1863:errorcluster)  [unwired: 1 in, 1 out]
        n671 = property on="VISA Marvin" class="VISAName"(error in=w1851, "Value"=w1850) -> ()  [unwired: 1 in, 2 out]
        n672 = property on="Status" class="Bool (strict)"(error in=w1863, "Value"=w1861) -> (error out=w1825:errorcluster)  [unwired: 1 in, 1 out]
        n673 = call "Select UUT"("error in (no error)"=w1825) -> ("EBAY"=w1823:bool, "error out"=w1824:errorcluster)  [unwired: 17 in]
        n674 = case shown="True" w1823 {
          tunnel: [string[][] [["1", "Communication Test", "", "", "", "", ""], ["1.1", "Serial RS-232", "N/A", "-", "", "", ""], ["1.2", "CAN Bus", "N/A", "-", "", "", ""], ["", "", "", "", "", "", ""], ["2", "Temperature Sensor Calibration", "", "", "", "", ""], ["2.1", "Sensor Reading Analog Offset", "0", "+/-0.100", ".", "", ""], ["", "", "", "", "", "", ""], ["3", "Motor Termistor Input Test", "", "", "", "", ""], ["3.1", "60 Degree", "60", "+/-3.00", "C", "", ""], ["3.2", "90 Degree", "90", "+/-3.00", "C", "", ""], ["3.3", "120 Degree", "120", "+/-3.00", "C", "", ""], ["", "", "", "", "", "", ""], ["4", "Enable Test", "", "", "", "", ""], ["4.1", "Fan Speed at Opened Enable ", "5000", "+/-200.0", "rpm", "", ""], ["4.2", "Fan Speed at Opened Enable ", "0", "+/-200.0", "rpm", "", ""], ["4.3", "Fan Speed at Closed Enable ", "5000", "+/-200.0", "rpm", "", ""], ["4.4", "Motor Rotation Direction", "Counter-clockwise (Inlet)", "-", "", "", ""], ["", "", "", "", "", "", ""], ["5", "Speed Command Test", "", "", "", "", ""], ["5.1", "Fan Speed", "6000", "+/-200.0", "rpm", "", ""], ["5.2", "Fan Speed", "9000", "+/-200.0", "rpm", "", ""], ["5.3", "Fan Speed", "12100", "+/-200.0", "rpm", "", ""], ["", "", "", "", "", "", ""], ["6", "Motor Stop time", "< 50", "-", "sec", "", ""], ["", "", "", "", "", "", ""], ["7", "Burn-in Test", "", "", "", "", ""], ["7.1", "DC Input Current", "28", "+/-5.000", "A", "", ""], ["7.2", "Fan Speed", "12100", "+/-200.0", "rpm", "", ""], ["7.3", "Ambient Temperature", "25", "+/-13.00", "C", "", ""], ["7.4", "After 10 min of operation", "", "-", "C", "", ""], ["7.5", "After 20 min of operation", "", "-", "C", "", ""], ["7.6", "After 30 min of operation", "", "-", "C", "", ""], ["", "", "", "", "", "", ""], ["8", "Visual Inspection", "", "", "", "", ""], ["8.1", "Verification of Components Not Installed", "N/A", "-", "", "", ""], ["8.2", "Manufacturing Defects", "N/A", "-", "", "", ""], ["", "", "", "", "", "", ""], ["9", "Power Supply Testing", "", "", "", "", ""], ["9.1", "Input Current Drawn", "", "", "", "", ""], ["9.2", "DC Input Current", "< 150", "-", "mA", "", ""], ["", "", "", "", "", "", ""], ["10", "Power Supply Voltages", "", "", "", "", ""], ["10.1", "12V", "12.0", "+/-0.500", "V", "", ""], ["10.2", "5V", "5.0", "+/-0.200", "V", "", ""], ["10.3", "3.3V", "3.3", "+/-0.100", "V", "", ""], ["10.4", "1.8V", "1.8", "+/-0.100", "V", "", ""], ["", "", "", "", "", "", ""], ["11", "Reverse Polarity Test - DC Input Current", "< 1", "-", "mA", "", ""], ["", "", "", "", "", "", ""], ["12", "Functional Test Procedure", "", "", "", "", ""], ["12.1", "Weight Check", "4180", "+/-10.00", "gr", "", ""], ["", "", "", "", "", "", ""], ["13", "Insulation Resistance Test", "", "", "", "", ""], ["13.1", "J3.B to Chassis", "> 1M", "-", "W", "", ""], ["13.2", "J1.16 to Chassis", "> 100K", "-", "W", "", ""], ["", "", "", "", "", "", ""], ["14", "Bonding Resistance", "", "", "", "", ""], ["14.1", "J1 Body to Chassis", "< 2m", "-", "W", "", ""], ["14.2", "J2  Body to Chassis", "< 2m", "-", "W", "", ""], ["14.3", "J3  Body to Chassis", "< 2m", "-", "W", "", ""], ["", "", "", "", "", "", ""], ["15", "CANbus Resistance Test", "", "", "", "", ""], ["15.1", "J1.17 to J1.18", "> 10K", "-", "W", "", ""], ["", "", "", "", "", "", ""], ["16", "Sealing Test", "N/A", "-", "", "", ""]] ("ArrAHU 2") string[][] [["1", "Communication Test", "", "", "", "", ""], ["1.1", "Serial RS-232", "N/A", "-", "", "", ""], ["1.2", "CAN Bus", "N/A", "-", "", "", ""], ["", "", "", "", "", "", ""], ["2", "Temperature Sensor Calibration", "", "", "", "", ""], ["2.1", "Sensor Reading Analog Offset", "0", "+/-0.100", ".", "", ""], ["", "", "", "", "", "", ""], ["3", "Motor Termistor Input Test", "", "", "", "", ""], ["3.1", "60 Degree", "60", "+/-3.00", "C", "", ""], ["3.2", "90 Degree", "90", "+/-3.00", "C", "", ""], ["3.3", "120 Degree", "120", "+/-3.00", "C", "", ""], ["", "", "", "", "", "", ""], ["4", "Enable Test", "", "", "", "", ""], ["4.1", "Fan Speed at Opened Enable ", "5000", "+/-200.0", "rpm", "", ""], ["4.2", "Fan Speed at Opened Enable ", "0", "+/-200.0", "rpm", "", ""], ["4.3", "Fan Speed at Closed Enable ", "5000", "+/-200.0", "rpm", "", ""], ["4.4", "Motor Rotation Direction", "Counter-clockwise (Inlet)", "-", "", "", ""], ["", "", "", "", "", "", ""], ["5", "Speed Command Test", "", "", "", "", ""], ["5.1", "Fan Speed", "6000", "+/-200.0", "rpm", "", ""], ["5.2", "Fan Speed", "11500", "+/-200.0", "rpm", "", ""], ["5.3", "Fan Speed", "15100", "+/-200.0", "rpm", "", ""], ["", "", "", "", "", "", ""], ["6", "Motor Stop time", "< 50", "-", "sec", "", ""], ["", "", "", "", "", "", ""], ["7", "Temperature Control Algorithm Test", "", "", "", "", ""], ["7.1", "Tair <   68 ± 2 oC", "6000", "+/-200.0", "rpm", "", ""], ["7.2", "Measured Temp.", "", "", "C", "", ""], ["7.3", "Tair >= 68 ± 2 oC", "11500", "+/-200.0", "rpm", "", ""], ["7.4", "Transition Temp.", "", "", "C", "", ""], ["7.5", "Tair >= 88 ± 2 oC", "15100", "+/-400.0", "rpm", "", ""], ["7.6", "Transition Temp.", "", "", "C", "", ""], ["7.7", "Tair <= 80 ± 2 oC", "11500", "+/-200.0", "rpm", "", ""], ["7.8", "Transition Temp.", "", "", "C", "", ""], ["7.9", "Tair <= 60 ± 2 oC", "6000", "+/-200.0", "rpm", "", ""], ["7.10", "Transition Temp.", "", "", "C", "", ""], ["", "", "", "", "", "", ""], ["8", "Burn-in Test", "", "", "", "", ""], ["8.1", "DC Input Current", "50", "+/-5.000", "A", "", ""], ["8.2", "Fan Speed", "15100", "+/-200.0", "rpm", "", ""], ["8.3", "Ambient Temperature", "25", "+/-13.00", "C", "", ""], ["8.4", "After 10 min of operation", "", "-", "C", "", ""], ["8.5", "After 20 min of operation", "", "-", "C", "", ""], ["8.6", "After 30 min of operation", "", "-", "C", "", ""], ["", "", "", "", "", "", ""], ["9", "Auxiliary Fan Test", "", "", "", "", ""], ["9.1", "Auxiliary Cooling Fan ON", "60", "+/-2.00", "C", "", ""], ["9.2", "Fan status", "ON", "-", "-", "", ""], ["9.3", "Auxiliary Cooling Fan OFF", "54", "+/-2.00", "C", "", ""], ["9.4", "Fan status", "OFF", "-", "-", "", ""], ["", "", "", "", "", "", ""], ["10", "Visual Inspection", "", "", "", "", ""], ["10.1", "Verification of Components Not Installed", "N/A", "-", "", "", ""], ["10.2", "Manufacturing Defects", "N/A", "-", "", "", ""], ["", "", "", "", "", "", ""], ["11", "Power Supply Testing", "", "", "", "", ""], ["11.1", "Input Current Drawn", "", "", "", "", ""], ["11.2", "DC Input Current", "< 150", "-", "mA", "", ""], ["", "", "", "", "", "", ""], ["12", "Power Supply Voltages", "", "", "", "", ""], ["12.1", "12V", "12.0", "+/-0.500", "V", "", ""], ["12.2", "5V", "5.0", "+/-0.200", "V", "", ""], ["12.3", "3.3V", "3.3", "+/-0.100", "V", "", ""], ["12.4", "1.8V", "1.8", "+/-0.100", "V", "", ""], ["", "", "", "", "", "", ""], ["13", "Reverse Polarity Test - DC Input Current", "< 1", "-", "mA", "", ""], ["", "", "", "", "", "", ""], ["14", "Functional Test Procedure", "", "", "", "", ""], ["14.1", "Weight Check", "4180", "+/-10.00", "gr", "", ""], ["", "", "", "", "", "", ""], ["15", "Insulation Resistance Test", "", "", "", "", ""], ["15.1", "J3.B to Chassis", "> 1M", "-", "W", "", ""], ["15.2", "J1.16 to Chassis", "> 100K", "-", "W", "", ""], ["", "", "", "", "", "", ""], ["16", "Bonding Resistance", "", "", "", "", ""], ["16.1", "J1 Body to Chassis", "< 2m", "-", "W", "", ""], ["16.2", "J2  Body to Chassis", "< 2m", "-", "W", "", ""], ["16.3", "J3  Body to Chassis", "< 2m", "-", "W", "", ""], ["", "", "", "", "", "", ""], ["17", "CANbus Resistance Test", "", "", "", "", ""], ["17.1", "J1.17 to J1.18", "> 10K", "-", "W", "", ""], ["", "", "", "", "", "", ""], ["18", "Sealing Test", "N/A", "-", "", "", ""]] ("ArrEbay 2")] -> w1859
          tunnel: ["AHU" "EBAY"] -> w1858
          tunnel: [w1876 w1888] -> w1857
          tunnel: w1824 -> [w1877 w1888]
          tunnel: [w1872 u8 95] -> w1830
          frame False {
            (unwired) string[][] [["6.1", "Visual Inspection", "", "", "", "", ""], ["6.1.1", "Verification of Components Not Installed", "N/A", "-", "", "", ""], ["", "", "", "", "", "", ""], ["6.1.2", "Manufacturing Defects", "N/A", "-", "", "", ""], ["", "", "", "", "", "", ""], ["6.2", "Power Supply Testing", "", "", "", "", ""], ["6.2.1", "Input Current Drawn", "", "", "", "", ""], ["6.2.1.1", "DC Input Current", "< 150", "-", "mA", "", ""], ["", "", "", "", "", "", ""], ["6.2.2", "Power Supply Voltages", "", "", "", "", ""], ["6.2.2.1", "12V", "12.0", "+/-0.500", "V", "", ""], ["6.2.2.2", "5V", "5.0", "+/-0.200", "V", "", ""], ["6.2.2.3", "3.3V", "3.3", "+/-0.100", "V", "", ""], ["6.2.2.4", "1.8V", "1.8", "+/-0.100", "V", "", ""], ["", "", "", "", "", "", ""], ["7", "Functional Test Procedure", "", "", "", "", ""], ["7.1", "Weight Check", "3800", "+/-100.0", "gr", "", ""], ["", "", "", "", "", "", ""], ["7.2", "Insulation Resistance Test", "", "", "", "", ""], ["7.2.1", "J3.B to Chassis", "> 1M", "-", "W", "", ""], ["7.2.2", "J1.16 to Chassis", "> 100K", "-", "W", "", ""], ["", "", "", "", "", "", ""], ["7.2", "Bonding Resistance", "", "", "", "", ""], ["7.2.3", "J1 Body to Chassis", "< 2m", "-", "W", "", ""], ["7.2.4", "J2  Body to Chassis", "< 2m", "-", "W", "", ""], ["7.2.5", "J3  Body to Chassis", "< 2m", "-", "W", "", ""], ["", "", "", "", "", "", ""], ["7.2.1", "CANbus Resistance Test", "", "", "", "", ""], ["7.2.1.1", "J1.17 to J1.18", "> 10K", "-", "W", "", ""], ["", "", "", "", "", "", ""], ["7.3", "Sealing Test", "N/A", "-", "", "", ""], ["", "", "", "", "", "", ""], ["7.4", "Communication Test", "", "", "", "", ""], ["7.4.1", "Serial RS-232", "N/A", "-", "", "", ""], ["7.4.2", "CAN Bus", "N/A", "-", "", "", ""], ["", "", "", "", "", "", ""], ["7.5", "Performances Tests", "", "", "", "", ""], ["7.5.1", "Reverse Polarity Test", "", "", "", "", ""], ["7.5.1.1", "DC Input Current", "< 1", "-", "mA", "", ""], ["", "", "", "", "", "", ""], ["7.5.2", "Enable Test", "", "", "", "", ""], ["7.5.2.1", "Fan Speed at Opened Enable ", "5000", "+/-200.0", "rpm", "", ""], ["7.5.2.2", "Fan Speed at Opened Enable ", "0", "+/-200.0", "rpm", "", ""], ["7.5.2.3", "Fan Speed at Closed Enable ", "5000", "+/-200.0", "rpm", "", ""], ["7.5.2.4", "Motor Rotation Direction", "Counter-clockwise (Inlet)", "-", "", "", ""], ["", "", "", "", "", "", ""], ["7.5.3", "Stop Time Test ", "", "", "", "", ""], ["7.5.3.1", "Motor Stop time", "< 50", "-", "sec", "", ""], ["", "", "", "", "", "", ""], ["7.5.4", "Speed Command Test", "", "", "", "", ""], ["7.5.4.1", "Fan Speed", "6000", "+/-200.0", "rpm", "", ""], ["7.5.4.2", "Fan Speed", "9000", "+/-200.0", "rpm", "", ""], ["7.5.4.3", "Fan Speed", "12100", "+/-200.0", "rpm", "", ""], ["", "", "", "", "", "", ""], ["7.5.5", "Temperature Sensor Calibration Test", "", "", "", "", ""], ["7.5.5.1", "Sensor Reading Analog Offset", "0", "+/-0.100", ".", "", ""], ["", "", "", "", "", "", ""], ["7.5.6", "Burn-in Test", "", "", "", "", ""], ["7.5.6.1", "DC Input Current", "28", "+/-3.000", "A", "", ""], ["7.5.6.2", "Fan Speed", "12100", "+/-200.000", "rpm", "", ""], ["7.5.6.3", "Ambient Temperature", "25", "+/-13.00", "C", "", ""], ["7.5.6.4", "After 10 min of operation", "", "", "C", "", ""], ["7.5.6.5", "After 20 min of operation", "", "", "C", "", ""], ["7.5.6.6", "After 30 min of operation", "", "", "C", "", ""], ["", "", "", "", "", "", ""], ["9", "Motor Temp Test", "", "", "", "", ""], ["9.1", "60 C", "60", "+/-3.000", "C", "", ""], ["9.2", "90 C", "90", "+/-3.000", "C", "", ""], ["9.3", "120 C", "120", "+/-3.000", "C", "", ""]] ("data")
            n675 = while {
              shift-right: [w1884] -> w1876
              shift-left: w1877 -> [w1885]
              tunnel: [w1879] -> w1875
              stop <- w1883 stop-if-true
              n676 = call "AHU UUT (subVI).vi"("error in (no error)"=w1885) -> ("AHU 47"=w1880:bool, "AHU 63"=w1879:bool, "OK"=w1882:bool, "error out"=w1884:errorcluster)  [unwired: 15 in]
              n677 = Exclusive Or(1:w1880, 2:w1879) -> (0:w1881:bool)
              n678 = And(x=w1882, y=w1881) -> (x .and. y?=w1883:bool)
            }
            n679 = Select(t=u8 63, s=w1875, f=u8 47) -> (s? t:f=w1872:u8)
          }
          frame True {
            (unwired) string[][] [["6.1", "Visual Inspection", "", "", "", "", ""], ["6.1.1", "Verification of Components Not Installed", "N/A", "-", "", "", ""], ["", "", "", "", "", "", ""], ["6.1.2", "Manufacturing Defects", "N/A", "-", "", "", ""], ["", "", "", "", "", "", ""], ["6.2", "Power Supply Testing", "", "", "", "", ""], ["6.2.1", "Input Current Drawn", "", "", "", "", ""], ["6.2.1.1", "DC Input Current", "< 150", "-", "mA", "", ""], ["", "", "", "", "", "", ""], ["6.2.2", "Power Supply Voltages", "", "", "", "", ""], ["6.2.2.1", "12V", "12.0", "+/-0.500", "V", "", ""], ["6.2.2.2", "5V", "5.0", "+/-0.200", "V", "", ""], ["6.2.2.3", "3.3V", "3.3", "+/-0.100", "V", "", ""], ["6.2.2.4", "1.8V", "1.8", "+/-0.100", "V", "", ""], ["", "", "", "", "", "", ""], ["7", "Functional Test Procedure", "", "", "", "", ""], ["7.1", "Weight Check", "4180", "+/-10.00", "gr", "", ""], ["", "", "", "", "", "", ""], ["7.2", "Insulation Resistance Test", "", "", "", "", ""], ["7.2.1", "J3.B to Chassis", "> 1M", "-", "W", "", ""], ["7.2.2", "J1.16 to Chassis", "> 100K", "-", "W", "", ""], ["", "", "", "", "", "", ""], ["7.2", "Bonding Resistance", "", "", "", "", ""], ["7.2.3", "J1 Body to Chassis", "< 2m", "-", "W", "", ""], ["7.2.4", "J2  Body to Chassis", "< 2m", "-", "W", "", ""], ["7.2.5", "J3  Body to Chassis", "< 2m", "-", "W", "", ""], ["", "", "", "", "", "", ""], ["7.2.1", "CANbus Resistance Test", "", "", "", "", ""], ["7.2.1.1", "J1.17 to J1.18", "> 10K", "-", "W", "", ""], ["", "", "", "", "", "", ""], ["7.3", "Sealing Test", "N/A", "-", "", "", ""], ["", "", "", "", "", "", ""], ["7.4", "Communication Test", "", "", "", "", ""], ["7.4.1", "Serial RS-232", "N/A", "-", "", "", ""], ["7.4.2", "CAN Bus", "N/A", "-", "", "", ""], ["", "", "", "", "", "", ""], ["7.5", "Performances Tests", "", "", "", "", ""], ["7.5.1", "Reverse Polarity Test", "", "", "", "", ""], ["7.5.1.1", "DC Input Current", "< 1", "-", "mA", "", ""], ["", "", "", "", "", "", ""], ["7.5.2", "Enable Test", "", "", "", "", ""], ["7.5.2.1", "Fan Speed at Opened Enable ", "5000", "+/-200.0", "rpm", "", ""], ["7.5.2.2", "Fan Speed at Opened Enable ", "0", "+/-200.0", "rpm", "", ""], ["7.5.2.3", "Fan Speed at Closed Enable ", "5000", "+/-200.0", "rpm", "", ""], ["7.5.2.4", "Motor Rotation Direction", "Counter-clockwise (Inlet)", "-", "", "", ""], ["", "", "", "", "", "", ""], ["7.5.3", "Stop Time Test ", "", "", "", "", ""], ["7.5.3.1", "Motor Stop time", "< 50", "-", "sec", "", ""], ["", "", "", "", "", "", ""], ["7.5.4", "Speed Command Test", "", "", "", "", ""], ["7.5.4.1", "Fan Speed", "6000", "+/-200.0", "rpm", "", ""], ["7.5.4.2", "Fan Speed", "11500", "+/-200.0", "rpm", "", ""], ["7.5.4.3", "Fan Speed", "15100", "+/-200.0", "rpm", "", ""], ["", "", "", "", "", "", ""], ["7.5.5", "Temperature Sensor Calibration Test", "", "", "", "", ""], ["7.5.5.1", "Sensor Reading Analog Offset", "0", "+/-0.100", ".", "", ""], ["", "", "", "", "", "", ""], ["7.5.6", "Temperature Control Algorithm Test", "", "", "", "", ""], ["7.5.6.1", "Tair <   68 ± 2 oC", "6000", "+/-200.0", "rpm", "", ""], ["7.5.6.2", "Measured Temp.", "", "", "C", "", ""], ["7.5.6.3", "Tair >= 68 ± 2 oC", "11500", "+/-200.0", "rpm", "", ""], ["7.5.6.4", "Transition Temp.", "", "", "C", "", ""], ["7.5.6.5", "Tair >= 88 ± 2 oC", "15100", "+/-400.0", "rpm", "", ""], ["7.5.6.6", "Transition Temp.", "", "", "C", "", ""], ["7.5.6.7", "Tair <= 80 ± 2 oC", "11500", "+/-200.0", "rpm", "", ""], ["7.5.6.8", "Transition Temp.", "", "", "C", "", ""], ["7.5.6.9", "Tair <= 60 ± 2 oC", "6000", "+/-200.0", "rpm", "", ""], ["7.5.6.10", "Transition Temp.", "", "", "C", "", ""], ["", "", "", "", "", "", ""], ["7.5.7", "Burn-in Test", "", "", "", "", ""], ["7.5.7.1", "DC Input Current", "50", "+/-5.000", "A", "", ""], ["7.5.7.2", "Fan Speed", "15100", "+/-200.0", "rpm", "", ""], ["7.5.7.3", "Ambient Temperature", "25", "+/-13.00", "C", "", ""], ["7.5.7.4", "After 10 min of operation", "", "-", "C", "", ""], ["7.5.7.5", "After 20 min of operation", "", "-", "C", "", ""], ["7.5.7.6", "After 30 min of operation", "", "-", "C", "", ""], ["", "", "", "", "", "", ""], ["8", "Auxiliary", "", "", "", "", ""], ["8.1", "Auxiliary Cooling Fan ON", "60", "+/-2.00", "C", "", ""], ["8.2", "Fan status", "ON", "-", "-", "", ""], ["8.3", "Auxiliary Cooling Fan OFF", "55", "+/-2.00", "C", "", ""], ["8.4", "Fan status", "OFF", "-", "-", "", ""], ["", "", "", "", "", "", ""], ["9", "Motor Temp. Test", "", "", "", "", ""], ["9.1", "60 Degree", "60", "+/-3.00", "C", "", ""], ["9.2", "90 Degree", "90", "+/-3.00", "C", "", ""], ["9.3", "120 Degree", "120", "+/-3.00", "C", "", ""]] ("data")
          }
        }
        "UUT" <- w1858
        "UUT" <- w1830
        n680 = for {
          tunnel: w1859 -> [w1894] mode=indexing
          tunnel: w1857 -> [w1892]
          tunnel: [w1891] -> w1853
          tunnel: w1859 -> [w1890]
          i -> [w1893]
          n681 = for {
            tunnel: w1894 -> [_] mode=indexing
            tunnel: w1893 -> [w1900]
            tunnel: w1892 -> [w1897]
            tunnel: [w1896] -> w1891
            tunnel: w1890 -> [w1895]
            i -> [w1901]
            n682 = Bundle By Name(cluster=T20 {"Row"=0, "Column"=0} ("Active Cell:Active Cell"), "Row"=w1900, "Column"=w1901) -> (w1899:T20)
            n683 = control-ref of="ATR"() -> (w1898:refnum<vi>)
            n684 = property class="Tbl (strict)"(reference=w1898, error in=w1897, "Active Cell"=w1899, "Cell BG Color"=u32 16777226, "Value"=w1895) -> (error out=w1896:errorcluster)  [unwired: 1 out]
          }
        }
        n685 = call "COM EvolutionBoard.vi"("error in (no error)"=w1853, "VISA resource name 2"=refnum<visa-resource-name> "COM1" ("VISA resource name")) -> ("error out"=w1849:errorcluster, "VISA resource name out"=w1848:refnum<visa-resource-name>)  [unwired: 8 in]
        n686 = call "TesterOption (SubVI).vi"("2 Options"=FALSE, "error in (no error)"=w1849, "On/Off"=FALSE, "Tester Option"=T11."Venable", "VISA Refnum in"=w1848) -> ("error out"=w1829:errorcluster, "VISA Refnum out"=→"VISA Tester":refnum<visa-resource-name>)  [unwired: 5 in]
        n687 = case shown="95" w1830 {
          tunnel: ["AHU Software Version" ("key") "EBAY Software Version" ("key")] -> w1839
          tunnel: ["AHU Serial Number" ("key") "EBAY Serial Number" ("key")] -> w1840
          frame 47, 63, Default {
          }
          frame 95 {
          }
        }
        n688 = call <vilib>:"Open Config Data.vi"("create file if necessary (T)"=FALSE, "configuration file path"=w1833) -> ("error out"=w1834:errorcluster, "refnum"=w1835:T25)  [unwired: 1 in, 7 out]
        n689 = call-poly <vilib>:"Read Key.vi"("section"=w1837, "error in (no error)"=w1834, "key"=w1839, "refnum"=w1835) -> ("error out"=w1841:errorcluster, "value"=→"UUT SoftwareVer":string, "refnum out"=w1838:T25)  [unwired: 2 in, 3 out]
        n690 = call-poly <vilib>:"Read Key.vi"("section"=w1837, "error in (no error)"=w1841, "key"=w1840, "refnum"=w1838) -> ("error out"=w1828:errorcluster, "value"=w1826:string, "refnum out"=w1827:T25)  [unwired: 2 in, 3 out]
        n691 = call <vilib>:"Close Config Data.vi"("error in (no error)"=w1828, "refnum"=w1827) -> ()  [unwired: 8 in, 2 out]
        n692 = Decimal String To Number(string=w1826) -> (number=w1831:i32)  [unwired: 2 in, 1 out]
        n693 = Increment(x=w1831) -> (x+1=→"Next SN":i32)
      }
      frame "Stop" {
        n694 = flat-sequence {
          tunnel: w1936 -> [w1974]
          tunnel: [w1973] -> w1929
          frame #0 {
            n695 = control-ref of="Pannel User Message"() -> (w1976:refnum<vi>)
            n696 = property class="Str"(reference=w1976, error in=w1974, "Value"="Program Stopped...\r\nPlease turn OFF All Power sinks") -> (error out=w1973:errorcluster)  [unwired: 1 out]
          }
        }
        n697 = control-ref of="VISA Tester"() -> (w1937:refnum<vi>)
        n698 = property class="VISAName"(reference=w1937, error in=w1929) -> ("Value"=w1935:refnum<visa-resource-name>)  [unwired: 2 out]
        n699 = disable-structure shown="Enabled" {
          disable-tunnel: w1929 -> [w1961 w1962]
          disable-tunnel: w1928 -> [w1959 _]
          disable-tunnel: [w1958 w1962] -> w1915
          frame Disabled {
            n700 = call "Clear CAN Buffer.vi"("error in (no error)"=w1961, "Cluster in"=w1959) -> ("error out"=w1960:errorcluster)  [unwired: 8 in, 1 out]
            n701 = call "Close CAN Device.vi"("error in (no error)"=w1960, "Cluster in"=w1959) -> ("error out"=w1958:errorcluster)  [unwired: 8 in, 1 out]
          }
          frame Enabled {
          }
        }
        n702 = VISA Close(VISA resource name=w1944, error in (no error)=w1929) -> (error out=w1938:errorcluster)
        n703 = property on="Stop Button" class="Bool (strict)"() -> ("Value"=w1907:bool)  [unwired: 2 in, 2 out]
        n704 = call "TesterOption (SubVI).vi"("2 Options"=FALSE, "On/Off"=FALSE, "Tester Option"=T11."Power", "VISA Refnum in"=w1935) -> ("error out"=w1924:errorcluster, "VISA Refnum out"=w1934:refnum<visa-resource-name>)  [unwired: 6 in]
        n705 = property on="ClosePanel" class="Bool (strict)"() -> ("Value"=w1908:bool)  [unwired: 2 in, 2 out]
        n706 = VISA Close(VISA resource name=w1934, error in (no error)=w1924) -> (error out=w1921:errorcluster)
        n707 = Or(x=w1908, y=w1907) -> (x .or. y?=w1906:bool)
        n708 = Flush Queue(queue=w1939, error in (no error)=w1938) -> (queue out=w1941:refnum<queue>, error out=w1940:errorcluster)  [unwired: 1 out]
        n709 = Flush Queue(queue=w1946, error in (no error)=w1938) -> (queue out=w1945:refnum<queue>, error out=w1947:errorcluster)  [unwired: 1 out]
        n710 = case shown="False" w1906 {
          tunnel: w1947 -> [w1949 w1957]
          tunnel: w1945 -> [w1951 w1953]
          tunnel: w1941 -> [w1950 w1952]
          tunnel: w1940 -> [w1948 w1956]
          tunnel: [w1949 w1955] -> w1923
          tunnel: [w1948 w1954] -> w1922
          tunnel: [w1951 w1953] -> w1905
          tunnel: [w1950 w1952] -> w1904
          frame False {
          }
          frame True {
            n711 = Release Queue(queue=w1952, error in (no error)=w1956) -> (error out=w1954:errorcluster)  [unwired: 1 in, 2 out]
            n712 = Release Queue(queue=w1953, error in (no error)=w1957) -> (error out=w1955:errorcluster)  [unwired: 1 in, 2 out]
          }
        }
        n713 = Merge Errors(w1923, w1922, w1921, w1915) -> (w1920:errorcluster)
        n714 = property on="Refresh Button" class="Bool (strict)"() -> ("Value"=w1909:bool)  [unwired: 2 in, 2 out]
        n715 = call <vilib>:"Clear Errors.vi"("error in (no error)"=w1920) -> ("error out"=w1919:errorcluster)  [unwired: 5 in, 1 out]
        n716 = property on="Stop Button" class="Bool (strict)"() -> ("Value"=w1913:bool)  [unwired: 2 in, 2 out]
        n717 = property on="ClosePanel" class="Bool (strict)"(error in=w1919) -> (error out=w1917:errorcluster, "Value"=w1918:bool)  [unwired: 1 in, 1 out]
        n718 = Not(x=w1909) -> (.not. x?=w1910:bool)
        n719 = Select(t=T10."Initialize", s=w1909, f=T10."Stop") -> (s? t:f=w1925:T10)
        n720 = Not(x=w1913) -> (.not. x?=w1912:bool)
        n721 = Compound Arithmetic op=AND(w1918, w1912, w1910) -> (w1914:bool)
        n722 = case shown="False" w1914 {
          tunnel: w1917 -> [w1965 w1969]
          tunnel: [w1965 w1969] -> w1916
          tunnel: [w1964 w1968] -> w1911
          tunnel: w1909 -> [w1963 _]
          frame False {
            n723 = case shown="False" w1963 {
              tunnel: [TRUE FALSE] -> w1964
              frame False {
              }
              frame True {
              }
            }
          }
          frame True {
            n724 = flat-sequence {
              tunnel: [TRUE] -> w1968
              frame #0 {
              }
              frame #1 {
                n725 = control-ref of="This VI"() -> (w1972:refnum<vi>)
                n726 = property class="VI"(reference=w1972, "FP.State"=T21."Closed" ("Front Panel Window:State")) -> ()  [unwired: 1 in, 2 out]
              }
            }
          }
        }
      }
      frame "MainProgram" {
        n727 = event shown="[8] \"Help Button\": Value Change" {
          selector: w1982 -> [_ _ _ _ _ _ _ _ _ _ _ _ _]
          dyn-events: _ -> [_ _ _ _ _ _ _ _ _ _ _ _ _]
          timeout: 120 -> [_ _ _ _ _ _ _ _ _ _ _ _ _]
          tunnel: [T10."MainProgram" T10."MainProgram" T10."MainProgram" T10."MainProgram" T10."MainProgram" T10."Stop" T10."MainProgram" w2567 T10."MainProgram" T10."MainProgram" T10."MainProgram" T10."Stop" T10."MainProgram"] -> w1995
          tunnel: [w1997 w2090 w2155 w2162 w2171 w2189 w2214 w2626 w2692 w2705 w2715 w2796 w2802] -> w1989
          tunnel: w1993 -> [w2010 w2090 w2154 w2164 w2171 w2189 w2221 w2626 w2693 w2704 w2711 w2796 w2807]
          tunnel: [w2018 w2084 w2156 w2163 w2172 w2187 w2210 w2575 w2690 w2702 w2716 w2794 w2800] -> w1990
          tunnel: w1991 -> [w2018 w2084 w2156 w2163 w2172 w2187 w2210 w2575 w2690 w2702 _ w2794 w2800]
          tunnel: w1988 -> [w2012 w2096 w2150 w2159 w2168 w2186 w2219 w2606 w2689 w2701 w2719 w2793 w2805]
          tunnel: w1987 -> [w2007 w2095 w2151 w2160 w2169 w2185 w2192 w2605 w2688 w2700 w2718 w2792 w2798]
          tunnel: [w2009 w2095 w2151 w2160 w2169 w2185 w2192 w2605 w2688 w2700 w2718 w2792 w2798] -> w1986
          tunnel: [w2011 w2096 w2150 w2159 w2168 w2186 w2219 w2606 w2689 w2701 w2719 w2793 w2805] -> w1985
          tunnel: w1984 -> [w2005 w2094 w2149 w2158 w2167 w2184 w2218 w2604 w2687 w2699 w2717 w2791 w2804]
          tunnel: [w2005 w2094 w2149 w2158 w2167 w2184 w2213 w2604 w2687 w2699 w2717 w2791 w2804] -> w1983
          tunnel: w1981 -> [_ _ _ _ _ _ _ w2573 _ _ _ _ _]
          tunnel: w1980 -> [w2006 w2093 w2148 w2157 w2166 w2182 w2208 w2579 w2686 w2698 w2713 w2790 w2803]
          tunnel: [w2006 w2093 w2148 w2157 w2166 w2182 w2208 w2578 w2686 w2698 w2713 w2790 w2803] -> w1979
          tunnel: w1978 -> [_ w2091 _ _ _ _ _ w2577 _ _ _ _ _]
          tunnel: w1977 -> [_ w2083 _ _ _ _ _ _ _ _ _ _ _]
          event Timeout {
            n728 = event-data() -> ()  [unwired: 1 in, 3 out]
            n729 = property class="Clust (strict)"(reference=w2007, error in=w2010) -> (reference out=w2009:refnum<vi>, error out=w2008:errorcluster, "Value"=w2015:T7)
            n730 = Unbundle By Name(w2015) -> ("DevType"=w2016:T2, "CanIndex"=w2014:T1)
            n731 = property on="ClosePanel" class="Bool (strict)"("Value"=FALSE ("ClosePanel")) -> ()  [unwired: 2 in, 2 out]
            n732 = call "VCI_Receive.vi"("CANIndex"=w2014, "DevIndex"=u32 0, "DevType"=w2016) -> ("Recieve"=w2013:T26[])  [unwired: 3 in, 5 out]
            n733 = Empty Array?(array=w2013) -> (empty?=w2000:bool)
            n734 = case shown="False" w2000 {
              tunnel: w2014 -> [w2032 _]
              tunnel: w2009 -> [w2030 _]
              tunnel: w2012 -> [w2029 w2065]
              tunnel: w2008 -> [w2028 w2064]
              tunnel: w2013 -> [w2033 _]
              tunnel: [w2023 w2064] -> w1997
              tunnel: [w2022 w2065] -> w2011
              tunnel: [TRUE FALSE] -> w1996
              frame False {
                n735 = call "Demo_MakeDispBuff.vi"("Channel"=w2032, "Type"=enum16{"接收", "发送"}."接收", "OBJs"=w2033) -> ("Buffer"=w2031:T27)
                n736 = for {
                  N: 3 -> [_]
                  tunnel: w2031 -> [w2047]
                  tunnel: w2030 -> [w2046]
                  tunnel: w2029 -> [w2037]
                  tunnel: w2028 -> [w2036]
                  tunnel: [w2039] -> w2026 mode=indexing
                  tunnel: [w2037] -> w2025
                  tunnel: [w2036] -> w2024
                  i -> [w2035]
                  n737 = property class="Clust (strict)"(reference=w2046) -> ("Value"=w2044:T7)  [unwired: 1 in, 2 out]
                  n738 = Index Array(array=w2047, index=w2035) -> (element=w2040:T28)
                  n739 = Unbundle By Name(w2040) -> ("Channel"=w2042:T1, "VCI_CAN_OBJ"=w2045:T26)  [unwired: 2 out]
                  n740 = Unbundle By Name(w2044) -> ("CanIndex"=w2043:T1)
                  n741 = Equal?(x=w2043, y=w2042) -> (x = y?=w2041:bool)
                  n742 = case shown="True" w2041 {
                    tunnel: w2045 -> [_ w2058]
                    tunnel: [w2048 w2054] -> w2039
                    tunnel: T22 {"ID"=0, "MSGTYPE"=0, "LEN"=0, "aDATA"=[]} ("Msg") -> [w2048 w2053]
                    frame False {
                    }
                    frame True {
                      n743 = Unbundle By Name(w2058) -> ("ID"=w2052:u32, "DataLen"=w2057:u8, "Data"=w2055:u8[])
                      n744 = Bundle By Name(cluster=w2053, "ID"=w2052, "MSGTYPE"=u8 0, "LEN"=w2057, "aDATA"=w2055) -> (w2054:T22)
                      n745 = Unbundle By Name(w2054) -> ("ID"=w2050:u32)
                      n746 = Split Number(x=w2050) -> (lo(x)=w2051:u16)  [unwired: 1 out]
                      n747 = Split Number(x=w2051) -> (lo(x)=w2049:u8)  [unwired: 1 out]
                      n748 = case shown="63" w2049 {
                        tunnel: ["EBAY 5F" "" "AHU 3F" "AHU 2F"] -> _
                        frame 95 {
                        }
                        frame Default {
                        }
                        frame 63 {
                        }
                        frame 47 {
                        }
                      }
                    }
                  }
                }
                n749 = Enqueue Element(queue=w2025, element=w2026, error in (no error)=w2024) -> (queue out=w2022:refnum<queue>, error out=w2023:errorcluster)  [unwired: 2 out]
              }
              frame True {
              }
            }
            n750 = control-ref of="ATR"() -> (w1999:refnum<vi>)
            n751 = property on="CAN Status" class="Bool (strict)"("Value"=w1996) -> ()  [unwired: 2 in, 2 out]
            n752 = call "PassFailUUT (SubVI).vi"("error in (no error)"=w1997, "Table in"=w1999) -> ("PassFaileUUTresult"=w1998:bool)  [unwired: 7 in, 2 out]
            n753 = property on="Test Failed" class="Bool (strict)"("Value"=w1998) -> ()  [unwired: 2 in, 2 out]
            n754 = property on="Automation" class="Bool (strict)"() -> ("Value"=w2002:bool)  [unwired: 2 in, 2 out]
            n755 = property on="Start" class="Bool (strict)"() -> ("Value"=w2004:bool)  [unwired: 2 in, 2 out]
            n756 = Or(x=w2002, y=w2004) -> (x .or. y?=w2003:bool)
            n757 = case shown="False" w2003 {
              frame False {
                n758 = property on="Pannel User Message" class="Str"("Value"="You can press start to execute(s) test(s).") -> ()  [unwired: 2 in, 2 out]
              }
              frame True {
              }
            }
          }
          event "SetSN": Value Change {
            n759 = event-data() -> ()  [unwired: 1 in, 6 out]
            n760 = property on="UUT" class="DigNum (strict)"() -> ("Value"=w2074:u8)  [unwired: 2 in, 2 out]
            n761 = Equal?(x=w2074, y=u8 95) -> (x = y?=w2072:bool)
            n762 = control-ref of="ATR"() -> (w2075:refnum<vi>)
            n763 = Select(t=u8 50 ("y"), s=w2072, f=u8 36 ("y")) -> (s? t:f=w2067:u8)
            n764 = property on="Current SN" class="DigNum (strict)"(error in=w2090) -> (error out=w2069:errorcluster, "Value"=w2089:i32)  [unwired: 1 in, 1 out]
            n765 = call "PassFailUUT (SubVI).vi"("error in (no error)"=w2069, "Table in"=w2075) -> ("Total Pass"=w2068:u8)  [unwired: 7 in, 2 out]
            n766 = Equal To 0?(x=w2089) -> (x = 0?=w2086:bool)
            n767 = Equal?(x=w2089, y=-1) -> (x = y?=w2087:bool)
            n768 = Equal?(x=w2068, y=w2067) -> (x = y?=w2066:bool)
            n769 = Or(x=w2087, y=w2086) -> (x .or. y?=w2085:bool)
            n770 = property on="CAN Status" class="Bool (strict)"() -> ("Value"=w2076:bool)  [unwired: 2 in, 2 out]
            n771 = property on="Status" class="Bool (strict)"() -> ("Value"=w2081:bool)  [unwired: 2 in, 2 out]
            n772 = And(x=w2081, y=w2076) -> (x .and. y?=w2077:bool)
            n773 = case shown="True" w2077 {
              tunnel: w2091 -> [_ w2110]
              tunnel: w2085 -> [_ w2099]
              tunnel: w2084 -> [_ w2109]
              tunnel: w2083 -> [_ w2108]
              tunnel: [errorcluster {"status"=FALSE, "code"=0, "source"=""} ("error out") w2107] -> w2080
              tunnel: [w2097 w2106] -> w2082
              tunnel: w2066 -> [_ w2100]
              frame False {
                w2097 = FALSE ("Value")
                n774 = property on="SetSN" class="Bool (strict)"("Value"=w2097) -> ()  [unwired: 2 in, 2 out]
                n775 = call "Display Message to User10"() -> ()  [unwired: 10 in, 2 out]
              }
              frame True {
                n776 = property on="Test Failed" class="Bool (strict)"() -> ("Value"=w2104:bool)  [unwired: 2 in, 2 out]
                n777 = property on="Automation" class="Bool (strict)"() -> ("Value"=w2106:bool)  [unwired: 2 in, 2 out]
                n778 = Not(x=w2104) -> (.not. x?=w2105:bool)
                n779 = Select(t=w2105, s=w2106, f=w2108) -> (s? t:f=w2102:bool)
                n780 = Or(x=w2100, y=w2102) -> (x .or. y?=w2101:bool)
                n781 = And(x=w2099, y=w2101) -> (x .and. y?=w2103:bool)
                n782 = case shown="False" w2103 {
                  tunnel: w2110 -> [_ w2140]
                  tunnel: w2109 -> [_ w2133]
                  tunnel: [w2112 w2125] -> w2107
                  tunnel: w2099 -> [w2111 _]
                  frame False {
                    n783 = case shown="False" w2111 {
                      tunnel: [w2114 w2115] -> w2112
                      frame False {
                        n784 = call "Display Message to User9"() -> ("error out"=w2114:errorcluster)  [unwired: 10 in, 1 out]
                      }
                      frame True {
                        n785 = call "Display Message to User3"() -> ("error out"=w2115:errorcluster)  [unwired: 10 in, 1 out]
                      }
                    }
                    n786 = property on="Automation" class="Bool (strict)"(error in=w2112, "Value"=FALSE ("Automation")) -> ()  [unwired: 1 in, 2 out]
                  }
                  frame True {
                    w2132 = FALSE ("SetSN")
                    n787 = property on="Next SN" class="DigNum (strict)"() -> ("Value"=w2116:i32)  [unwired: 2 in, 2 out]
                    n788 = property on="VISA Tester" class="VISAName"() -> ("Value"=w2123:refnum<visa-resource-name>)  [unwired: 2 in, 2 out]
                    n789 = call "TesterOption (SubVI).vi"("2 Options"=FALSE, "On/Off"=FALSE, "Tester Option"=T11."Venable", "VISA Refnum in"=w2123) -> ("error out"=w2118:errorcluster)  [unwired: 6 in, 1 out]
                    n790 = call <vilib>:"Clear Errors.vi"("error in (no error)"=w2118) -> ("error out"=w2119:errorcluster)  [unwired: 5 in, 1 out]
                    n791 = Number To Decimal String(number=w2116) -> (decimal integer string=w2117:string)  [unwired: 1 in]
                    "UUT SN Report" <- w2117
                    n792 = Search and Replace String(input string="EP=1\r\nSN=0\r\n" ("write buffer"), search string="0", replace string=w2117) -> (result string=w2135:string)  [unwired: 5 in, 3 out]
                    n793 = call "SerialMarvinSendGet.vi"("error in (no error)"=w2119, "Clear Log"=FALSE, "write buffer"=w2135, "VISA resource name"=w2133) -> ("error out"=w2124:errorcluster)  [unwired: 6 in, 1 out]
                    n794 = property on="UUT" class="DigNum (strict)"(error in=w2124) -> ("Value"=w2141:u8)  [unwired: 1 in, 2 out]
                    n795 = case shown="47, 63, Default" w2141 {
                      tunnel: ["AHU Serial Number" ("key") "EBAY Serial Number" ("key")] -> w2144
                      frame 47, 63, Default {
                      }
                      frame 95 {
                      }
                    }
                    n796 = call <vilib>:"Open Config Data.vi"("create file if necessary (T)"=FALSE, "configuration file path"=w2140) -> ("error out"=w2138:errorcluster, "refnum"=w2139:T25)  [unwired: 1 in, 7 out]
                    n797 = call-poly <vilib>:"Write Key.vi"("section"="Marvin", "error in (no error)"=w2138, "value"=w2117, "key"=w2144, "refnum"=w2139) -> ("error out"=w2128:errorcluster, "refnum out"=w2127:T25)  [unwired: 4 in, 1 out]
                    n798 = call <vilib>:"Close Config Data.vi"("error in (no error)"=w2128, "refnum"=w2127) -> ("error out"=w2126:errorcluster)  [unwired: 8 in, 1 out]
                    n799 = property on="Current SN" class="DigNum (strict)"("Value"=w2116) -> ()  [unwired: 2 in, 2 out]
                    n800 = property on="SetSN" class="Bool (strict)"(error in=w2126, "Value"=w2132) -> (error out=w2131:errorcluster)  [unwired: 1 in, 1 out]
                    n801 = property on="Automation" class="Bool (strict)"(error in=w2131, "Value"=w2132) -> (error out=w2130:errorcluster)  [unwired: 1 in, 1 out]
                    n802 = Increment(x=w2116) -> (x+1=w2129:i32)
                    n803 = property on="Next SN" class="DigNum (strict)"(error in=w2130, "Value"=w2129) -> (error out=w2125:errorcluster)  [unwired: 1 in, 1 out]
                  }
                }
              }
            }
            n804 = property on="SetSN" class="Bool (strict)"(error in=w2080, "Value"=FALSE ("SetSN")) -> (error out=w2079:errorcluster)  [unwired: 1 in, 1 out]
            n805 = case shown="True" w2082 {
              tunnel: w2079 -> [_ _]
              frame False {
              }
              frame True {
                w2147 = TRUE ("Value (Signaling)")
                n806 = property on="Report" class="Bool (strict)"("Val(Sgnl)"=w2147, "Value"=w2147) -> ()  [unwired: 2 in, 2 out]
              }
            }
          }
          event "ATR": Mouse Enter {
            n807 = event-data() -> ()  [unwired: 1 in, 4 out]
            n808 = call-poly <vilib>:"Set Cursor.vi"("error in (no error)"=w2154, "icon"=u16 1) -> ("error out"=w2155:errorcluster)  [unwired: 8 in, 1 out]
          }
          event "ATR": Mouse Leave {
            n809 = event-data() -> ()  [unwired: 1 in, 4 out]
            n810 = call-poly <vilib>:"Set Cursor.vi"("error in (no error)"=w2164, "icon"=u16 0) -> ("error out"=w2162:errorcluster)  [unwired: 8 in, 1 out]
          }
          event "ATR": Mouse Down? {
            n811 = event-data() -> ("Coords"=w2179:T29)  [unwired: 1 in, 4 out]
            n812 = invoke on="ATR" class="Tbl (strict)" method="Point To Row Column"("Point"=w2179) -> ("InBounds"=w2175:bool, "CellPosition"=w2174:T20)  [unwired: 5 in, 4 out]
            n813 = Greater Than 0?(x=w2174) -> (x > 0?=w2178:cluster{"Row":bool, "Column":bool})
            n814 = Cluster To Array(cluster=w2178) -> (array=w2177:bool[])
            n815 = Or Array Elements(Boolean array=w2177) -> (logical OR=w2176:bool)
            n816 = Or(x=w2175, y=w2176) -> (x .or. y?=w2173:bool)
            n817 = event-data("Discard?"=w2173) -> ()  [unwired: 1 in, 1 out]
          }
          event Panel Close? {
            n818 = event-data() -> ("VIRef"=w2183:refnum<vi>)  [unwired: 1 in, 3 out]
            n819 = Close Reference(reference=w2183) -> ()  [unwired: 1 in, 1 out]
            n820 = disable-structure shown="Disabled" {
              frame Disabled {
                n821 = property on="Stop Button" class="Bool (strict)"("Val(Sgnl)"=TRUE ("Stop Button"), "Value"=FALSE ("Stop Button")) -> ()  [unwired: 2 in, 2 out]
              }
              frame Enabled {
              }
            }
            n822 = event-data("Discard?"=TRUE) -> ()  [unwired: 1 in, 1 out]
            "ClosePanel" <- TRUE ("ClosePanel")
          }
          event "Start": Value Change {
            w2209 = T16 [] items=["Auxiliary", "Temp Sens Cal", "Com Test", "Enable Test", "Speed Command", "Stop Time", "Temp Control", "Burn in", "Visual Inspec", "Empty"]
            n823 = event-data() -> ()  [unwired: 1 in, 2 out]
            n824 = property on="VISA Tester" class="VISAName"() -> ("Value"=w2207:refnum<visa-resource-name>)  [unwired: 2 in, 2 out]
            n825 = property on="UUT" class="Str"(error in=w2221) -> (error out=w2203:errorcluster, "Value"=w2220:string)  [unwired: 1 in, 1 out]
            n826 = control-ref of="Pannel User Message"() -> (w2200:refnum<vi>)
            n827 = control-ref of="Motor Speed RPM"() -> (w2195:refnum<vi>)
            n828 = call "TesterOption (SubVI).vi"("2 Options"=FALSE, "error in (no error)"=w2203, "On/Off"=FALSE, "Tester Option"=T11."Venable", "VISA Refnum in"=w2207) -> ("error out"=w2202:errorcluster)  [unwired: 5 in, 1 out]
            n829 = control-ref of="Stop Burn-in"() -> (w2198:refnum<vi>)
            n830 = control-ref of="Stop Button"() -> (w2199:refnum<vi>)
            n831 = call "Write panel message (SubVI).vi"("Stop BurnIn"=w2198, 4:"rpm"=w2195, 5:"rpm"=FALSE ("rpm"), "PrintTime"=TRUE, "Stop"=w2199, "error in (no error)"=w2202, "Time to wait"=5.0, "Strin"="TESTER BIT TEST OPERATION IN PROCESS", "String in"=w2200) -> ("error out"=w2201:errorcluster)  [unwired: 2 in]
            n832 = while {
              tunnel: w2220 -> [w2249]
              tunnel: [w2248] -> w2216
              tunnel: [w2247] -> w2215
              shift-right: [w2244] -> _
              shift-left: enum16{"Stop", "Tests", "Bit test", "Start"}."Start" -> [w2246]
              tunnel: w2210 -> [w2245]
              tunnel: w2209 -> [w2243]
              tunnel: w2201 -> [w2228]
              tunnel: w2199 -> [w2237]
              tunnel: w2198 -> [w2236]
              tunnel: w2200 -> [w2235]
              tunnel: w2195 -> [w2234]
              tunnel: w2192 -> [w2227]
              stop <- w2242 stop-if-true
              n833 = property class="Clust (strict)"(reference=w2227, error in=w2228) -> ("Value"=w2230:T7)  [unwired: 2 out]
              n834 = Unbundle By Name(w2230) -> ("DevType"=w2232:T2, "CanIndex"=w2231:T1)
              n835 = property on="VISA Tester" class="VISAName"() -> ("Value"=w2240:refnum<visa-resource-name>)  [unwired: 2 in, 2 out]
              n836 = call "VCI_Receive.vi"("CANIndex"=w2231, "DevIndex"=u32 0, "DevType"=w2232) -> ("Recieve"=w2233:T26[])  [unwired: 3 in, 5 out]
              n837 = Empty Array?(array=w2233) -> (empty?=w2226:bool)
              n838 = Not(x=w2226) -> (.not. x?=w2225:bool)
              n839 = property on="CAN Status" class="Bool (strict)"("Value"=w2225) -> (error out=w2224:errorcluster)  [unwired: 2 in, 1 out]
              n840 = property on="CAN Status" class="Bool (strict)"(error in=w2224) -> (error out=w2223:errorcluster, "Value"=w2238:bool)  [unwired: 1 in, 1 out]
              n841 = property on="Status" class="Bool (strict)"(error in=w2223) -> (error out=w2239:errorcluster, "Value"=w2241:bool)  [unwired: 1 in, 1 out]
              n842 = case shown="\"Start\"" w2246 {
                tunnel: w2249 -> [_ w2264 w2374 _]
                tunnel: [w2254 w2263 w2409 w2515] -> w2248
                tunnel: [w2250 w2262 w2372 w2507] -> w2247
                tunnel: w2245 -> [_ _ w2390 w2520]
                tunnel: w2235 -> [_ _ _ w2519]
                tunnel: w2237 -> [_ _ _ w2518]
                tunnel: w2236 -> [_ _ _ w2517]
                tunnel: w2234 -> [_ _ _ w2516]
                tunnel: [w2253 w2261 w2377 w2511] -> w2244
                tunnel: w2243 -> [w2254 _ w2409 w2515]
                tunnel: [w2252 w2260 FALSE FALSE] -> w2242
                tunnel: w2241 -> [_ _ _ w2513]
                tunnel: w2240 -> [_ _ w2391 _]
                tunnel: w2239 -> [w2250 _ _ _]
                tunnel: w2238 -> [_ _ _ w2508]
                frame "Stop", Default {
                  n843 = property on="Start" class="Bool (strict)"(error in=w2250, "Value"=FALSE ("Start")) -> ()  [unwired: 1 in, 2 out]
                  n844 = flat-sequence {
                    tunnel: [enum16{"Stop", "Tests", "Bit test", "Start"}."Stop"] -> w2253
                    tunnel: w2250 -> [_]
                    tunnel: [TRUE] -> w2252
                    frame #0 {
                    }
                  }
                }
                frame "Tests" {
                  w2257 = FALSE ("Stop Burn-in")
                  w2259 = T19."Disabled and Grayed Out" ("Disabled")
                  n845 = case shown="\"AHU\", Default" w2264 {
                    tunnel: [w2279 w2328] -> w2263
                    tunnel: [w2278 w2327] -> w2262
                    tunnel: [w2267 w2315] -> w2258
                    frame "AHU", Default {
                      n846 = call "Load Program Process AHU.vi"() -> ("Speed Command Test"=w2272:bool, "Enable Test"=w2273:bool, "Burn-in Test"=w2270:bool, "Auxiliary"=w2268:bool, "Temperature Sensor Calibration Test"=w2275:bool, "Communication Test"=w2274:bool, "Stop Time Test"=w2271:bool, "Visual Inspection"=w2269:bool, "OK"=w2276:bool, "Automation"=w2267:bool, "error out"=w2278:errorcluster)  [unwired: 8 in, 9 out]
                      n847 = Or(x=w2276, y=w2267) -> (x .or. y?=w2277:bool)
                      n848 = case shown="True" w2277 {
                        tunnel: [w2280 w2290] -> w2279
                        tunnel: w2267 -> [_ w2289]
                        tunnel: w2275 -> [_ w2288]
                        tunnel: w2274 -> [_ w2287]
                        tunnel: w2273 -> [_ w2286]
                        tunnel: w2272 -> [_ w2285]
                        tunnel: w2271 -> [_ w2284]
                        tunnel: w2270 -> [_ w2283]
                        tunnel: w2269 -> [_ w2282]
                        tunnel: w2268 -> [_ w2281]
                        frame False {
                          w2280 = T16 [] items=["Auxiliary", "Temp Sens Cal", "Com Test", "Enable Test", "Speed Command", "Stop Time", "Temp Control", "Burn in", "Visual Inspec", "Empty"]
                        }
                        frame True {
                          n849 = case shown="False" w2289 {
                            tunnel: [w2313 w2314] -> w2290
                            tunnel: w2288 -> [w2295 _]
                            tunnel: w2287 -> [w2294 _]
                            tunnel: w2286 -> [w2296 _]
                            tunnel: w2285 -> [w2293 _]
                            tunnel: w2284 -> [w2292 _]
                            tunnel: w2283 -> [w2306 _]
                            tunnel: w2282 -> [w2291 _]
                            tunnel: w2281 -> [_ _]
                            frame False {
                              w2299 = T23."Empty" ("f")
                              n850 = Select(t=T23."Com Test" ("f"), s=w2294, f=w2299) -> (s? t:f=w2305:T23)
                              n851 = Select(t=T23."Temp Sens Cal" ("f"), s=w2295, f=w2299) -> (s? t:f=w2304:T23)
                              n852 = Select(t=T23."Stop Time" ("f"), s=w2292, f=w2299) -> (s? t:f=w2303:T23)
                              n853 = Select(t=T23."Enable Test" ("f"), s=w2296, f=w2299) -> (s? t:f=w2302:T23)
                              n854 = Select(t=T23."Speed Command" ("f"), s=w2293, f=w2299) -> (s? t:f=w2301:T23)
                              n855 = Select(t=T23."Burn in" ("f"), s=w2306, f=w2299) -> (s? t:f=w2300:T23)
                              n856 = Select(t=T23."Visual Inspec" ("f"), s=w2291, f=w2299) -> (s? t:f=w2297:T23)
                              n857 = Build Array(w2305, w2304, w2303, w2302, w2301, w2300, w2297) -> (w2313:T16)
                            }
                            frame True {
                              w2314 = T16 [enum."Com Test", enum."Temp Sens Cal", enum."Stop Time", enum."Enable Test", enum."Speed Command", enum."Burn in", enum."Visual Inspec"] items=["Auxiliary", "Temp Sens Cal", "Com Test", "Enable Test", "Speed Command", "Stop Time", "Temp Control", "Burn in", "Visual Inspec", "Empty"]
                            }
                          }
                        }
                      }
                    }
                    frame "EBAY" {
                      n858 = call "Load Program Process EBAY.vi"() -> ("Speed Command Test"=w2321:bool, "Enable Test"=w2322:bool, "Burn-in Test"=w2319:bool, "Temperature Control Algorithm Test"=w2318:bool, "Auxiliary"=w2316:bool, "Temperature Sensor Calibration Test"=w2324:bool, "Communication Test"=w2323:bool, "Stop Time Test"=w2320:bool, "Visual Inspection"=w2317:bool, "OK"=w2325:bool, "Automation"=w2315:bool, "error out"=w2327:errorcluster)  [unwired: 8 in, 8 out]
                      n859 = Or(x=w2325, y=w2315) -> (x .or. y?=w2326:bool)
                      n860 = case shown="True" w2326 {
                        tunnel: [w2329 w2340] -> w2328
                        tunnel: w2315 -> [_ w2339]
                        tunnel: w2324 -> [_ w2338]
                        tunnel: w2323 -> [_ w2337]
                        tunnel: w2322 -> [_ w2336]
                        tunnel: w2321 -> [_ w2335]
                        tunnel: w2320 -> [_ w2334]
                        tunnel: w2319 -> [_ w2333]
                        tunnel: w2318 -> [_ w2332]
                        tunnel: w2317 -> [_ w2331]
                        tunnel: w2316 -> [_ w2330]
                        frame False {
                          w2329 = T16 [] items=["Auxiliary", "Temp Sens Cal", "Com Test", "Enable Test", "Speed Command", "Stop Time", "Temp Control", "Burn in", "Visual Inspec", "Empty"]
                        }
                        frame True {
                          n861 = case shown="False" w2339 {
                            tunnel: [w2369 w2370] -> w2340
                            tunnel: w2338 -> [w2345 _]
                            tunnel: w2337 -> [w2344 _]
                            tunnel: w2336 -> [w2343 _]
                            tunnel: w2335 -> [w2342 _]
                            tunnel: w2334 -> [w2341 _]
                            tunnel: w2333 -> [w2347 _]
                            tunnel: w2332 -> [w2346 _]
                            tunnel: w2331 -> [w2360 _]
                            tunnel: w2330 -> [w2351 _]
                            frame False {
                              w2349 = T23."Empty" ("f")
                              n862 = Select(t=T23."Com Test" ("f"), s=w2344, f=w2349) -> (s? t:f=w2359:T23)
                              n863 = Select(t=T23."Temp Sens Cal" ("f"), s=w2345, f=w2349) -> (s? t:f=w2358:T23)
                              n864 = Select(t=T23."Stop Time" ("f"), s=w2341, f=w2349) -> (s? t:f=w2357:T23)
                              n865 = Select(t=T23."Enable Test" ("f"), s=w2343, f=w2349) -> (s? t:f=w2356:T23)
                              n866 = Select(t=T23."Speed Command" ("f"), s=w2342, f=w2349) -> (s? t:f=w2355:T23)
                              n867 = Select(t=T23."Temp Control" ("f"), s=w2346, f=w2349) -> (s? t:f=w2354:T23)
                              n868 = Select(t=T23."Burn in" ("f"), s=w2347, f=w2349) -> (s? t:f=w2353:T23)
                              n869 = Select(t=T23."Visual Inspec" ("f"), s=w2360, f=w2349) -> (s? t:f=w2352:T23)
                              n870 = Select(t=T23."Auxiliary" ("f"), s=w2351, f=w2349) -> (s? t:f=w2348:T23)
                              n871 = Build Array(w2359, w2358, w2357, w2356, w2355, w2354, w2353, w2348, w2352) -> (w2369:T16)
                            }
                            frame True {
                              w2370 = T16 [enum."Com Test", enum."Temp Sens Cal", enum."Stop Time", enum."Enable Test", enum."Speed Command", enum."Temp Control", enum."Burn in", enum."Auxiliary", enum."Visual Inspec"] items=["Auxiliary", "Temp Sens Cal", "Com Test", "Enable Test", "Speed Command", "Stop Time", "Temp Control", "Burn in", "Visual Inspec", "Empty"]
                            }
                          }
                        }
                      }
                    }
                  }
                  "Automation" <- w2258
                  n872 = flat-sequence {
                    tunnel: [enum16{"Stop", "Tests", "Bit test", "Start"}."Tests"] -> w2261
                    tunnel: [TRUE] -> w2260
                    frame #0 {
                    }
                  }
                  n873 = property on="Stop Button" class="Bool (strict)"("Value"=w2257) -> ()  [unwired: 2 in, 2 out]
                  n874 = property on="Stop Burn-in" class="Bool (strict)"("Value"=w2257) -> ()  [unwired: 2 in, 2 out]
                  n875 = property on="Start" class="Bool (strict)"("DisabledEnum"=w2259) -> ()  [unwired: 2 in, 2 out]
                  n876 = property on="Report" class="Bool (strict)"("DisabledEnum"=w2259) -> ()  [unwired: 2 in, 2 out]
                }
                frame "Bit test" {
                  # "Stop"
                  n877 = call "SerialMarvinSendGet.vi"("write buffer"="TA[1]\r\n", "VISA resource name"=w2390) -> ("error out"=w2403:errorcluster, "read buffer"=w2406:string)  [unwired: 8 in]
                  n878 = Fract/Exp String To Number(string=w2406) -> (number=w2405:dbl)  [unwired: 3 in, 1 out]
                  n879 = Less Or Equal?(x=w2405, y=100.0) -> (x <= y?=w2388:bool)
                  n880 = call "TesterOption (SubVI).vi"("On/Off 2"=FALSE, "Tester Option 2"=T11."Venable", "2 Options"=TRUE, "error in (no error)"=w2403, "On/Off"=TRUE, "Tester Option"=T11."25C", "VISA Refnum in"=w2391) -> ("error out"=w2393:errorcluster)  [unwired: 3 in, 1 out]
                  n881 = call "Time Delay5"("error in (no error)"=w2393) -> ("error out"=w2392:errorcluster)  [unwired: 10 in]
                  n882 = call "SerialMarvinSendGet.vi"("error in (no error)"=w2392, "write buffer"="TA[2]\r\n", "VISA resource name"=w2390) -> ("error out"=w2389:errorcluster, "read buffer"=w2395:string)  [unwired: 7 in]
                  n883 = case shown="\"EBAY\"" w2374 {
                    tunnel: w2391 -> [w2439 _ w2467]
                    tunnel: w2390 -> [_ _ w2470]
                    tunnel: w2389 -> [w2440 w2458 w2469]
                    tunnel: [w2433 w2458 w2465] -> w2376
                    tunnel: [w2430 "" w2460] -> w2383
                    tunnel: [w2429 bool[] [] w2459] -> w2381
                    frame "AHU" {
                      n884 = call "TesterOption (SubVI).vi"("On/Off 2"=FALSE, "Tester Option 2"=T11."Venable", "2 Options"=TRUE, "error in (no error)"=w2440, "On/Off"=TRUE, "Tester Option"=T11."K17", "VISA Refnum in"=w2439) -> ("error out"=w2442:errorcluster)  [unwired: 3 in, 1 out]
                      n885 = call "Time Delay7"("error in (no error)"=w2442) -> ("error out"=w2441:errorcluster)  [unwired: 10 in]
                      n886 = call "GetADCTester (SubVI).vi"("error in (no error)"=w2441, "GetADCTester"=T13."Current", "TimeToGet"=5, "VISA Refnum in"=w2439) -> ("error out"=w2433:errorcluster, "ADCValOutput Single"=w2435:dbl)  [unwired: 5 in, 1 out]
                      n887 = Less Or Equal?(x=w2435, y=50.0) -> (x <= y?=w2434:bool)
                      n888 = Build Array(w2434) -> (w2429:bool[])
                      n889 = for {
                        tunnel: w2429 -> [w2455] mode=indexing
                        tunnel: string[] ["CURRENT OPERATION FAILED!"] -> [w2451] mode=indexing
                        shift-right: [w2453] -> w2430
                        shift-left: "" -> [w2452]
                        n890 = Concatenate Strings(w2451, "  TEST FAILED!" ("string"), "\r\n") -> (w2448:string)
                        n891 = Select(t=w2448, s=w2455, f=w2452) -> (s? t:f=w2454:string)
                        n892 = Concatenate Strings(w2452, w2454) -> (w2453:string)
                      }
                    }
                    frame Default {
                    }
                    frame "EBAY" {
                      w2468 = T30 [enum."Fan", enum."Current"] items=["Term1", "Term2", "Current", "Fan", "TempCPU"]
                      n893 = call "TesterOption (SubVI).vi"("On/Off 2"=FALSE, "Tester Option 2"=T11."Venable", "2 Options"=TRUE, "error in (no error)"=w2469, "On/Off"=TRUE, "Tester Option"=T11."K17", "VISA Refnum in"=w2467) -> ("error out"=w2472:errorcluster)  [unwired: 3 in, 1 out]
                      n894 = call "Time Delay6"("error in (no error)"=w2472) -> ("error out"=w2471:errorcluster)  [unwired: 10 in]
                      n895 = call "SerialMarvinSendGet.vi"("error in (no error)"=w2471, "write buffer"="TA[3]\r\n", "VISA resource name"=w2470) -> ("error out"=w2466:errorcluster, "read buffer"=w2474:string)  [unwired: 7 in]
                      n896 = Fract/Exp String To Number(string=w2474) -> (number=w2475:dbl)  [unwired: 3 in, 1 out]
                      n897 = for {
                        tunnel: w2468 -> [w2499] mode=indexing
                        tunnel: w2467 -> [w2498]
                        tunnel: w2466 -> [w2496]
                        tunnel: [w2495] -> w2465
                        tunnel: [w2492] -> w2463 mode=indexing
                        i -> [w2493]
                        n898 = call "GetADCTester (SubVI).vi"("error in (no error)"=w2496, "GetADCTester"=w2499, "TimeToGet"=0, "VISA Refnum in"=w2498) -> ("error out"=w2495:errorcluster, "ADCValOutput Single"=w2494:dbl)  [unwired: 5 in, 1 out]
                        n899 = case shown="1" w2493 {
                          tunnel: w2494 -> [w2502 w2505 _]
                          tunnel: [w2500 w2503 FALSE] -> w2492
                          frame 1 {
                            n900 = Less Or Equal?(x=w2502, y=50.0) -> (x <= y?=w2500:bool)
                          }
                          frame 0 {
                            n901 = Greater Or Equal?(x=w2505, y=2200.0) -> (x >= y?=w2503:bool)
                          }
                          frame Default {
                          }
                        }
                      }
                      n902 = Less Or Equal?(x=w2475, y=100.0) -> (x <= y?=w2464:bool)
                      n903 = Build Array (concatenate)(w2464, w2463) -> (w2459:bool[])
                      n904 = for {
                        tunnel: w2459 -> [w2482] mode=indexing
                        tunnel: string[] ["TA[3] OPERATION FAILED!", "EBAY FAN OPERATION FAILED!", "CURRENT OPERATION FAILED!"] -> [w2485] mode=indexing
                        shift-right: [w2487] -> w2460
                        shift-left: "" -> [w2486]
                        n905 = Concatenate Strings(w2485, "\r\n") -> (w2483:string)
                        n906 = case shown="False" w2482 {
                          tunnel: [w2490 w2491] -> w2487
                          tunnel: w2486 -> [w2489 w2491]
                          tunnel: w2483 -> [w2488 _]
                          frame False {
                            n907 = Concatenate Strings(w2489, w2488) -> (w2490:string)
                          }
                          frame True {
                          }
                        }
                      }
                    }
                  }
                  n908 = Fract/Exp String To Number(string=w2395) -> (number=w2396:dbl)  [unwired: 3 in, 1 out]
                  n909 = Less Or Equal?(x=w2396, y=100.0) -> (x <= y?=w2387:bool)
                  n910 = Build Array(w2388, w2387) -> (w2382:bool[])
                  n911 = for {
                    tunnel: w2382 -> [w2418] mode=indexing
                    tunnel: string[] ["TA[1] OPERATION FAILED!", "TA[2] OPERATION FAILED!"] -> [w2422] mode=indexing
                    shift-right: [w2424] -> w2384
                    shift-left: "" -> [w2423]
                    tunnel: w2376 -> [w2419]
                    tunnel: [w2419] -> w2375
                    n912 = Concatenate Strings(w2422, "\r\n") -> (w2420:string)
                    n913 = case shown="False" w2418 {
                      tunnel: [w2427 w2428] -> w2424
                      tunnel: w2423 -> [w2426 w2428]
                      tunnel: w2420 -> [w2425 _]
                      frame False {
                        n914 = Concatenate Strings(w2426, w2425) -> (w2427:string)
                      }
                      frame True {
                      }
                    }
                  }
                  n915 = Build Array (concatenate)(w2382, w2381) -> (w2380:bool[])
                  n916 = And Array Elements(Boolean array=w2380) -> (logical AND=w2371:bool)
                  n917 = case shown="False" w2371 {
                    tunnel: w2384 -> [w2416 _]
                    tunnel: w2383 -> [w2415 _]
                    tunnel: w2375 -> [w2413 w2417]
                    tunnel: [w2413 w2417] -> w2373
                    frame False {
                      n918 = Concatenate Strings(w2416, w2415) -> (w2414:string)
                      n919 = One Button Dialog(message=w2414) -> ()  [unwired: 1 in, 1 out]
                    }
                    frame True {
                    }
                  }
                  n920 = case shown="False" w2371 {
                    tunnel: w2373 -> [w2411 w2412]
                    tunnel: [w2410 w2412] -> w2372
                    frame False {
                      n921 = call "Display Message to User6"("error in (no error)"=w2411) -> ("error out"=w2410:errorcluster)  [unwired: 9 in, 1 out]
                    }
                    frame True {
                    }
                  }
                  n922 = Select(t=enum16{"Stop", "Tests", "Bit test", "Start"}."Tests", s=w2371, f=enum16{"Stop", "Tests", "Bit test", "Start"}."Stop") -> (s? t:f=w2377:enum16{"Stop", "Tests", "Bit test", "Start"})
                }
                frame "Start" {
                  n923 = And(x=w2508, y=w2513) -> (x .and. y?=w2509:bool)
                  n924 = case shown="True" w2509 {
                    tunnel: w2520 -> [_ w2547]
                    tunnel: w2519 -> [_ w2538]
                    tunnel: w2518 -> [_ w2534]
                    tunnel: w2517 -> [_ w2532]
                    tunnel: w2516 -> [_ w2531]
                    tunnel: [FALSE w2530] -> w2512
                    tunnel: [w2526 w2529] -> w2507
                    tunnel: [FALSE TRUE] -> w2510
                    frame False {
                      n925 = call "Display Message to User5"() -> ("error out"=w2526:errorcluster)  [unwired: 10 in, 1 out]
                    }
                    frame True {
                      n926 = property on="VISA Tester" class="VISAName"() -> (error out=w2545:errorcluster, "Value"=w2544:refnum<visa-resource-name>)  [unwired: 2 in, 1 out]
                      n927 = call "TesterOption (SubVI).vi"("2 Options"=FALSE, "error in (no error)"=w2545, "On/Off"=FALSE, "Tester Option"=T11."Venable", "VISA Refnum in"=w2544) -> ("error out"=w2540:errorcluster)  [unwired: 5 in, 1 out]
                      n928 = call "Write panel message (SubVI).vi"("Stop BurnIn"=w2532, 4:"rpm"=w2531, 5:"rpm"=FALSE ("rpm"), "PrintTime"=FALSE, "Stop"=w2534, "error in (no error)"=w2540, "Time to wait"=3.0, "Strin"="TESTER BIT TEST OPERATION IN PROCESS\nPlease wait...", "String in"=w2538) -> ("error out"=w2539:errorcluster)  [unwired: 2 in]
                      n929 = property on="UUT SoftwareVer" class="Str"() -> ("Value"=w2528:string)  [unwired: 2 in, 2 out]
                      n930 = call "SerialMarvinSendGet.vi"("error in (no error)"=w2539, "write buffer"="VR\r\n", "VISA resource name"=w2547) -> ("error out"=w2529:errorcluster, "read buffer"=w2546:string)  [unwired: 7 in]
                      n931 = Equal?(x=w2546, y=w2528) -> (x = y?=w2530:bool)
                    }
                  }
                  n932 = case shown="False" w2512 {
                    tunnel: [enum16{"Stop", "Tests", "Bit test", "Start"}."Stop" enum16{"Stop", "Tests", "Bit test", "Start"}."Bit test"] -> w2511
                    tunnel: w2510 -> [w2521 _]
                    frame False {
                      n933 = case shown="True" w2521 {
                        frame False {
                        }
                        frame True {
                          n934 = call "Display Message to User4"() -> ()  [unwired: 10 in, 2 out]
                        }
                      }
                    }
                    frame True {
                    }
                  }
                }
              }
            }
            n935 = Bundle By Name(cluster=T8 {"VISA"="COM1", "Array Test"=[]}, "VISA"=w2210, "Array Test"=w2216) -> (w2212:T8)
            n936 = Enqueue Element(queue=w2218, element=w2212, error in (no error)=w2215) -> (queue out=w2213:refnum<queue>, error out=w2214:errorcluster)  [unwired: 2 out]
          }
          event "Report", "Stop Button": Value Change {
            w2585 = "Marvin" ("section")
            n937 = event-data() -> ("CtlRef"=w2571:refnum<vi>)  [unwired: 1 in]
            n938 = local read "UUT"() -> (w2581:string)
            n939 = call <vilib>:"Application Directory.vi"() -> ("Application Directory"=w2613:path)
            n940 = Build Path(base path=w2613, name or relative path="Reports") -> (appended path=w2616:path)
            n941 = property on="CAN Status" class="Bool (strict)"() -> ("Value"=w2549:bool)  [unwired: 2 in, 2 out]
            n942 = property on="Status" class="Bool (strict)"() -> ("Value"=w2550:bool)  [unwired: 2 in, 2 out]
            n943 = case shown="\"EBAY\", Default" w2581 {
              tunnel: ["REV EBAY" ("key") "REV AHU" ("key")] -> w2583
              frame "EBAY", Default {
              }
              frame "AHU" {
              }
            }
            n944 = call <vilib>:"Check if File or Folder Exists.vi"("path"=w2616) -> ("error out"=w2614:errorcluster, "file or folder exists?"=w2617:bool, "dup path"=w2615:path)  [unwired: 8 in]
            n945 = And(x=w2550, y=w2549) -> (x .and. y?=w2551:bool)
            n946 = case shown="False" w2617 {
              tunnel: w2614 -> [w2683 w2684]
              tunnel: w2615 -> [w2682 w2685]
              tunnel: [w2681 w2685] -> w2622
              tunnel: [w2680 w2684] -> w2619
              frame False {
                n947 = Create Folder(path (use dialog)=w2682, error in=w2683) -> (created path=w2681:path, error out=w2680:errorcluster)  [unwired: 1 in, 1 out]
              }
              frame True {
              }
            }
            n948 = case shown="True" w2551 {
              tunnel: [w2629 w2648] -> w2602
              tunnel: [w2629 w2647] -> w2580
              tunnel: w2575 -> [_ w2635]
              tunnel: [w2629 w2640] -> w2572
              tunnel: [w2629 w2639] -> w2574
              tunnel: [w2629 w2643] -> w2565
              tunnel: [w2629 w2642] -> w2557
              frame False {
                (unwired) "47"
                (unwired) " 413-8005_47_AHU"
                (unwired) "413-8005-1-47"
                (unwired) "5.3.9" ("read buffer")
                (unwired) "95"
                (unwired) "414-8005_95_EBAY_"
                (unwired) "414-8005-95"
                (unwired) "414-8005-95   "
                w2629 = "N_A" ("read buffer")
                n949 = disable-structure shown="Disabled" {
                  frame Disabled {
                    n950 = call "Display Message to User7"() -> ()  [unwired: 10 in, 2 out]
                  }
                  frame Enabled {
                  }
                }
                n951 = Decimal String To Number(string="1" ("Value")) -> (number=w2630:i32)  [unwired: 2 in, 1 out]
                n952 = Number To Decimal String(number=w2630, width (-)=i16 4) -> ()  [unwired: 1 out]
              }
              frame True {
                n953 = call "SerialMarvinSendGet.vi"("write buffer"="SN\r\n", "VISA resource name"=w2635) -> ("error out"=w2634:errorcluster, "read buffer"=w2637:string)  [unwired: 8 in]
                n954 = call "Time Delay2"("error in (no error)"=w2634) -> ("error out"=w2633:errorcluster)  [unwired: 10 in]
                n955 = Decimal String To Number(string=w2637) -> (number=w2636:i32)  [unwired: 2 in, 1 out]
                n956 = Number To Decimal String(number=w2636, width (-)=i16 4) -> (decimal integer string=w2640:string)
                n957 = call "SerialMarvinSendGet.vi"("error in (no error)"=w2633, "write buffer"="VR\r\n", "VISA resource name"=w2635) -> ("error out"=w2644:errorcluster, "read buffer"=w2639:string)  [unwired: 7 in]
                n958 = property on="UUT" class="DigNum (strict)"(error in=w2644) -> ("Value"=w2646:u8)  [unwired: 1 in, 2 out]
                n959 = case shown="95, Default" w2646 {
                  tunnel: ["414-8005_95_EBAY_" " 413-8005_47_AHU" " 413-8005_63_AHU"] -> w2648
                  tunnel: ["414-8005-95   " w2654 w2657] -> w2647
                  tunnel: ["414-8005-95" w2654 w2657] -> w2643
                  tunnel: ["95" "47" "63"] -> w2642
                  frame 95, Default {
                  }
                  frame 47 {
                    w2654 = "413-8005-1-47"
                    (unwired) "AHU-L (47) 413-8005-1"
                  }
                  frame 63 {
                    w2657 = "413-8005-2-63"
                    (unwired) "AHU-R (63) 413-8005-2"
                  }
                }
              }
            }
            n960 = Get Date/Time String(want seconds? (F)=TRUE) -> (date string=w2618:string)  [unwired: 2 in, 1 out]
            n961 = call <vilib>:"Open Config Data.vi"("create file if necessary (T)"=FALSE, "configuration file path"=w2577) -> ("refnum"=w2592:T25)  [unwired: 1 in, 8 out]
            n962 = property on="Logger Path" class="Path"(error in=w2619, "Value"=w2622, "StartPath"=w2622) -> (error out=w2620:errorcluster)  [unwired: 1 in, 1 out]
            n963 = Search and Replace String(replace all?=TRUE ("replace all? (F)"), input string=w2618, search string="/") -> (result string=w2599:string)  [unwired: 5 in, 3 out]
            n964 = call-poly <vilib>:"Read Key.vi"("section"=w2585, "key"=w2583, "refnum"=w2592) -> ("error out"=w2587:errorcluster, "value"=w2590:string, "refnum out"=w2589:T25)  [unwired: 5 in, 1 out]
            n965 = property on="Logger Path" class="Path"(error in=w2620) -> (error out=w2595:errorcluster, "StartPath"=w2598:path)  [unwired: 1 in, 1 out]
            n966 = call-poly <vilib>:"Read Key.vi"("section"=w2585, "error in (no error)"=w2587, "key"="Tester Software Ver", "refnum"=w2589) -> ("error out"=w2584:errorcluster, "value"=w2582:string, "refnum out"=w2588:T25)  [unwired: 4 in, 1 out]
            n967 = Concatenate Strings("ATR" ("string"), w2602, w2572, "_", w2599, ".docx" ("string")) -> (w2596:string)
            n968 = call <vilib>:"Close Config Data.vi"("error in (no error)"=w2584, "refnum"=w2588) -> ()  [unwired: 8 in, 2 out]
            n969 = Build Path(base path=w2598, name or relative path=w2596) -> (appended path=w2597:path)
            n970 = call "HeaderuRayon.vi"("Oper."=w2573, "VR"=w2574, "S/N"=w2572, "UUT"=w2580, "UA"=w2557, "UUTHeader"=w2581, "Tester Software Ver"=w2582) -> ("HEADER1"=w2623:string)  [unwired: 1 in]
            n971 = Concatenate Strings("  Rev-" ("string"), w2590) -> (w2576:string)
            n972 = while {
              tunnel: w2596 -> [w2665]
              tunnel: w2598 -> [w2662]
              shift-right: [w2664] -> w2594
              shift-left: w2597 -> [w2663]
              shift-right: [w2660] -> w2578
              shift-left: w2579 -> [w2661]
              tunnel: w2595 -> [w2666]
              tunnel: [w2667] -> _
              stop <- w2659 continue-if-true
              n973 = call <vilib>:"Check if File or Folder Exists.vi"("error in (no error)"=w2666, "path"=w2663) -> ("error out"=w2667:errorcluster, "file or folder exists?"=w2659:bool)  [unwired: 7 in, 1 out]
              n974 = case shown="True" w2659 {
                tunnel: w2665 -> [_ w2679]
                tunnel: w2661 -> [_ w2671]
                tunnel: [w2669 w2676] -> w2664
                tunnel: w2663 -> [w2669 _]
                tunnel: w2662 -> [_ w2677]
                tunnel: [1 w2670] -> w2660
                frame False {
                }
                frame True {
                  w2672 = ".docx" ("search string")
                  n975 = Search and Replace String(input string=w2679, search string=w2672) -> (result string=w2678:string)  [unwired: 6 in, 3 out]
                  n976 = Number To Decimal String(number=w2671) -> (decimal integer string=w2674:string)  [unwired: 1 in]
                  n977 = call <vilib>:"Space Constant.vi"() -> ("String"=w2673:string)
                  n978 = Concatenate Strings(w2678, w2673, w2674, w2672) -> (w2675:string)
                  n979 = Build Path(base path=w2677, name or relative path=w2675) -> (appended path=w2676:path)
                  n980 = Increment(x=w2671) -> (x+1=w2670:i32)
                }
              }
            }
            n981 = Open/Create/Replace File(file path (use dialog)=w2594, operation (0:open)=T24."create") -> (error out=w2608:errorcluster)  [unwired: 4 in, 2 out]
            n982 = control-ref of="ATR"() -> (w2624:refnum<vi>)
            n983 = property class="Tbl (strict)"(reference=w2624, error in=w2608) -> ("Value"=w2625:string[][])  [unwired: 2 out]
            n984 = call "MarvinReport.vi"("HEADER1"=w2623, "ATR Or"=w2624, "Steps   pfull"=w2625, "Footer UUT"=w2565, "pageNum"=3, "FILE NAME"=w2596, "Report Folder"=w2594, "REV"=w2576, "Test-Conductor"=w2573) -> ("error out"=w2560:errorcluster)  [unwired: 5 in, 1 out]
            n985 = call <vilib>:"Clear Errors.vi"("error in (no error)"=w2560) -> ("error out"=w2559:errorcluster)  [unwired: 5 in, 1 out]
            n986 = property class="Bool (strict)"(reference=w2571, error in=w2559) -> ("BoolText.Text"=w2570:string)  [unwired: 2 out]
            n987 = Equal?(x=w2570, y="Report") -> (x = y?=w2564:bool)
            n988 = Select(t=T10."MainProgram", s=w2564, f=T10."Stop") -> (s? t:f=w2567:T10)
            n989 = Select(t="Save Report...", s=w2564, f="Program Stopped...\r\nPlease turn OFF All Power sinks") -> (s? t:f=w2562:string)
            n990 = property on="Report" class="Bool (strict)"(error in=w2559, "Value"=FALSE ("Report")) -> (error out=w2552:errorcluster)  [unwired: 1 in, 1 out]
            n991 = property on="VISA Tester" class="VISAName"() -> ("Value"=w2556:refnum<visa-resource-name>)  [unwired: 2 in, 2 out]
            n992 = property on="Pannel User Message" class="Str"("Value"=w2562) -> ()  [unwired: 2 in, 2 out]
            n993 = call "TesterOption (SubVI).vi"("2 Options"=FALSE, "error in (no error)"=w2552, "On/Off"=FALSE, "Tester Option"=T11."Venable", "VISA Refnum in"=w2556) -> ()  [unwired: 5 in, 2 out]
          }
          event "Help Button": Value Change {
            n994 = event-data() -> ()  [unwired: 1 in, 6 out]
            n995 = vi-ref "Help.vi"() -> (w2695:refnum<vi>)
            n996 = invoke class="VI" method="FP.Open"(reference=w2695, error in=w2693, "Activate"=TRUE ("Activate?"), "State"=T21."Standard") -> (error out=w2694:errorcluster)  [unwired: 1 in, 4 out]
            n997 = call "Help.vi"("error in"=w2694) -> ("error out"=w2692:errorcluster)  [unwired: 7 in]
          }
          event "Serial Com": Value Change {
            n998 = event-data() -> ()  [unwired: 1 in, 6 out]
            n999 = property on="Serial Com" class="Bool"(error in=w2704, "Visible"=FALSE) -> (error out=w2708:errorcluster)  [unwired: 1 in, 1 out]
            n1000 = property on="VISA Marvin" class="VISAName"(error in=w2708, "Visible"=TRUE) -> (error out=w2705:errorcluster)  [unwired: 1 in, 1 out]
          }
          event "VISA Marvin": Value Change {
            n1001 = event-data() -> ()  [unwired: 1 in, 6 out]
            n1002 = property on="Serial Com" class="Bool"(error in=w2711, "Visible"=FALSE) -> (error out=w2710:errorcluster)  [unwired: 1 in, 1 out]
            n1003 = control-ref of="This VI"() -> (w2722:refnum<vi>)
            n1004 = property on="Pannel User Message" class="Str"(error in=w2711, "Value"="Serial connection in process" ("Pannel User Message")) -> ()  [unwired: 1 in, 2 out]
            n1005 = call "Serial InitMarvin.vi"("error in (no error)"=w2710, "VI reference (current VI)"=w2722, "VISA Refnum in"="VISA Marvin") -> ("error out"=w2714:errorcluster, "Boolean"=w2712:bool)  [unwired: 7 in]
            n1006 = property on="VISA Marvin" class="VISAName"(error in=w2714, "Visible"=FALSE) -> (error out=w2725:errorcluster)  [unwired: 1 in, 1 out]
            n1007 = property on="Serial Com" class="Bool"(error in=w2725, "Visible"=TRUE) -> (error out=w2721:errorcluster)  [unwired: 1 in, 1 out]
            n1008 = case shown="True" w2712 {
              tunnel: w2721 -> [w2728 w2740]
              tunnel: "VISA Marvin" -> [w2729 w2737]
              tunnel: [w2729 w2736] -> w2716
              tunnel: [w2728 w2735] -> w2715
              frame False {
              }
              frame True {
                n1009 = call "SerialMarvinSendGet.vi"("error in (no error)"=w2740, "Clear Log"=FALSE, "write buffer"="VC\r\n", "VISA resource name"=w2737) -> ("error out"=w2739:errorcluster, "read buffer"=w2733:string)  [unwired: 6 in]
                n1010 = Decimal String To Number(string=w2733) -> (number=w2732:i32)  [unwired: 2 in, 1 out]
                n1011 = Less Or Equal?(x=w2732, y=50) -> (x <= y?=w2730:bool)
                n1012 = property on="Status" class="Bool (strict)"("Value"=w2730) -> ()  [unwired: 2 in, 2 out]
                n1013 = case shown="True" w2730 {
                  tunnel: w2739 -> [w2741 w2765]
                  tunnel: w2737 -> [w2742 w2764]
                  tunnel: [w2742 w2755] -> w2736
                  tunnel: [w2741 w2749] -> w2735
                  frame False {
                  }
                  frame True {
                    n1014 = call <vilib>:"Clear Errors.vi"("error in (no error)"=w2765) -> ("error out"=w2766:errorcluster)  [unwired: 5 in, 1 out]
                    n1015 = control-ref of="ATR"() -> (w2752:refnum<vi>)
                    n1016 = VISA Flush I/O Buffer(VISA resource name=w2764, error in (no error)=w2766) -> (VISA resource name out=w2755:refnum<visa-resource-name>, error out=w2763:errorcluster)  [unwired: 1 in]
                    n1017 = call "Display Message to User2"("error in (no error)"=w2763) -> ("error out"=w2762:errorcluster, "Yes"=w2761:bool)  [unwired: 9 in]
                    n1018 = case shown="True" w2761 {
                      tunnel: w2762 -> [w2767 w2789]
                      tunnel: [w2767 w2768] -> w2760
                      tunnel: w2755 -> [_ w2786]
                      frame False {
                      }
                      frame True {
                        w2774 = FALSE ("2 Options")
                        n1019 = property on="UUT" class="DigNum (strict)"() -> ("Value"=w2788:u8)  [unwired: 2 in, 2 out]
                        n1020 = call "SetParam.vi"("RS"=TRUE, "error in (no error)"=w2789, "Param to Set in"=w2788, "Visa"=w2786) -> ("error out"=w2769:errorcluster)  [unwired: 7 in]
                        n1021 = control-ref of="Pannel User Message"() -> (w2785:refnum<vi>)
                        n1022 = control-ref of="Stop Burn-in"() -> (w2783:refnum<vi>)
                        n1023 = control-ref of="Stop Button"() -> (w2784:refnum<vi>)
                        n1024 = control-ref of="Motor Speed RPM"() -> (w2782:refnum<vi>)
                        n1025 = property on="VISA Tester" class="VISAName"() -> ("Value"=w2778:refnum<visa-resource-name>)  [unwired: 2 in, 2 out]
                        n1026 = call "TesterOption (SubVI).vi"("2 Options"=w2774, "error in (no error)"=w2769, "On/Off"=FALSE, "Tester Option"=T11."Power", "VISA Refnum in"=w2778) -> ("error out"=w2779:errorcluster, "VISA Refnum out"=w2781:refnum<visa-resource-name>)  [unwired: 5 in]
                        n1027 = call "Write panel message (SubVI).vi"("Stop BurnIn"=w2783, "rpm"=w2782, "PrintTime"=TRUE, "Stop"=w2784, "error in (no error)"=w2779, "Time to wait"=20.0, "Strin"="Restart the UUT\nPlease wait...", "String in"=w2785) -> ("error out"=w2780:errorcluster)  [unwired: 3 in]
                        n1028 = call "TesterOption (SubVI).vi"("2 Options"=w2774, "error in (no error)"=w2780, "On/Off"=FALSE, "Tester Option"=T11."Venable", "VISA Refnum in"=w2781) -> ("error out"=w2768:errorcluster)  [unwired: 5 in, 1 out]
                      }
                    }
                    n1029 = call "Find_Number_LineMARVIN.vi"("Test Paragraph"="2.1", "TableIn"=w2752) -> ("Line number"=w2753:i32)  [unwired: 3 in, 3 out]
                    n1030 = call "SerialMarvinSendGet.vi"("error in (no error)"=w2760, "write buffer"="SN\r\n", "VISA resource name"=w2755) -> ("error out"=w2756:errorcluster, "read buffer"=w2744:string)  [unwired: 7 in]
                    n1031 = call "SerialMarvinSendGet.vi"("error in (no error)"=w2756, "write buffer"="AO[1]\r\n", "VISA resource name"=w2755) -> ("error out"=w2750:errorcluster, "read buffer"=w2751:string)  [unwired: 7 in]
                    n1032 = Fract/Exp String To Number(string=w2751) -> (number=w2746:dbl)  [unwired: 3 in, 1 out]
                    n1033 = In Range and Coerce(upper limit=0.1 ("x"), x=w2746, lower limit=-0.1) -> (In Range?=w2745:bool)  [unwired: 1 out]
                    n1034 = call "PassOrFail (SubVI).vi"("Test#"="2", "index (row)"=w2753, "error in (no error)"=w2750, "Data in"=w2746, "Pass?Fail"=w2745, "Table in"=w2752) -> ("error out"=w2749:errorcluster)  [unwired: 5 in]
                    n1035 = property on="UUT SN Report" class="Str"("Value"=w2744) -> ()  [unwired: 2 in, 2 out]
                    n1036 = Decimal String To Number(string=w2744) -> (number=→"Current SN":i32)  [unwired: 2 in, 1 out]
                  }
                }
              }
            }
          }
          event "Refresh Button": Value Change {
            n1037 = event-data() -> ()  [unwired: 1 in, 6 out]
          }
          event "Settings": Value Change {
            n1038 = event-data() -> ()  [unwired: 1 in, 6 out]
            n1039 = control-ref of="VISA Tester"() -> (w2799:refnum<vi>)
            n1040 = control-ref of="UUT"() -> (w2797:refnum<vi>)
            n1041 = property on="Status" class="Bool (strict)"() -> ("Value"=w2801:bool)  [unwired: 2 in, 2 out]
            n1042 = case shown="True" w2801 {
              tunnel: w2807 -> [_ w2819]
              tunnel: [w2808 w2814] -> w2802
              tunnel: w2800 -> [_ w2813]
              tunnel: w2799 -> [_ w2812]
              tunnel: w2798 -> [_ w2811]
              tunnel: w2797 -> [_ w2810]
              frame False {
                n1043 = call "Display Message to User8"() -> ("error out"=w2808:errorcluster)  [unwired: 10 in, 1 out]
              }
              frame True {
                n1044 = vi-ref "Calibration (SubVI).vi"() -> (w2818:refnum<vi>)
                n1045 = invoke class="VI" method="FP.Open"(reference=w2818, error in=w2819, "Activate"=TRUE ("Activate?"), "State"=T21."Standard") -> (error out=w2815:errorcluster)  [unwired: 1 in, 4 out]
                n1046 = call "Calibration (SubVI).vi"("VISA UUT"=w2813, "error constant"=w2815, "UUT"=w2810, "CAN Cluster in"=w2811, "Visa Tester"=w2812) -> ("error constant 2"=w2814:errorcluster, "AO[1]Meas"=→"Cal":dbl)  [unwired: 5 in]
              }
            }
          }
        }
      }
      frame "Initialize" {
        w2823 = FALSE ("Visible")
        w2824 = FALSE ("Visible")
        w2825 = FALSE ("Visible")
        w2826 = FALSE ("Visible")
        w2838 = refnum<visa-resource-name> "COM1" ("VISA resource name")
        w2828 = FALSE ("Visible")
        w2821 = FALSE ("Serial Status")
        n1047 = property on="ComTestResult" class="Bool (strict)"("Value"=w2826) -> ()  [unwired: 2 in, 2 out]
        n1048 = property on="VenableResult" class="Bool (strict)"("Value"=w2826) -> ()  [unwired: 2 in, 2 out]
        n1049 = property on="VenableDirectionResult" class="Bool (strict)"("Value"=w2826) -> ()  [unwired: 2 in, 2 out]
        n1050 = property on="SpeedResult" class="Bool (strict)"("Value"=w2826) -> ()  [unwired: 2 in, 2 out]
        n1051 = property on="Serial Com" class="Bool"(error in=errorcluster {"status"=FALSE, "code"=0, "source"=""} ("error out"), "Visible"=TRUE) -> (error out=w2840:errorcluster)  [unwired: 1 in, 1 out]
        n1052 = property on="AuxiOFFResult" class="Bool (strict)"("Value"=w2825) -> ()  [unwired: 2 in, 2 out]
        n1053 = property on="AuxiONResult" class="Bool (strict)"("Value"=w2825) -> ()  [unwired: 2 in, 2 out]
        n1054 = property on="VisualInspectionResult" class="Bool (strict)"("Value"=w2825) -> ()  [unwired: 2 in, 2 out]
        n1055 = property on="SensCalResult" class="Bool (strict)"("Value"=w2825) -> ()  [unwired: 2 in, 2 out]
        n1056 = property on="VISA Marvin" class="VISAName"(error in=w2840, "Visible"=w2828, "Value"=w2838) -> (error out=w2829:errorcluster)  [unwired: 1 in, 1 out]
        n1057 = property on="Stop Burn-in" class="Bool (strict)"(error in=w2829, "Visible"=w2828) -> (error out=w2822:errorcluster)  [unwired: 1 in, 1 out]
        n1058 = property on="BurnDC" class="Bool (strict)"("Value"=w2824) -> ()  [unwired: 2 in, 2 out]
        n1059 = property on="BurnTemp" class="Bool (strict)"("Value"=w2824) -> ()  [unwired: 2 in, 2 out]
        n1060 = property on="BurnSpeed" class="Bool (strict)"("Value"=w2824) -> ()  [unwired: 2 in, 2 out]
        n1061 = property on="BurnResult" class="Bool (strict)"("Value"=w2824) -> ()  [unwired: 2 in, 2 out]
        n1062 = property on="Refresh Button" class="Bool (strict)"(error in=w2822, "Value"=FALSE ("Refresh Button")) -> ()  [unwired: 1 in, 2 out]
        n1063 = property on="StopTimeResult" class="Bool (strict)"("Value"=w2823) -> ()  [unwired: 2 in, 2 out]
        n1064 = property on="MotorTempResult" class="Bool (strict)"("Value"=w2823) -> ()  [unwired: 2 in, 2 out]
        n1065 = property on="TempControlResult" class="Bool (strict)"("Value"=w2823) -> ()  [unwired: 2 in, 2 out]
        n1066 = property on="Automation" class="Bool (strict)"("Value"=w2823) -> ()  [unwired: 2 in, 2 out]
        n1067 = flat-sequence {
          tunnel: w2822 -> [w2843]
          tunnel: [w2842] -> w2836
          tunnel: [w2846] -> w2835
          tunnel: w2836 -> [w2846]
          tunnel: [w2858] -> w2834
          tunnel: w2835 -> [w2859]
          tunnel: [w2859] -> w2833
          frame #0 {
            n1068 = control-ref of="This VI"() -> (w2844:refnum<vi>)
            n1069 = invoke class="VI" method="Default Vals.Reinit All"(reference=w2844, error in=w2843) -> (error out=w2842:errorcluster)  [unwired: 1 in, 2 out]
          }
          frame #1 {
            w2849 = u32 4294967295  # AccMask
            w2845 = T4 0 items=["使用Flash参数", "使用界面设置参数"] ("InitFlag")
            w2847 = T6 0 items=["normal operation", "Listen-only mode", "test mode"]  # Mode
            w2848 = T5 3 items=["接收所有类型"=1, "只接收标准帧"=2, "只接收扩展帧"=3] ("Fliter")
            w2853 = u8 10 items=["5k bps"=1, "10k bps"=2, "20k bps"=3, "40k bps"=4, "50k bps"=5, "80k bps"=6, "100k bps"=7, "125k bps"=8, "200k bps"=9, "250k bps"=10, "400k bps"=11, "500k bps"=12, "666k bps"=13, "800k bps"=14, "1000k bps"=15, "33.33k bps"=16, "66.66k bps"=17, "83.33k bps"=18]  # kBaudRate
            w2850 = u32 0  # AccCode
            w2851 = T2 4 items=["USB-CAN"=3, "USB-CAN2"=4] ("DevType")
            w2852 = T7 {"DevType"=3, "DevIndex"=0, "CanIndex"=0, "VCI_INIT_CONFIG"={"AccCode"=0, "AccMask"=0, "InitFlag"=1, "Fliter"=7, "Timing0"=0, "Timing1"=0, "Mode"=0}}  # Config
            # "CANalystII"
            n1070 = call "Demo_GetT0T1.vi"("kBaudRate"=w2853) -> ("Timing0"=w2855:u8, "Timing1"=w2856:u8)
            n1071 = Bundle By Name(cluster=w2852, "DevType"=w2851, "CanIndex"="Channel 2", "VCI_INIT_CONFIG.AccCode"=w2850, "VCI_INIT_CONFIG.AccMask"=w2849, "VCI_INIT_CONFIG.InitFlag"=w2845, "VCI_INIT_CONFIG.Fliter"=w2848, "VCI_INIT_CONFIG.Timing0"=w2855, "VCI_INIT_CONFIG.Timing1"=w2856, "VCI_INIT_CONFIG.Mode"=w2847) -> (→"Config_CANAT":T7)
          }
          frame #2 {
            w2860 = u16 284 items=["1M"=20, "500K"=28, "250K"=284, "125K"=796, "100K"=17199, "50K"=18223, "20K"=21295, "10K"=26415, "5K"=32639] ("baud in")
            n1072 = control-ref of="Config_CANAT"() -> (w2858:refnum<vi>)
            n1073 = call "InitCAN_ATII.vi"("Config"=w2858) -> ("Sts"=→"CAN Status":bool)
            n1074 = call "ChangeCANBaud.vi"("baud in"=w2860, "reference"=w2858) -> ()
          }
        }
        "Status" <- w2821
        "Test Failed" <- w2821
      }
    }
  }
  n1075 = property on="Settings" class="Bool (strict)"("Visible"=w4) -> ()  [unwired: 2 in, 2 out]
  n1076 = property on="Cal" class="DigNum (strict)"("Visible"=w4) -> ()  [unwired: 2 in, 2 out]
  n1077 = disable-structure shown="Disabled" {
    frame Disabled {
      w2862 = T19."Disabled and Grayed Out" ("Disabled")
      w2863 = FALSE ("Start")
      n1078 = property on="VISA Tester" class="VISAName" props=["Value"]() -> ()  [unwired: 2 in, 3 out]
      n1079 = property on="Current SN" class="DigNum (strict)" props=["Value"]() -> ()  [unwired: 2 in, 3 out]
      n1080 = property on="UUT" class="DigNum (strict)" props=["Value"]() -> ()  [unwired: 2 in, 3 out]
      n1081 = property on="Status" class="Bool (strict)" props=["Value"]() -> ()  [unwired: 2 in, 3 out]
      n1082 = property on="UUT SoftwareVer" class="Str" props=["Value"]() -> ()  [unwired: 2 in, 3 out]
      n1083 = property on="Next SN" class="DigNum (strict)" props=["Value"]() -> ()  [unwired: 3 in, 2 out]
      n1084 = property on="Start" class="Bool (strict)"("Value"=w2863, "DisabledEnum"=w2862) -> ()  [unwired: 2 in, 2 out]
      n1085 = property on="Report" class="Bool (strict)"("Value"=w2863, "DisabledEnum"=w2862) -> ()  [unwired: 2 in, 2 out]
    }
    frame Enabled {
    }
  }
  n1086 = disable-structure shown="Disabled" {
    frame Disabled {
      (unwired) 0.02003173828125 ("x")
      n1087 = control-ref of="Stop Burn-in"() -> ()  [unwired: 1 out]
      n1088 = control-ref of="Stop Button"() -> ()  [unwired: 1 out]
      n1089 = control-ref of="Motor Speed RPM"() -> ()  [unwired: 1 out]
      n1090 = control-ref of="Config_CANAT"() -> ()  [unwired: 1 out]
      n1091 = control-ref of="UUT"() -> ()  [unwired: 1 out]
      n1092 = call "GetADCTester (SubVI).vi"() -> ()  [unwired: 9 in, 3 out]
      n1093 = call "CANSendMotorSpeed.vi"() -> ()  [unwired: 11 in, 1 out]
      n1094 = control-ref of="Config_CANAT"() -> ()  [unwired: 1 out]
      n1095 = call "Find_Number_LineMARVIN.vi"() -> ()  [unwired: 5 in, 4 out]
      n1096 = property on="UUT" class="DigNum (strict)" props=["Value"]() -> ()  [unwired: 2 in, 3 out]
      n1097 = control-ref of="UUT"() -> ()  [unwired: 1 out]
      n1098 = call "DegToDAC (SubVI).vi"() -> ()  [unwired: 10 in, 2 out]
      n1099 = call "Write panel message (SubVI).vi"() -> ()  [unwired: 11 in, 1 out]
      n1100 = property on="VISA Tester" class="VISAName" props=["Value"]() -> ()  [unwired: 2 in, 3 out]
      n1101 = control-ref of="ATR"() -> ()  [unwired: 1 out]
      n1102 = call "TesterOption (SubVI).vi"() -> ()  [unwired: 10 in, 2 out]
      n1103 = call "TesterOption (SubVI).vi"() -> ()  [unwired: 10 in, 2 out]
      n1104 = call "PassOrFail (SubVI).vi"() -> ()  [unwired: 11 in, 1 out]
    }
    frame Enabled {
    }
  }
  n1105 = disable-structure shown="Disabled" {
    frame Disabled {
      n1106 = flat-sequence {
        frame #0 {
          n1107 = call "CANSendMotorSpeed.vi"("Remote"=TRUE, "Motor Speed RPM"=u16 0) -> ("error out"=w2865:errorcluster, "UUT"=w2868:refnum<vi>)  [unwired: 8 in]
          n1108 = property on="VISA Tester" class="VISAName"() -> ("Value"=w2864:refnum<visa-resource-name>)  [unwired: 2 in, 2 out]
          n1109 = call "TesterOption (SubVI).vi"("error in (no error)"=w2865, "On/Off"=FALSE, "Tester Option"=T11."Power", "VISA Refnum in"=w2864) -> ()  [unwired: 6 in, 2 out]
        }
      }
    }
    frame Enabled {
    }
  }
  "Pannel User Message" <- w2
